vi "Lab Panel V2.6.vi"() -> ()   [LabVIEW 2013]
uses:
  <vilib>/Platform/TimedLoop/XDataNode/timing_clust.ctl
  <vilib>/Platform/TimedLoop/XDataNode/nitl_modes.ctl
  <vilib>/Platform/TimedLoop/XDataNode/wakeup.ctl
  <vilib>/platform/TimedLoop/XDataNode/XDataNode.xnode
  <vilib>/Platform/TimedLoop/XDataNode/XDNodeRunTimeDep.lvlib
panel:
  out "TEMP update":bool
  out "AI update":bool
  in  "stop":bool
  in  "Tab Control 2":T1(tab)
  out "LAB05-2 (SIG)":T2 {"PF" format="%.2f"; "AMPS" format="%.1f"}
  out "LAB05-1 (SIG)":T2 {"PF" format="%.2f"; "AMPS" format="%.1f"}
  out "LAB04-2 (SIG)":T2 {"PF" format="%.2f"; "AMPS" format="%.1f"}
  out "LAB04-1 (SIG)":T2 {"PF" format="%.2f"; "AMPS" format="%.1f"}
  out "LAB03-2 (SIG)":T2 {"PF" format="%.2f"; "AMPS" format="%.1f"}
  out "LAB03-1 (SIG)":T2 {"PF" format="%.2f"; "AMPS" format="%.1f"}
  out "LAB02-2 (SIG)":T2 {"PF" format="%.2f"; "AMPS" format="%.1f"}
  in  "LAB01-1RUN":bool
  in  "LAB05-1 (O/I)":bool
  in  "LAB05-2 (O/I)":bool
  in  "LAB04-1 (O/I)":bool
  in  "LAB04-2 (O/I)":bool
  in  "LAB02-1 (O/I)":bool
  in  "LAB02-2 (O/I)":bool
  in  "LAB01-2 (O/I)":bool
  in  "LAB01-1 (O/I)":bool
  in  "LAB03-1 (O/I)":bool
  in  "LAB05-2 RUN":bool
  in  "LAB05-1 RUN":bool
  in  "LAB04-2 RUN":bool
  in  "LAB04-1 RUN":bool
  in  "LAB03-2 RUN":bool
  in  "LAB03-1 RUN":bool
  in  "LAB02-2 RUN":bool
  in  "LAB02-1 RUN":bool
  in  "LAB01-2 RUN":bool
  in  "LAB05-2 SELECT":T3(radio)
  in  "LAB05-1 SELECT":T3(radio)
  in  "LAB04-2 SELECT":T3(radio)
  in  "LAB04-1 SELECT":T3(radio)
  in  "LAB03-2 SELECT":T3(radio)
  in  "LAB03-1 SELECT":T3(radio)
  in  "LAB02-2 SELECT":T3(radio)
  in  "LAB02-1 SELECT":T3(radio)
  in  "LAB01-2 SELECT":T3(radio)
  in  "LAB01-1 SELECT":T3(radio)
  in  "LAB03-2 (O/I)":bool
  out "LAB01-1 (SIG)":T2 {"PF" format="%.2f"; "AMPS" format="%.1f"}
  out "LAB01-2 (SIG)":T2 {"PF" format="%.2f"; "AMPS" format="%.1f"}
  out "LAB02-1 (SIG)":T2 {"PF" format="%.2f"; "AMPS" format="%.1f"}
  out "LAB05-2 (DISP)":T4 {"MINS" format="%.2g"}
  out "LAB05-1 (DISP)":T4 {"MINS" format="%.2g"}
  out "LAB04-2 (DISP)":T4 {"MINS" format="%.2g"}
  out "LAB04-1 (DISP)":T4 {"MINS" format="%.2g"}
  out "LAB03-2 (DISP)":T4 {"MINS" format="%.2g"}
  out "LAB03-1 (DISP)":T4 {"MINS" format="%.2g"}
  in  "LAB05-2 (SET)":T5
  in  "LAB05-1 (SET)":T5
  in  "LAB04-2 (SET)":T5
  in  "LAB04-1 (SET)":T5
  in  "LAB03-2 (SET)":T5
  in  "LAB03-1 (SET)":T5
  out "LAB02-2 (DISP)":T4 {"MINS" format="%.2g"}
  out "LAB02-1 (DISP)":T4 {"MINS" format="%.2g"}
  in  "LAB02-2 (SET)":T5
  in  "LAB02-1 (SET)":T5
  out "LAB05-2 (RESULT)":bool
  out "LAB05-1 (RESULT)":bool
  out "LAB04-2 (RESULT)":bool
  out "LAB04-1 (RESULT)":bool
  out "LAB03-2 (RESULT)":bool
  out "LAB03-1 (RESULT)":bool
  out "LAB02-2 (RESULT)":bool
  out "LAB02-1 (RESULT)":bool
  out "LAB01-2 (RESULT)":bool
  out "LAB01-1 (RESULT)":bool
  in  "LAB01-1 (SET)":T5
  in  "LAB01-2(SET)":T5
  out "LAB01-1 (DISP)":T4 {"MINS" format="%.2g"}
  out "LAB01-2 (DISP)":T4 {"MINS" format="%.2f"}
  out "LAB05-2 (TEMP START)":cluster{"TL":dbl, "TN":dbl}
  out "LAB04-2 (TEMP START)":cluster{"TL":dbl, "TN":dbl}
  out "LAB03-2 (TEMP START)":cluster{"TL":dbl, "TN":dbl}
  out "LAB02-2 (TEMP START)":cluster{"TL":dbl, "TN":dbl}
  out "LAB01-2 (TEMP START)":cluster{"TL":dbl, "TN":dbl}
  out "LAB05-1 (TEMP START)":cluster{"TL":dbl, "TN":dbl}
  out "LAB04-1 (TEMP START)":cluster{"TL":dbl, "TN":dbl}
  out "LAB03-1 (TEMP START)":cluster{"TL":dbl, "TN":dbl}
  out "LAB02-1 (TEMP START)":cluster{"TL":dbl, "TN":dbl}
  out "LAB01-1 (TEMP START)":cluster{"TL":dbl, "TN":dbl}
  in  "JIG ON TIME (S)":dbl=1.0 min=1.0 max=10.0 step=0.5 format="%.1g"
  in  "JIG OFF TIME (S)":dbl=2.0 min=2.0 max=10.0 step=0.5 format="%.1g"
  out "LAB01-1 (JIG)":bool
  out "LAB01-2 (JIG)":bool
  out "LAB02-1 (JIG)":bool
  out "LAB02-2 (JIG)":bool
  out "LAB03-1 (JIG)":bool
  out "LAB03-2 (JIG)":bool
  out "LAB04-1 (JIG)":bool
  out "LAB04-2 (JIG)":bool
  out "LAB05-1 (JIG)":bool
  out "LAB05-2 (JIG)":bool
  out "LAB01 (CAL)":T6 {"2 (TN) cal" min=0.0 step=0.01 format="%.2f"; "2 (TL) cal" min=0.0 step=0.01 format="%.2f"; "2 (PF) cal" min=0.0 step=0.01 format="%.2f"; "2 (V) cal" min=0.0 step=0.01 format="%.2f"; "2 (A) cal" min=0.0 step=0.01 format="%.2f"; "1 (TN) cal" min=0.0 step=0.01 format="%.2f"; "1 (TL) cal" min=0.0 step=0.01 format="%.2f"; "1 (PF) cal" min=0.0 step=0.01 format="%.2f"; "1 (V) cal" min=0.0 step=0.01 format="%.2f"; "1  (A) cal" min=0.0 step=0.01 format="%.2f"}
  out "LAB03 (CAL)":T6 {"2 (TN) cal" min=0.0 step=0.01 format="%.2f"; "2 (TL) cal" min=0.0 step=0.01 format="%.2f"; "2 (PF) cal" min=0.0 step=0.01 format="%.2f"; "2 (V) cal" min=0.0 step=0.01 format="%.2f"; "2 (A) cal" min=0.0 step=0.01 format="%.2f"; "1 (TN) cal" min=0.0 step=0.01 format="%.2f"; "1 (TL) cal" min=0.0 step=0.01 format="%.2f"; "1 (PF) cal" min=0.0 step=0.01 format="%.2f"; "1 (V) cal" min=0.0 step=0.01 format="%.2f"; "1  (A) cal" min=0.0 step=0.01 format="%.2f"}
  out "LAB02 (CAL)":T7 {"2 (TN) cal" min=0.0 step=0.01 format="%.2f"; "2 (TL) cal" min=0.0 step=0.01 format="%.2f"; "2 (PF) cal" min=0.0 step=0.01 format="%.2f"; "2 (V) cal" min=0.0 step=0.01 format="%.2f"; "2 (A) cal" min=0.0 step=0.01 format="%.2f"; "1 (TN) cal" min=0.0 step=0.01 format="%.2f"; "1 (TL) cal" min=0.0 step=0.01 format="%.2f"; "1 (PF) cal" min=0.0 step=0.01 format="%.2f"; "1 (V) cal" min=0.0 step=0.01 format="%.2f"; "1 (A) cal" min=0.0 step=0.01 format="%.2f"}
  out "LAB05 (CAL)":T6 {"2 (TN) cal" min=0.0 step=0.01 format="%.2f"; "2 (TL) cal" min=0.0 step=0.01 format="%.2f"; "2 (PF) cal" min=0.0 step=0.01 format="%.2f"; "2 (V) cal" min=0.0 step=0.01 format="%.2f"; "2 (A) cal" min=0.0 step=0.01 format="%.2f"; "1 (TN) cal" min=0.0 step=0.01 format="%.2f"; "1 (TL) cal" min=0.0 step=0.01 format="%.2f"; "1 (PF) cal" min=0.0 step=0.01 format="%.2f"; "1 (V) cal" min=0.0 step=0.01 format="%.2f"; "1  (A) cal" min=0.0 step=0.01 format="%.2f"}
  out "LAB04 (CAL)":T6 {"2 (TN) cal" min=0.0 step=0.01 format="%.2f"; "2 (TL) cal" min=0.0 step=0.01 format="%.2f"; "2 (PF) cal" min=0.0 step=0.01 format="%.2f"; "2 (V) cal" min=0.0 step=0.01 format="%.2f"; "2 (A) cal" min=0.0 step=0.01 format="%.2f"; "1 (TN) cal" min=0.0 step=0.01 format="%.2f"; "1 (TL) cal" min=0.0 step=0.01 format="%.2f"; "1 (PF) cal" min=0.0 step=0.01 format="%.2f"; "1 (V) cal" min=0.0 step=0.01 format="%.2f"; "1  (A) cal" min=0.0 step=0.01 format="%.2f"}
  out "calibration file error out":errorcluster
  in  "CALIBRATE":bool
  in  "Amps fail level":dbl=1.0 min=1.0 max=100.0 step=1.0
  in  "Tab Control":T8(tab)
  out "LAB01-2 (GRAPH)":dynamicdata(graph)
  out "LAB01-1 (GRAPH)":dynamicdata(graph)
  out "LAB02-2 (GRAPH)":dynamicdata(graph)
  out "LAB02-1 (GRAPH)":dynamicdata(graph)
  out "LAB03-2 (GRAPH)":dynamicdata(graph)
  out "LAB03-1 (GRAPH)":dynamicdata(graph)
  out "LAB04-2 (GRAPH)":dynamicdata(graph)
  out "LAB04-1 (GRAPH)":dynamicdata(graph)
  out "LAB05-2 (GRAPH)":dynamicdata(graph)
  out "LAB05-1 (GRAPH)":dynamicdata(graph)
  out "LAB05 TEMP":T9
  out "LAB04 TEMP":T9
  out "LAB02 TEMP":T9
  out "LAB01 TEMP":T9
  out "LAB03 TEMP":T9
  out "Analog Error Array":errorcluster[](array[cluster])
  out "AI loop time":dbl format="%.6g"
  out "loops":dbl
  in  "loop  delay(mS)":dbl
  out "on loops":dbl
  out "off loops":dbl
  out "jig cycle":dbl
  out "LAB01-1 (TDMS)":refnum<k34>
  out "data file error":errorcluster
  out "LAB02-1 (TDMS)":refnum<k34>
  out "LAB01-2 (TDMS)":refnum<k34>
  out "LAB02-2 (TDMS)":refnum<k34>
  out "LAB03-1 (TDMS)":refnum<k34>
  out "LAB03-2 (TDMS)":refnum<k34>
  out "LAB04-1 (TDMS)":refnum<k34>
  out "LAB04-2 (TDMS)":refnum<k34>
  out "LAB05-1 (TDMS)":refnum<k34>
  out "LAB05-2 (TDMS)":refnum<k34>
  # "LAB01"
  # "LAB02"
  # "LAB05"
  # "LAB03"
  # "LAB04"
  # "LAB01"
  # "LAB02"
  # "LAB03"
  # "LAB04"
  # "LAB05"
  # "JIG SET"
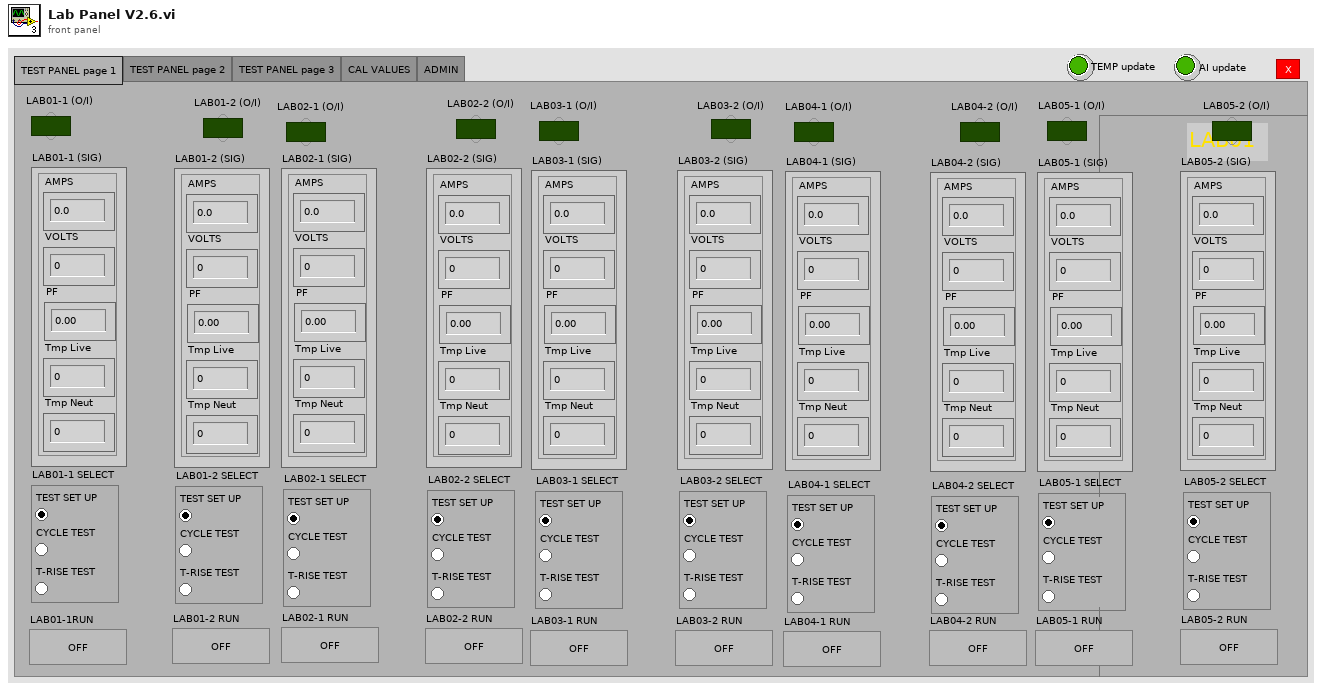
[diagram p1: front panel]
types:
  T1 = enum32{"TEST PANEL page 1", "TEST PANEL page 2", "TEST PANEL page 3", "CAL VALUES", "ADMIN"}
  T2 = cluster{"AMPS":dbl, "VOLTS":dbl, "PF":dbl, "Tmp Live":dbl, "Tmp Neut":dbl}
  T3 = enum32{"TEST SET UP", "CYCLE TEST", "T-RISE TEST"}
  T4 = cluster{"CYCLE":dbl, "MINS":dbl, "STATUS":string}
  T5 = cluster{"NAME":string, "DESCRIPTION":string, "CYCLES":dbl, "T-RISE mins":dbl, "T-RISE deg C":dbl}
  T6 = cluster{"1  (A) cal":dbl, "1 (V) cal":dbl, "1 (PF) cal":dbl, "1 (TL) cal":dbl, "1 (TN) cal":dbl, "2 (A) cal":dbl, "2 (V) cal":dbl, "2 (PF) cal":dbl, "2 (TL) cal":dbl, "2 (TN) cal":dbl}
  T7 = cluster{"1 (A) cal":dbl, "1 (V) cal":dbl, "1 (PF) cal":dbl, "1 (TL) cal":dbl, "1 (TN) cal":dbl, "2 (A) cal":dbl, "2 (V) cal":dbl, "2 (PF) cal":dbl, "2 (TL) cal":dbl, "2 (TN) cal":dbl}
  T8 = enum32{"LAB01", "LAB02", "LAB03", "LAB04", "LAB05", "TEMPERATURE", "ERROR"}
  T9 = cluster{"T1 Live":dbl, "T1 Neut":dbl, "T2 Live":dbl, "T2 Neut":dbl, "ID":dbl, "ER":dbl}
  T10 = typedef "XDNodeRunTimeDep.lvlib/timing_clust.ctl" = cluster{"Expected End [f-1]":u64, "Actual End [f-1]":u64, "Finished Late? [f-1]":bool, "Expected End [i-1]":u64, "Actual End [i-1]":u64, "Finished Late? [i-1]":bool, "Expected Start [i]":u64, "Actual Start [i]":u64, "Expected Start [f]":u64, "Actual Start [f]":u64, "Source Name":string, "Structure Name":string, "Period":i64, "Deadline":i64, "Offset":i64, "Start":i64, "Priority":i32, "Timeout":i32, "Mode":T11, "Wakeup Reason":T12, "Error":errorcluster, "Source Type":string, "Secondary Source Type":string, "Global End Time":u64, "Global Start Time":u64, "Frame Duration":u64, "Iteration Duration":u64, "Assigned CPU":i32, "I/O Scan Engine Mode":u32}
  T11 = typedef "XDNodeRunTimeDep.lvlib/nitl_modes.ctl" = enum32{"No Change", "Process missed periods, maintain original phase", "Discard missed periods, maintain original phase", "Process missed periods, ignore original phase", "Discard missed periods, ignore original phase"}
  T12 = typedef "XDNodeRunTimeDep.lvlib/wakeup.ctl" = enum32{"Normal", "Aborted", "Asynchronous wakeup", "Timing source error", "Timed loop error", "Timeout"}
  T13 = enum16{"open", "open or create", "create or replace", "create", "open (read-only)"}
  T14 = cluster{"T1":dbl, "T2":dbl, "T3":dbl, "T4":dbl, "ID":dbl, "ER":dbl}
  T15 = cluster{"LAB01-1 (A)":dbl, "LAB01-1 (V)":dbl, "LAB01-1 (PF)":dbl, "LAB01-2 (A)":dbl, "LAB01-2 (V)":dbl, "LAB01-2 (PF)":dbl}
  T16 = cluster{"LAB02-1 (A)":dbl, "LAB02-1 (V)":dbl, "LAB02-1 (PF)":dbl, "LAB02-2 (A)":dbl, "LAB02-2 (V)":dbl, "LAB02-2 (PF)":dbl}
  T17 = cluster{"LAB03-1 (A)":dbl, "LAB03-1 (V)":dbl, "LAB03-1 (PF)":dbl, "LAB03-2 (A)":dbl, "LAB03-2 (V)":dbl, "LAB03-2 (PF)":dbl}
  T18 = cluster{"LAB04-1 (A)":dbl, "LAB04-1 (V)":dbl, "LAB04-1 (PF)":dbl, "LAB04-2 (A)":dbl, "LAB04-2 (V)":dbl, "LAB04-2 (PF)":dbl}
  T19 = cluster{"LAB05-1 (A)":dbl, "LAB05-1 (V)":dbl, "LAB05-1 (PF)":dbl, "LAB05-2 (A)":dbl, "LAB05-2 (V)":dbl, "LAB05-2 (PF)":dbl}
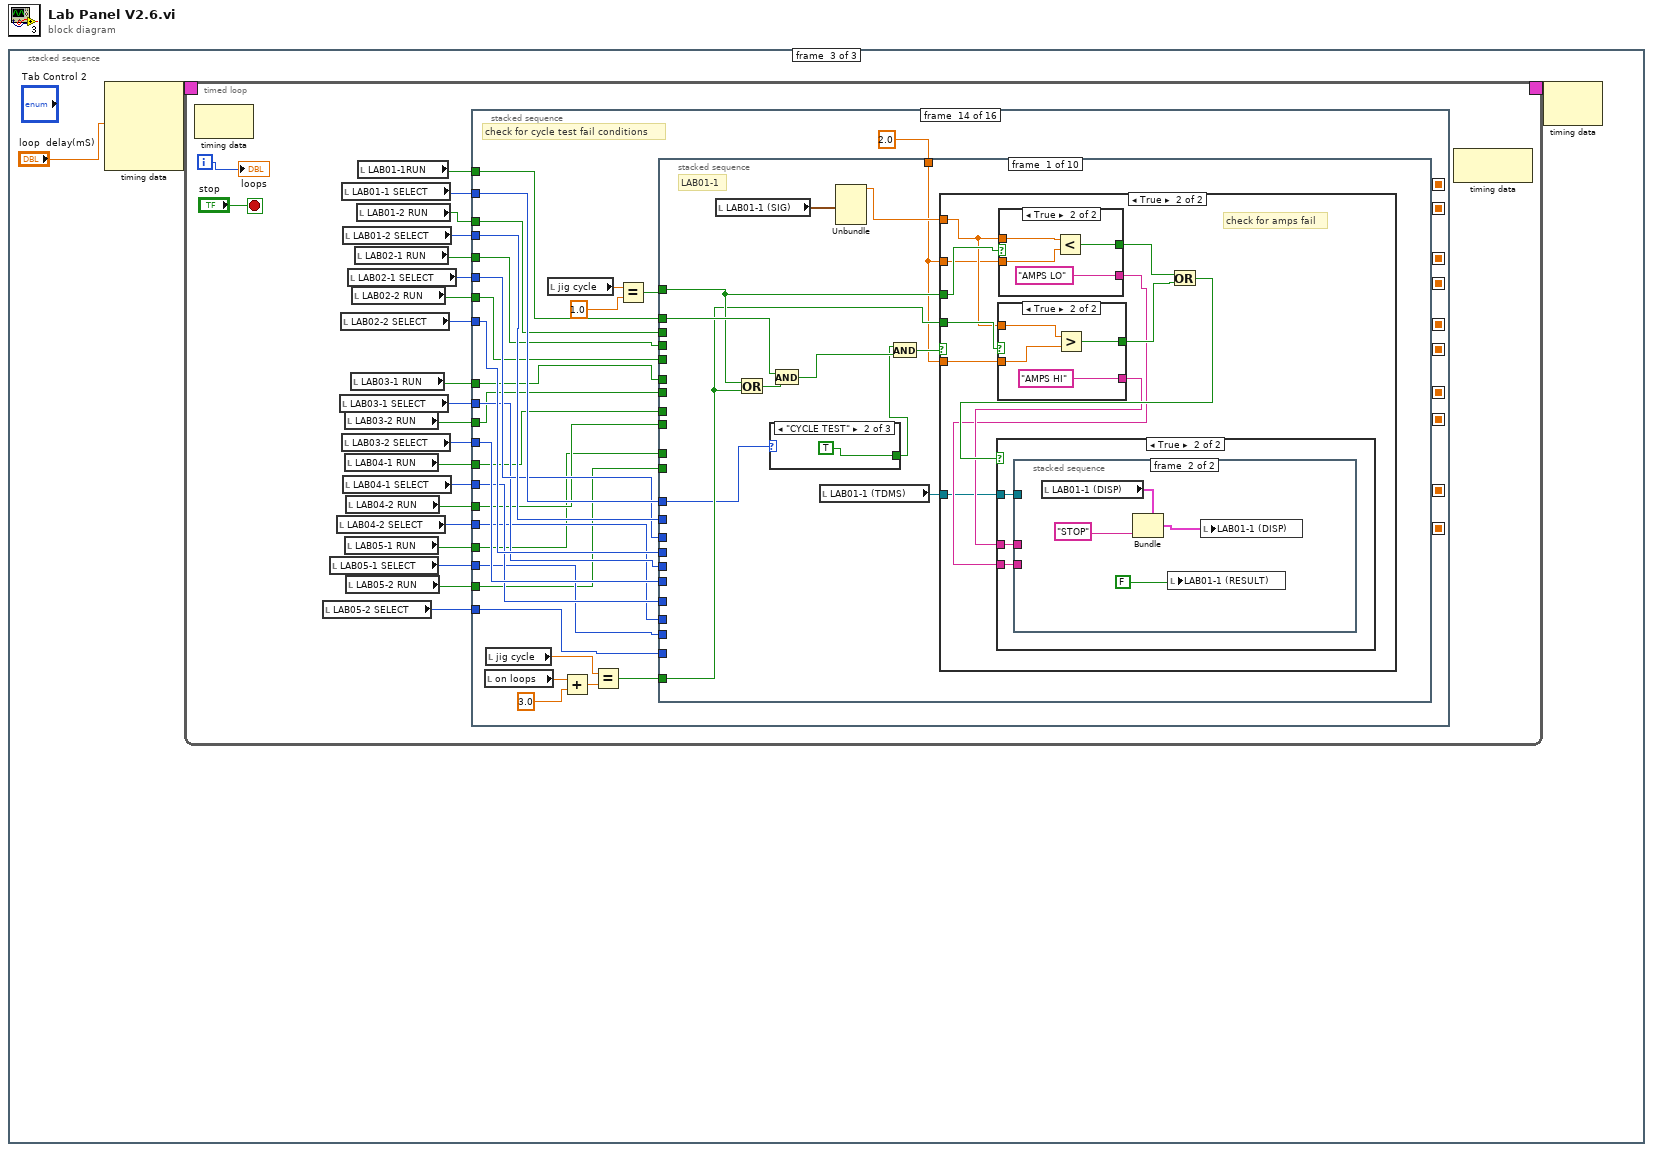
[diagram p0: block diagram]
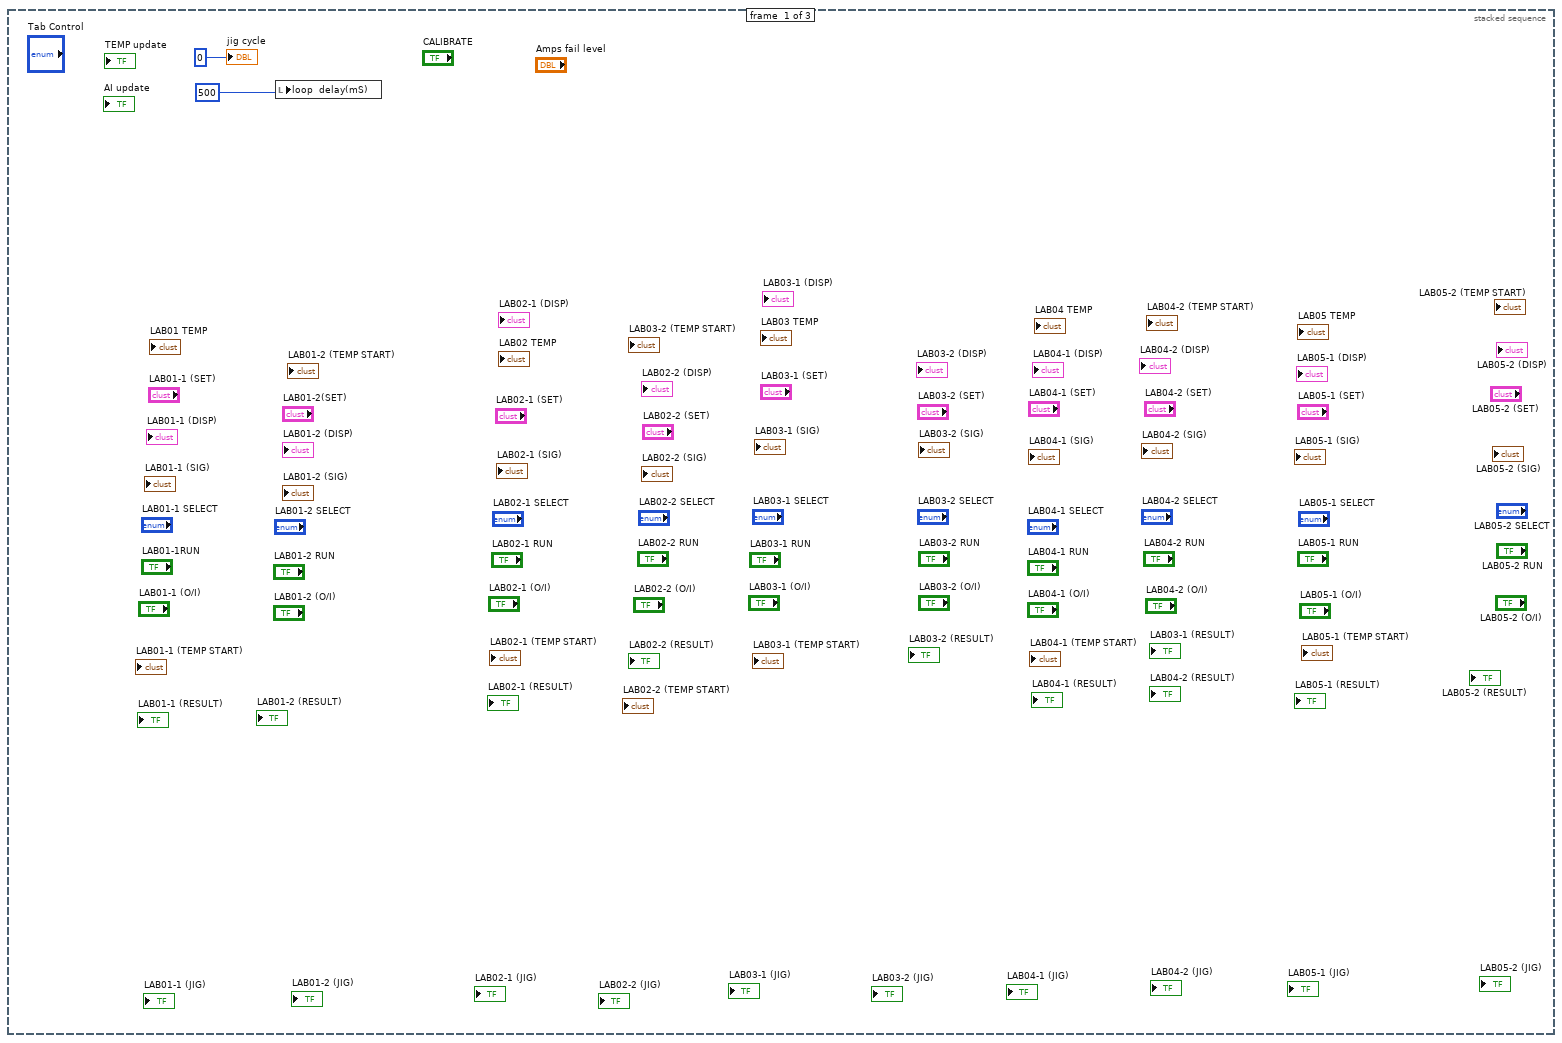
[diagram p2: hidden frame]
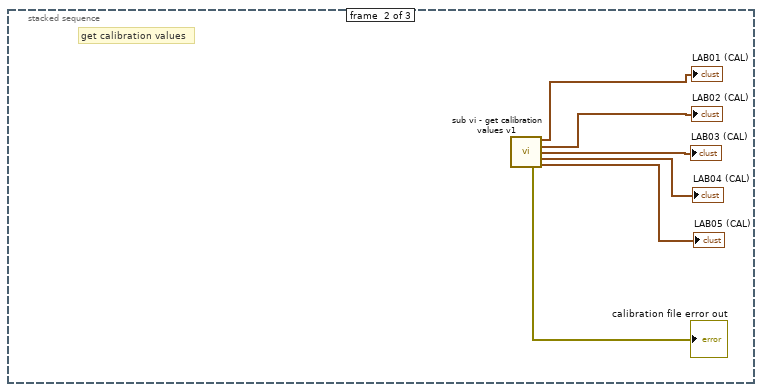
[diagram p3: hidden frame]
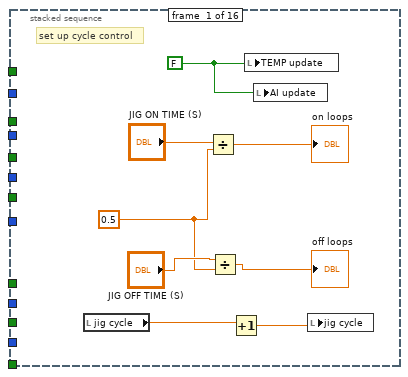
[diagram p4: hidden frame]
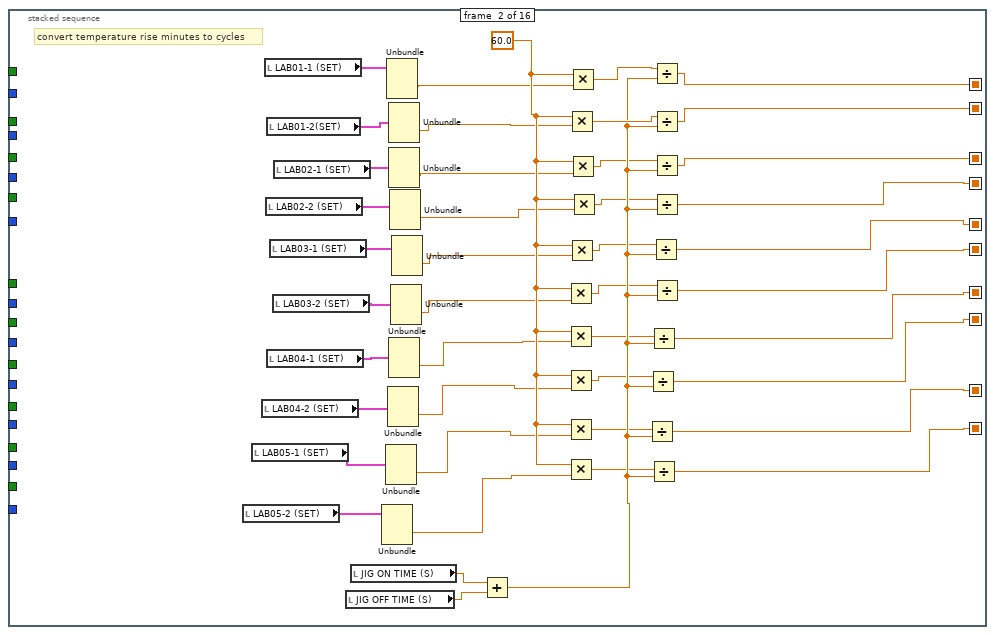
[diagram p5: hidden frame]
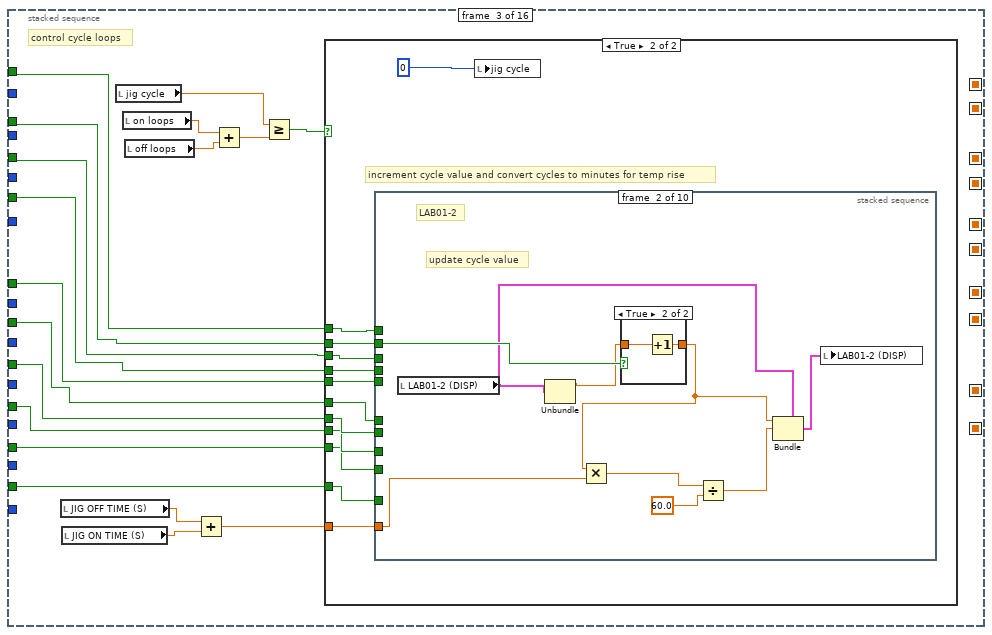
[diagram p6: hidden frame]
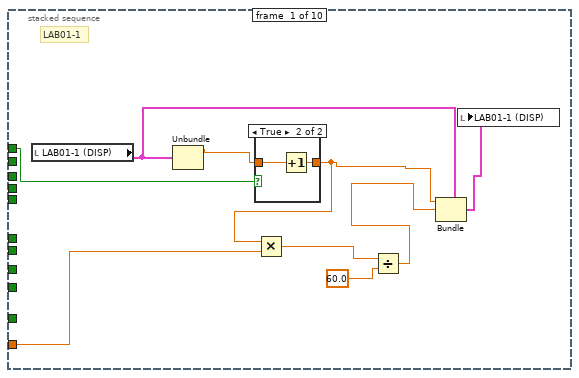
[diagram p8: hidden frame]
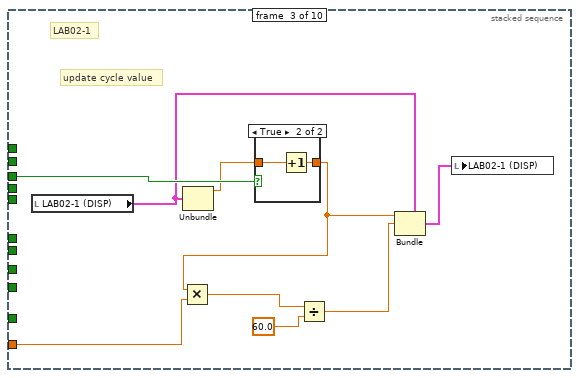
[diagram p11: hidden frame]
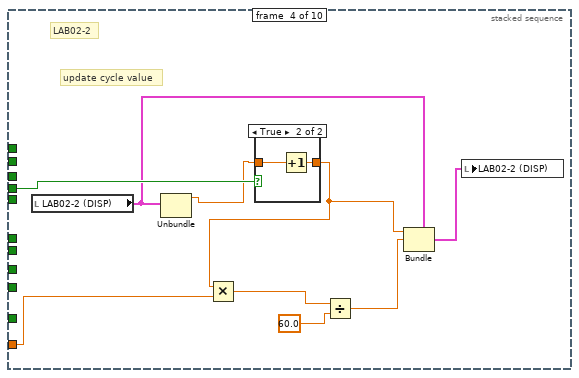
[diagram p13: hidden frame]
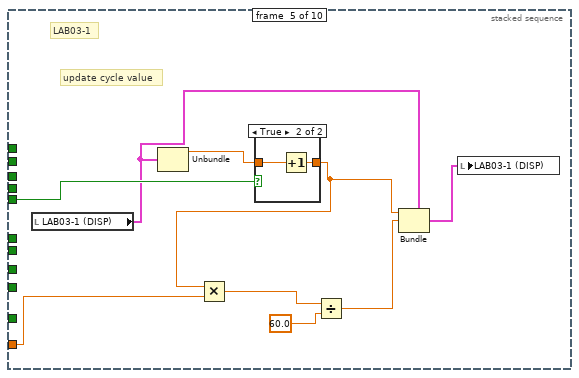
[diagram p15: hidden frame]
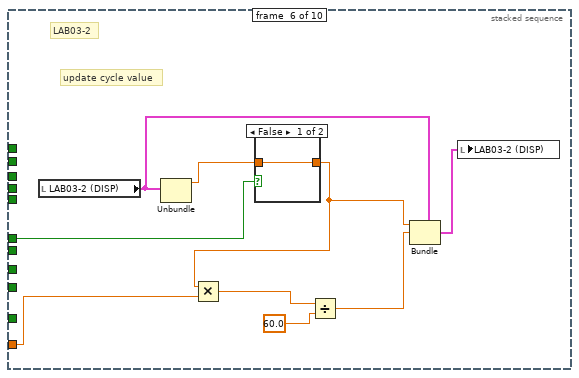
[diagram p17: hidden frame]
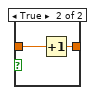
[diagram p18: hidden frame]
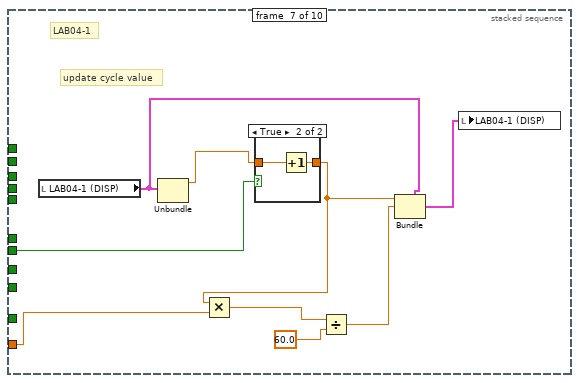
[diagram p19: hidden frame]
diagram:
  n1 = stacked-sequence {
    frame #0 {
      n2 = local write "loop  delay(mS)"(500) -> ()
      "jig cycle" <- 0
    }
    frame #1 {
      # "get calibration values"
      n3 = call "sub vi - get calibration values v1.vi"() -> ("LAB01 (CAL)"=→"LAB01 (CAL)":T6, "LAB02 (CAL)"=→"LAB02 (CAL)":T7, "LAB03 (CAL)"=→"LAB03 (CAL)":T6, "LAB04 (CAL)"=→"LAB04 (CAL)":T6, "calibration file error out"=→"calibration file error out":errorcluster, "LAB05 (CAL)"=→"LAB05 (CAL)":T6)  [unwired: 10 in]
    }
    frame #2 {
      n4 = node-c288("loop  delay(mS)") -> (w11:T10)  [unwired: 3 in]
      n5 = timed-loop {
        timing: w11 -> [_]
        timing-out: [_] -> w10
        i -> [w33]
        stop <- "stop" stop-if-true
        n6 = node-c288() -> ()  [unwired: 1 in, 1 out]
        n7 = local read "LAB05-2 SELECT"() -> (w12:T3)
        n8 = local read "LAB05-1 SELECT"() -> (w13:T3)
        n9 = local read "LAB04-2 SELECT"() -> (w14:T3)
        n10 = local read "LAB03-1 SELECT"() -> (w17:T3)
        n11 = local read "LAB02-2 SELECT"() -> (w18:T3)
        n12 = local read "LAB01-1 SELECT"() -> (w21:T3)
        n13 = local read "LAB03-2 SELECT"() -> (w16:T3)
        n14 = local read "LAB01-2 SELECT"() -> (w20:T3)
        n15 = local read "LAB04-1 SELECT"() -> (w15:T3)
        n16 = local read "LAB03-2 RUN"() -> (w26:bool)
        n17 = local read "LAB04-1 RUN"() -> (w25:bool)
        n18 = local read "LAB05-1 RUN"() -> (w23:bool)
        n19 = local read "LAB04-2 RUN"() -> (w24:bool)
        n20 = local read "LAB05-2 RUN"() -> (w22:bool)
        n21 = local read "LAB02-1 SELECT"() -> (w19:T3)
        n22 = local read "LAB03-1 RUN"() -> (w27:bool)
        n23 = local read "LAB02-2 RUN"() -> (w28:bool)
        n24 = local read "LAB02-1 RUN"() -> (w29:bool)
        n25 = local read "LAB01-2 RUN"() -> (w30:bool)
        n26 = local read "LAB01-1RUN"() -> (w31:bool)
        n27 = stacked-sequence {
          seq-local: [_ w85 _ _ _ _ _ _ _ _ _ _ _ _ _ _] -> [_ _ _ _ _ w1464 _ _ _ _ _ _ _ _ _ _]
          seq-local: [_ w84 _ _ _ _ _ _ _ _ _ _ _ _ _ _] -> [_ _ _ _ _ _ _ _ _ _ _ _ _ _ _ _]
          seq-local: [_ w71 _ _ _ _ _ _ _ _ _ _ _ _ _ _] -> [_ _ _ _ _ _ _ _ _ _ _ _ _ _ _ _]
          seq-local: [_ w70 _ _ _ _ _ _ _ _ _ _ _ _ _ _] -> [_ _ _ _ _ _ _ _ _ _ _ _ _ _ _ _]
          seq-local: [_ w69 _ _ _ _ _ _ _ _ _ _ _ _ _ _] -> [_ _ _ _ _ _ _ _ _ _ _ _ _ _ _ _]
          seq-local: [_ w68 _ _ _ _ _ _ _ _ _ _ _ _ _ _] -> [_ _ _ _ _ _ _ _ _ _ _ _ _ _ _ _]
          seq-local: [_ w67 _ _ _ _ _ _ _ _ _ _ _ _ _ _] -> [_ _ _ _ _ _ _ _ _ _ _ _ _ _ _ _]
          seq-local: [_ w66 _ _ _ _ _ _ _ _ _ _ _ _ _ _] -> [_ _ _ _ _ _ _ _ _ _ _ _ _ _ _ _]
          seq-local: [_ w65 _ _ _ _ _ _ _ _ _ _ _ _ _ _] -> [_ _ _ _ _ _ _ _ _ _ _ _ _ _ _ _]
          seq-local: [_ w64 _ _ _ _ _ _ _ _ _ _ _ _ _ _] -> [_ _ _ _ _ _ _ _ _ _ _ _ _ _ _ _]
          tunnel: w31 -> [_ _ w101 w257 w1064 w1475 w1785 _ _ _ _ _ w2350 w2839 w3378 _]
          tunnel: w30 -> [_ _ w100 w255 w1063 w1474 w1784 _ _ _ _ _ w2349 w2837 w3368 _]
          tunnel: w29 -> [_ _ w99 w253 w1062 w1473 w1783 _ _ _ _ _ w2348 w2835 w3367 _]
          tunnel: w28 -> [_ _ w98 w251 w1061 w1472 w1782 _ _ _ _ _ w2347 w2833 w3366 _]
          tunnel: w27 -> [_ _ w97 w249 w1060 w1471 w1781 _ _ _ _ _ w2346 w2831 w3365 _]
          tunnel: w26 -> [_ _ w96 w247 w1059 w1470 w1780 _ _ _ _ _ w2345 w2829 w3364 _]
          tunnel: w25 -> [_ _ w95 w245 w1058 w1469 w1779 _ _ _ _ _ w2344 w2827 w3360 _]
          tunnel: w24 -> [_ _ w94 w243 w1057 w1468 w1778 _ _ _ _ _ w2343 w2825 w3363 _]
          tunnel: w23 -> [_ _ w93 w241 w1056 w1467 w1777 _ _ _ _ _ w2342 w2823 w3362 _]
          tunnel: w22 -> [_ _ w92 w239 w1055 w1466 w1776 _ _ _ _ _ w2341 w2821 w3361 _]
          tunnel: w21 -> [_ _ _ w256 w1054 w1465 _ _ _ _ _ _ _ w2841 w3379 _]
          tunnel: w20 -> [_ _ _ w254 w1053 w1463 _ _ _ _ _ _ _ w2836 w3377 _]
          tunnel: w19 -> [_ _ _ w252 w1052 w1462 _ _ _ _ _ _ _ w2834 w3376 _]
          tunnel: w18 -> [_ _ _ w250 w1051 w1461 _ _ _ _ _ _ _ w2832 w3375 _]
          tunnel: w17 -> [_ _ _ w248 w1050 w1460 _ _ _ _ _ _ _ w2830 w3374 _]
          tunnel: w16 -> [_ _ _ w246 w1049 w1459 _ _ _ _ _ _ _ w2828 w3373 _]
          tunnel: w15 -> [_ _ _ w244 w1048 w1458 _ _ _ _ _ _ _ w2826 w3372 _]
          tunnel: w14 -> [_ _ _ w242 w1047 w1457 _ _ _ _ _ _ _ w2824 w3371 _]
          tunnel: w13 -> [_ _ _ w240 w1046 w1456 _ _ _ _ _ _ _ w2822 w3370 _]
          tunnel: w12 -> [_ _ _ w238 w1045 w1455 _ _ _ _ _ _ _ w2820 w3369 _]
          frame #0 {
            w36 = FALSE
            w41 = 0.5
            # "set up cycle control"
            n28 = local read "jig cycle"() -> (w40:dbl)
            n29 = Divide(x="JIG ON TIME (S)", y=w41) -> (x/y=→"on loops":dbl)
            n30 = Divide(x="JIG OFF TIME (S)", y=w41) -> (x/y=→"off loops":dbl)
            n31 = Increment(x=w40) -> (x+1=w39:dbl)
            n32 = local write "TEMP update"(w36) -> ()
            n33 = local write "AI update"(w36) -> ()
            n34 = local write "jig cycle"(w39) -> ()
          }
          frame #1 {
            w81 = 60.0
            # "convert temperature rise minutes to cycles"
            n35 = local read "LAB05-2 (SET)"() -> (w45:T5)
            n36 = local read "LAB05-1 (SET)"() -> (w47:T5)
            n37 = local read "LAB04-2 (SET)"() -> (w49:T5)
            n38 = local read "LAB01-1 (SET)"() -> (w63:T5)
            n39 = local read "LAB02-2 (SET)"() -> (w57:T5)
            n40 = local read "LAB01-2(SET)"() -> (w61:T5)
            n41 = local read "LAB04-1 (SET)"() -> (w51:T5)
            n42 = local read "LAB03-1 (SET)"() -> (w55:T5)
            n43 = local read "LAB03-2 (SET)"() -> (w53:T5)
            n44 = local read "LAB02-1 (SET)"() -> (w59:T5)
            n45 = local read "JIG OFF TIME (S)"() -> (w86:dbl)
            n46 = local read "JIG ON TIME (S)"() -> (w87:dbl)
            n47 = Unbundle(w45) -> ("T-RISE mins"=w44:dbl)  [unwired: 4 out]
            n48 = Unbundle(w47) -> ("T-RISE mins"=w46:dbl)  [unwired: 4 out]
            n49 = Unbundle(w63) -> ("T-RISE mins"=w62:dbl)  [unwired: 4 out]
            n50 = Unbundle(w49) -> ("T-RISE mins"=w48:dbl)  [unwired: 4 out]
            n51 = Unbundle(w61) -> ("T-RISE mins"=w60:dbl)  [unwired: 4 out]
            n52 = Unbundle(w59) -> ("T-RISE mins"=w58:dbl)  [unwired: 4 out]
            n53 = Unbundle(w51) -> ("T-RISE mins"=w50:dbl)  [unwired: 4 out]
            n54 = Unbundle(w57) -> ("T-RISE mins"=w56:dbl)  [unwired: 4 out]
            n55 = Unbundle(w53) -> ("T-RISE mins"=w52:dbl)  [unwired: 4 out]
            n56 = Unbundle(w55) -> ("T-RISE mins"=w54:dbl)  [unwired: 4 out]
            n57 = Add(x=w87, y=w86) -> (x+y=w80:dbl)
            n58 = Multiply(x=w81, y=w52) -> (x*y=w76:dbl)
            n59 = Multiply(x=w81, y=w50) -> (x*y=w75:dbl)
            n60 = Multiply(x=w81, y=w48) -> (x*y=w74:dbl)
            n61 = Multiply(x=w81, y=w46) -> (x*y=w73:dbl)
            n62 = Multiply(x=w81, y=w44) -> (x*y=w72:dbl)
            n63 = Multiply(x=w81, y=w60) -> (x*y=w82:dbl)
            n64 = Multiply(x=w81, y=w54) -> (x*y=w77:dbl)
            n65 = Multiply(x=w81, y=w62) -> (x*y=w83:dbl)
            n66 = Multiply(x=w81, y=w58) -> (x*y=w79:dbl)
            n67 = Multiply(x=w81, y=w56) -> (x*y=w78:dbl)
            n68 = Divide(x=w73, y=w80) -> (x/y=w65:dbl)
            n69 = Divide(x=w74, y=w80) -> (x/y=w66:dbl)
            n70 = Divide(x=w75, y=w80) -> (x/y=w67:dbl)
            n71 = Divide(x=w72, y=w80) -> (x/y=w64:dbl)
            n72 = Divide(x=w77, y=w80) -> (x/y=w69:dbl)
            n73 = Divide(x=w83, y=w80) -> (x/y=w85:dbl)
            n74 = Divide(x=w82, y=w80) -> (x/y=w84:dbl)
            n75 = Divide(x=w79, y=w80) -> (x/y=w71:dbl)
            n76 = Divide(x=w78, y=w80) -> (x/y=w70:dbl)
            n77 = Divide(x=w76, y=w80) -> (x/y=w68:dbl)
          }
          frame #2 {
            # "control cycle loops"
            n78 = local read "JIG OFF TIME (S)"() -> (w90:dbl)
            n79 = local read "JIG ON TIME (S)"() -> (w89:dbl)
            n80 = local read "jig cycle"() -> (w103:dbl)
            n81 = local read "on loops"() -> (w105:dbl)
            n82 = local read "off loops"() -> (w104:dbl)
            n83 = Add(x=w90, y=w89) -> (x+y=w88:dbl)
            n84 = Add(x=w105, y=w104) -> (x+y=w91:dbl)
            n85 = Greater Or Equal?(x=w103, y=w91) -> (x >= y?=w102:bool)
            n86 = case shown="True" w102 {
              tunnel: w101 -> [_ w116]
              tunnel: w100 -> [_ w115]
              tunnel: w99 -> [_ w114]
              tunnel: w98 -> [_ w113]
              tunnel: w97 -> [_ w112]
              tunnel: w96 -> [_ w111]
              tunnel: w95 -> [_ w110]
              tunnel: w94 -> [_ w109]
              tunnel: w93 -> [_ w108]
              tunnel: w92 -> [_ w107]
              tunnel: w88 -> [_ w106]
              frame False {
              }
              frame True {
                # "increment cycle value and convert cycles to minutes for temp rise"
                n87 = stacked-sequence {
                  tunnel: w116 -> [w126 _ _ _ _ _ _ _ _ _]
                  tunnel: w115 -> [_ w138 _ _ _ _ _ _ _ _]
                  tunnel: w114 -> [_ _ w150 _ _ _ _ _ _ _]
                  tunnel: w113 -> [_ _ _ w162 _ _ _ _ _ _]
                  tunnel: w112 -> [_ _ _ _ w174 _ _ _ _ _]
                  tunnel: w111 -> [_ _ _ _ _ w186 _ _ _ _]
                  tunnel: w110 -> [_ _ _ _ _ _ w198 _ _ _]
                  tunnel: w109 -> [_ _ _ _ _ _ _ w210 _ _]
                  tunnel: w108 -> [_ _ _ _ _ _ _ _ w222 _]
                  tunnel: w107 -> [_ _ _ _ _ _ _ _ _ w234]
                  tunnel: w106 -> [w123 w135 w147 w159 w171 w183 w195 w207 w219 w231]
                  frame #0 {
                    # "LAB01-1"
                    n88 = local read "LAB01-1 (DISP)"() -> (w121:T4)
                    n89 = Unbundle(w121) -> ("CYCLE"=w122:dbl)  [unwired: 2 out]
                    n90 = case shown="True" w126 {
                      tunnel: w122 -> [w127 w129]
                      tunnel: [w127 w128] -> w120
                      frame False {
                      }
                      frame True {
                        n91 = Increment(x=w129) -> (x+1=w128:dbl)
                      }
                    }
                    n92 = Multiply(x=w120, y=w123) -> (x*y=w124:dbl)
                    n93 = Divide(x=w124, y=60.0) -> (x/y=w119:dbl)
                    n94 = Bundle(cluster=w121, "CYCLE"=w120, "MINS"=w119) -> (w118:T4)  [unwired: 1 in]
                    n95 = local write "LAB01-1 (DISP)"(w118) -> ()
                  }
                  frame #1 {
                    # "update cycle value"
                    # "LAB01-2"
                    n96 = local read "LAB01-2 (DISP)"() -> (w133:T4)
                    n97 = Unbundle(w133) -> ("CYCLE"=w134:dbl)  [unwired: 2 out]
                    n98 = case shown="True" w138 {
                      tunnel: w134 -> [w139 w141]
                      tunnel: [w139 w140] -> w131
                      frame False {
                      }
                      frame True {
                        n99 = Increment(x=w141) -> (x+1=w140:dbl)
                      }
                    }
                    n100 = Multiply(x=w131, y=w135) -> (x*y=w136:dbl)
                    n101 = Divide(x=w136, y=60.0) -> (x/y=w130:dbl)
                    n102 = Bundle(cluster=w133, "CYCLE"=w131, "MINS"=w130) -> (w132:T4)  [unwired: 1 in]
                    n103 = local write "LAB01-2 (DISP)"(w132) -> ()
                  }
                  frame #2 {
                    # "update cycle value"
                    # "LAB02-1"
                    n104 = local read "LAB02-1 (DISP)"() -> (w145:T4)
                    n105 = Unbundle(w145) -> ("CYCLE"=w146:dbl)  [unwired: 2 out]
                    n106 = case shown="True" w150 {
                      tunnel: [w151 w153] -> w143
                      tunnel: w146 -> [w151 w152]
                      frame False {
                      }
                      frame True {
                        n107 = Increment(x=w152) -> (x+1=w153:dbl)
                      }
                    }
                    n108 = Multiply(x=w143, y=w147) -> (x*y=w148:dbl)
                    n109 = Divide(x=w148, y=60.0) -> (x/y=w142:dbl)
                    n110 = Bundle(cluster=w145, "CYCLE"=w143, "MINS"=w142) -> (w144:T4)  [unwired: 1 in]
                    n111 = local write "LAB02-1 (DISP)"(w144) -> ()
                  }
                  frame #3 {
                    # "update cycle value"
                    # "LAB02-2"
                    n112 = local read "LAB02-2 (DISP)"() -> (w157:T4)
                    n113 = Unbundle(w157) -> ("CYCLE"=w158:dbl)  [unwired: 2 out]
                    n114 = case shown="True" w162 {
                      tunnel: [w163 w165] -> w156
                      tunnel: w158 -> [w163 w164]
                      frame False {
                      }
                      frame True {
                        n115 = Increment(x=w164) -> (x+1=w165:dbl)
                      }
                    }
                    n116 = Multiply(x=w156, y=w159) -> (x*y=w160:dbl)
                    n117 = Divide(x=w160, y=60.0) -> (x/y=w155:dbl)
                    n118 = Bundle(cluster=w157, "CYCLE"=w156, "MINS"=w155) -> (w154:T4)  [unwired: 1 in]
                    n119 = local write "LAB02-2 (DISP)"(w154) -> ()
                  }
                  frame #4 {
                    # "update cycle value"
                    # "LAB03-1"
                    n120 = local read "LAB03-1 (DISP)"() -> (w169:T4)
                    n121 = Unbundle(w169) -> ("CYCLE"=w170:dbl)  [unwired: 2 out]
                    n122 = case shown="True" w174 {
                      tunnel: [w175 w177] -> w166
                      tunnel: w170 -> [w175 w176]
                      frame False {
                      }
                      frame True {
                        n123 = Increment(x=w176) -> (x+1=w177:dbl)
                      }
                    }
                    n124 = Multiply(x=w166, y=w171) -> (x*y=w172:dbl)
                    n125 = Divide(x=w172, y=60.0) -> (x/y=w167:dbl)
                    n126 = Bundle(cluster=w169, "CYCLE"=w166, "MINS"=w167) -> (w168:T4)  [unwired: 1 in]
                    n127 = local write "LAB03-1 (DISP)"(w168) -> ()
                  }
                  frame #5 {
                    # "update cycle value"
                    # "LAB03-2"
                    n128 = local read "LAB03-2 (DISP)"() -> (w181:T4)
                    n129 = Unbundle(w181) -> ("CYCLE"=w182:dbl)  [unwired: 2 out]
                    n130 = case shown="False" w186 {
                      tunnel: [w187 w189] -> w180
                      tunnel: w182 -> [w187 w188]
                      frame False {
                      }
                      frame True {
                        n131 = Increment(x=w188) -> (x+1=w189:dbl)
                      }
                    }
                    n132 = Multiply(x=w180, y=w183) -> (x*y=w184:dbl)
                    n133 = Divide(x=w184, y=60.0) -> (x/y=w179:dbl)
                    n134 = Bundle(cluster=w181, "CYCLE"=w180, "MINS"=w179) -> (w178:T4)  [unwired: 1 in]
                    n135 = local write "LAB03-2 (DISP)"(w178) -> ()
                  }
                  frame #6 {
                    # "update cycle value"
                    # "LAB04-1"
                    n136 = local read "LAB04-1 (DISP)"() -> (w193:T4)
                    n137 = Unbundle(w193) -> ("CYCLE"=w194:dbl)  [unwired: 2 out]
                    n138 = case shown="True" w198 {
                      tunnel: [w199 w201] -> w191
                      tunnel: w194 -> [w199 w200]
                      frame False {
                      }
                      frame True {
                        n139 = Increment(x=w200) -> (x+1=w201:dbl)
                      }
                    }
                    n140 = Multiply(x=w191, y=w195) -> (x*y=w196:dbl)
                    n141 = Divide(x=w196, y=60.0) -> (x/y=w190:dbl)
                    n142 = Bundle(cluster=w193, "CYCLE"=w191, "MINS"=w190) -> (w192:T4)  [unwired: 1 in]
                    n143 = local write "LAB04-1 (DISP)"(w192) -> ()
                  }
                  frame #7 {
                    # "update cycle value"
                    # "LAB04-2"
                    n144 = local read "LAB04-2 (DISP)"() -> (w205:T4)
                    n145 = Unbundle(w205) -> ("CYCLE"=w206:dbl)  [unwired: 2 out]
                    n146 = case shown="True" w210 {
                      tunnel: [w211 w213] -> w203
                      tunnel: w206 -> [w211 w212]
                      frame False {
                      }
                      frame True {
                        n147 = Increment(x=w212) -> (x+1=w213:dbl)
                      }
                    }
                    n148 = Multiply(x=w203, y=w207) -> (x*y=w209:dbl)
                    n149 = Divide(x=w209, y=60.0) -> (x/y=w202:dbl)
                    n150 = Bundle(cluster=w205, "CYCLE"=w203, "MINS"=w202) -> (w204:T4)  [unwired: 1 in]
                    n151 = local write "LAB04-2 (DISP)"(w204) -> ()
                  }
                  frame #8 {
                    # "update cycle value"
                    # "LAB05-1"
                    n152 = local read "LAB05-1 (DISP)"() -> (w217:T4)
                    n153 = Unbundle(w217) -> ("CYCLE"=w218:dbl)  [unwired: 2 out]
                    n154 = case shown="True" w222 {
                      tunnel: [w223 w225] -> w215
                      tunnel: w218 -> [w223 w224]
                      frame False {
                      }
                      frame True {
                        n155 = Increment(x=w224) -> (x+1=w225:dbl)
                      }
                    }
                    n156 = Multiply(x=w215, y=w219) -> (x*y=w220:dbl)
                    n157 = Divide(x=w220, y=60.0) -> (x/y=w214:dbl)
                    n158 = Bundle(cluster=w217, "CYCLE"=w215, "MINS"=w214) -> (w216:T4)  [unwired: 1 in]
                    n159 = local write "LAB05-1 (DISP)"(w216) -> ()
                  }
                  frame #9 {
                    # "update cycle value"
                    # "LAB05-2"
                    n160 = local read "LAB05-2 (DISP)"() -> (w230:T4)
                    n161 = Unbundle(w230) -> ("CYCLE"=w229:dbl)  [unwired: 2 out]
                    n162 = case shown="True" w234 {
                      tunnel: [w235 w237] -> w228
                      tunnel: w229 -> [w235 w236]
                      frame False {
                      }
                      frame True {
                        n163 = Increment(x=w236) -> (x+1=w237:dbl)
                      }
                    }
                    n164 = Multiply(x=w228, y=w231) -> (x*y=w232:dbl)
                    n165 = Divide(x=w232, y=60.0) -> (x/y=w227:dbl)
                    n166 = Bundle(cluster=w230, "CYCLE"=w228, "MINS"=w227) -> (w226:T4)  [unwired: 1 in]
                    n167 = local write "LAB05-2 (DISP)"(w226) -> ()
                  }
                }
                n168 = local write "jig cycle"(0) -> ()
              }
            }
          }
          frame #3 {
            # "check for RUN switch change, start test if true and stop test if false"
            n169 = Get Date/Time In Seconds() -> (seconds since 1Jan1904=w260:timestamp)
            n170 = Format Date/Time String(time format string (%c)="%Y%m%d", seconds (now)=w260) -> (date/time string=w261:string)  [unwired: 1 in]
            n171 = Format Date/Time String(time format string (%c)="%H%M", seconds (now)=w260) -> (date/time string=w258:string)  [unwired: 1 in]
            n172 = event shown="[3] \"LAB02-1 RUN\": Value Change" {
              selector: _ -> [_ _ _ _ _ _ _ _ _ _ _]
              dyn-events: _ -> [_ _ _ _ _ _ _ _ _ _ _]
              timeout: 10 -> [_ _ _ _ _ _ _ _ _ _ _]
              tunnel: "c:\\crabtree\\Test Data\\" -> [_ w269 w347 w425 w503 w581 w659 w737 w815 w893 w971]
              tunnel: w261 -> [_ w268 w346 w424 w502 w580 w658 w736 w814 w892 w970]
              tunnel: w258 -> [_ w266 w345 w423 w501 w579 w657 w735 w813 w891 w969]
              tunnel: w256 -> [_ w267 _ _ _ _ _ _ _ _ _]
              tunnel: w257 -> [_ w265 _ _ _ _ _ _ _ _ _]
              tunnel: w255 -> [_ _ w344 _ _ _ _ _ _ _ _]
              tunnel: w254 -> [_ _ w343 _ _ _ _ _ _ _ _]
              tunnel: w253 -> [_ _ _ w422 _ _ _ _ _ _ _]
              tunnel: w252 -> [_ _ _ w421 _ _ _ _ _ _ _]
              tunnel: w251 -> [_ _ _ _ w500 _ _ _ _ _ _]
              tunnel: w250 -> [_ _ _ _ w499 _ _ _ _ _ _]
              tunnel: w249 -> [_ _ _ _ _ w578 _ _ _ _ _]
              tunnel: w248 -> [_ _ _ _ _ w577 _ _ _ _ _]
              tunnel: w247 -> [_ _ _ _ _ _ w656 _ _ _ _]
              tunnel: w246 -> [_ _ _ _ _ _ w655 _ _ _ _]
              tunnel: w245 -> [_ _ _ _ _ _ _ w734 _ _ _]
              tunnel: w244 -> [_ _ _ _ _ _ _ w733 _ _ _]
              tunnel: w243 -> [_ _ _ _ _ _ _ _ w812 _ _]
              tunnel: w242 -> [_ _ _ _ _ _ _ _ w811 _ _]
              tunnel: w241 -> [_ _ _ _ _ _ _ _ _ w890 _]
              tunnel: w240 -> [_ _ _ _ _ _ _ _ _ w889 _]
              tunnel: w239 -> [_ _ _ _ _ _ _ _ _ _ w968]
              tunnel: w238 -> [_ _ _ _ _ _ _ _ _ _ w967]
              event Timeout {
                n173 = event-data() -> ()  [unwired: 1 in, 3 out]
              }
              event "LAB01-1RUN": Value Change {
                n174 = event-data() -> ()  [unwired: 1 in, 6 out]
                n175 = case shown="True" w265 {
                  tunnel: w269 -> [_ w291]
                  tunnel: w268 -> [_ w290]
                  tunnel: w267 -> [w270 w289]
                  tunnel: w266 -> [_ w288]
                  frame False {
                    # "stop test"
                    n176 = stacked-sequence {
                      tunnel: w270 -> [w276 _]
                      frame #0 {
                        n177 = local read "LAB01-1 (DISP)"() -> (w275:T4)
                        n178 = Unbundle(w275) -> ("CYCLE"=w273:dbl, "MINS"=w274:dbl)  [unwired: 1 out]
                        n179 = case shown="\"CYCLE TEST\"" w276 {
                          tunnel: w274 -> [_ _ w283]
                          tunnel: w273 -> [w281 w282 _]
                          tunnel: [w281 w282 w283] -> w272
                          frame "TEST SET UP", Default {
                          }
                          frame "CYCLE TEST" {
                          }
                          frame "T-RISE TEST" {
                          }
                        }
                        n180 = local read "LAB01-1 (TDMS)"() -> (w280:refnum<k34>)
                        n181 = Build Array("STOPPED") -> (w277:string[])
                        n182 = Build Array(w272) -> (w271:dbl[])
                        n183 = TDMS Write(0:w280, 5:"TEST RESULT", 7:w277, 9:w271) -> ()  [unwired: 2 in, 4 out]
                      }
                      frame #1 {
                        n184 = local read "LAB01-1 (DISP)"() -> (w287:T4)
                        n185 = Bundle(cluster=w287, "STATUS"="STOP") -> (w285:T4)  [unwired: 2 in]
                        n186 = local write "LAB01-1 (RESULT)"(FALSE) -> ()
                        n187 = local write "LAB01-1 (DISP)"(w285) -> ()
                      }
                    }
                  }
                  frame True {
                    # "start new test and create test file"
                    n188 = stacked-sequence {
                      seq-local: [w297 _ _ _ _] -> [_ w316 _ _ _]
                      tunnel: w291 -> [w306 _ _ _ _]
                      tunnel: w290 -> [w304 _ _ _ _]
                      tunnel: w289 -> [w303 _ _ _ _]
                      tunnel: w288 -> [w294 _ _ _ _]
                      frame #0 {
                        n189 = local read "LAB01-1 (SET)"() -> (w296:T5)
                        n190 = case shown="\"TEST SET UP\", Default" w303 {
                          tunnel: ["TEST SET UP-" "CYCLE TEST-" "T-RISE TEST-"] -> w299
                          frame "TEST SET UP", Default {
                          }
                          frame "CYCLE TEST" {
                          }
                          frame "T-RISE TEST" {
                          }
                        }
                        n191 = Unbundle(w296) -> ("DESCRIPTION"=w295:string)  [unwired: 4 out]
                        n192 = Concatenate Strings(w306, "LAB01-1\\", w304, "\\") -> (w300:string)
                        n193 = String To Path(string=w300) -> (path=w302:path)
                        n194 = Concatenate Strings(w300, w299, w295, "-", w294, ".tdms") -> (w297:string)
                        n195 = Create Folder(path (use dialog)=w302) -> (error out=w301:errorcluster)  [unwired: 2 in, 2 out]
                        n196 = call <vilib>:"Clear Errors.vi"("error in (no error)"=w301) -> ()  [unwired: 6 in, 1 out]
                      }
                      frame #1 {
                        n197 = String To Path(string=w316) -> (path=w310:path)
                        n198 = TDMS Open(5:FALSE, 6:FALSE, 10:T13."create or replace" ("operation (0:open)"), 11:w310) -> (0:w312:errorcluster, 3:→"LAB01-1 (TDMS)":refnum<k34>)  [unwired: 3 in]
                        n199 = local write "data file error"(w312) -> ()
                      }
                      frame #2 {
                        n200 = local read "LAB01-1 (SET)"() -> (w322:T5)
                        n201 = local read "LAB01-1 (TDMS)"() -> (w333:refnum<k34>)
                        n202 = Build Array("Testers Name", "Description", "Set Test Cycles", "T-Rise minutes", "T-Rise Deg C") -> (w323:string[])
                        n203 = Unbundle(w322) -> ("NAME"=w321:string, "DESCRIPTION"=w320:string, "CYCLES"=w319:dbl, "T-RISE mins"=w318:dbl, "T-RISE deg C"=w317:dbl)
                        n204 = Number To Decimal String(number=w319) -> (decimal integer string=w332:string)  [unwired: 1 in]
                        n205 = Number To Decimal String(number=w318) -> (decimal integer string=w331:string)  [unwired: 1 in]
                        n206 = Number To Decimal String(number=w317) -> (decimal integer string=w330:string)  [unwired: 1 in]
                        n207 = Build Array(w321, w320, w332, w331, w330) -> (w329:string[])
                        n208 = TDMS Set Properties(5:w329, 7:w323, 11:w333) -> ()  [unwired: 3 in, 4 out]
                      }
                      frame #3 {
                        w335 = 0.0
                        n209 = local read "LAB01-1 (DISP)"() -> (w337:T4)
                        n210 = Bundle(cluster=w337, "CYCLE"=w335, "MINS"=w335, "STATUS"="RUN") -> (w336:T4)
                        n211 = local write "LAB01-1 (DISP)"(w336) -> ()
                      }
                      frame #4 {
                        n212 = local read "LAB01-1 (SIG)"() -> (w340:T2)
                        n213 = local read "LAB01-1 (TEMP START)"() -> (w342:cluster{"TL":dbl, "TN":dbl})
                        n214 = Unbundle(w340) -> ("Tmp Live"=w339:dbl, "Tmp Neut"=w338:dbl)  [unwired: 3 out]
                        n215 = Bundle(cluster=w342, "TL"=w339, "TN"=w338) -> (w341:cluster{"TL":dbl, "TN":dbl})
                        n216 = local write "LAB01-1 (TEMP START)"(w341) -> ()
                      }
                    }
                  }
                }
              }
              event "LAB01-2 RUN": Value Change {
                n217 = event-data() -> ()  [unwired: 1 in, 6 out]
                n218 = case shown="True" w344 {
                  tunnel: w347 -> [_ w369]
                  tunnel: w346 -> [_ w368]
                  tunnel: w343 -> [w348 w367]
                  tunnel: w345 -> [_ w366]
                  frame False {
                    # "stop test"
                    n219 = stacked-sequence {
                      tunnel: w348 -> [w354 _]
                      frame #0 {
                        n220 = local read "LAB01-2 (DISP)"() -> (w353:T4)
                        n221 = Unbundle(w353) -> ("CYCLE"=w351:dbl, "MINS"=w352:dbl)  [unwired: 1 out]
                        n222 = case shown="\"CYCLE TEST\"" w354 {
                          tunnel: w352 -> [_ _ w361]
                          tunnel: w351 -> [w359 w360 _]
                          tunnel: [w359 w360 w361] -> w350
                          frame "TEST SET UP", Default {
                          }
                          frame "CYCLE TEST" {
                          }
                          frame "T-RISE TEST" {
                          }
                        }
                        n223 = local read "LAB01-2 (TDMS)"() -> (w358:refnum<k34>)
                        n224 = Build Array("STOPPED") -> (w355:string[])
                        n225 = Build Array(w350) -> (w349:dbl[])
                        n226 = TDMS Write(0:w358, 5:"TEST RESULT", 7:w355, 9:w349) -> ()  [unwired: 2 in, 4 out]
                      }
                      frame #1 {
                        n227 = local read "LAB01-2 (DISP)"() -> (w365:T4)
                        n228 = Bundle(cluster=w365, "STATUS"="STOP") -> (w363:T4)  [unwired: 2 in]
                        n229 = local write "LAB01-2 (RESULT)"(FALSE) -> ()
                        n230 = local write "LAB01-2 (DISP)"(w363) -> ()
                      }
                    }
                  }
                  frame True {
                    # "start new test and create test file"
                    n231 = stacked-sequence {
                      seq-local: [w375 _ _ _ _] -> [_ w394 _ _ _]
                      tunnel: w369 -> [w384 _ _ _ _]
                      tunnel: w368 -> [w382 _ _ _ _]
                      tunnel: w367 -> [w381 _ _ _ _]
                      tunnel: w366 -> [w372 _ _ _ _]
                      frame #0 {
                        n232 = local read "LAB01-2(SET)"() -> (w374:T5)
                        n233 = case shown="\"TEST SET UP\", Default" w381 {
                          tunnel: ["TEST SET UP-" "CYCLE TEST-" "T-RISE TEST-"] -> w377
                          frame "TEST SET UP", Default {
                          }
                          frame "CYCLE TEST" {
                          }
                          frame "T-RISE TEST" {
                          }
                        }
                        n234 = Unbundle(w374) -> ("DESCRIPTION"=w373:string)  [unwired: 4 out]
                        n235 = Concatenate Strings(w384, "LAB01-2\\", w382, "\\") -> (w378:string)
                        n236 = String To Path(string=w378) -> (path=w380:path)
                        n237 = Concatenate Strings(w378, w377, w373, "-", w372, ".tdms") -> (w375:string)
                        n238 = Create Folder(path (use dialog)=w380) -> (error out=w379:errorcluster)  [unwired: 2 in, 2 out]
                        n239 = call <vilib>:"Clear Errors.vi"("error in (no error)"=w379) -> ()  [unwired: 6 in, 1 out]
                      }
                      frame #1 {
                        n240 = String To Path(string=w394) -> (path=w388:path)
                        n241 = TDMS Open(5:FALSE, 6:FALSE, 10:T13."create or replace" ("operation (0:open)"), 11:w388) -> (0:w390:errorcluster, 3:→"LAB01-2 (TDMS)":refnum<k34>)  [unwired: 3 in]
                        n242 = local write "data file error"(w390) -> ()
                      }
                      frame #2 {
                        n243 = local read "LAB01-2(SET)"() -> (w400:T5)
                        n244 = local read "LAB01-2 (TDMS)"() -> (w411:refnum<k34>)
                        n245 = Build Array("Testers Name", "Description", "Set Test Cycles", "T-Rise minutes", "T-Rise Deg C") -> (w401:string[])
                        n246 = Unbundle(w400) -> ("NAME"=w399:string, "DESCRIPTION"=w398:string, "CYCLES"=w397:dbl, "T-RISE mins"=w396:dbl, "T-RISE deg C"=w395:dbl)
                        n247 = Number To Decimal String(number=w397) -> (decimal integer string=w410:string)  [unwired: 1 in]
                        n248 = Number To Decimal String(number=w396) -> (decimal integer string=w409:string)  [unwired: 1 in]
                        n249 = Number To Decimal String(number=w395) -> (decimal integer string=w408:string)  [unwired: 1 in]
                        n250 = Build Array(w399, w398, w410, w409, w408) -> (w407:string[])
                        n251 = TDMS Set Properties(5:w407, 7:w401, 11:w411) -> ()  [unwired: 3 in, 4 out]
                      }
                      frame #3 {
                        w413 = 0.0
                        n252 = local read "LAB01-2 (DISP)"() -> (w415:T4)
                        n253 = Bundle(cluster=w415, "CYCLE"=w413, "MINS"=w413, "STATUS"="RUN") -> (w414:T4)
                        n254 = local write "LAB01-2 (DISP)"(w414) -> ()
                      }
                      frame #4 {
                        n255 = local read "LAB01-2 (SIG)"() -> (w418:T2)
                        n256 = local read "LAB01-2 (TEMP START)"() -> (w420:cluster{"TL":dbl, "TN":dbl})
                        n257 = Unbundle(w418) -> ("Tmp Live"=w417:dbl, "Tmp Neut"=w416:dbl)  [unwired: 3 out]
                        n258 = Bundle(cluster=w420, "TL"=w417, "TN"=w416) -> (w419:cluster{"TL":dbl, "TN":dbl})
                        n259 = local write "LAB01-2 (TEMP START)"(w419) -> ()
                      }
                    }
                  }
                }
              }
              event "LAB02-1 RUN": Value Change {
                n260 = event-data() -> ()  [unwired: 1 in, 6 out]
                n261 = case shown="False" w422 {
                  tunnel: w425 -> [_ w447]
                  tunnel: w424 -> [_ w446]
                  tunnel: w421 -> [w426 w445]
                  tunnel: w423 -> [_ w444]
                  frame False {
                    # "stop test"
                    n262 = stacked-sequence {
                      tunnel: w426 -> [w432 _]
                      frame #0 {
                        n263 = local read "LAB02-1 (DISP)"() -> (w431:T4)
                        n264 = Unbundle(w431) -> ("CYCLE"=w429:dbl, "MINS"=w430:dbl)  [unwired: 1 out]
                        n265 = case shown="\"CYCLE TEST\"" w432 {
                          tunnel: w430 -> [_ _ w439]
                          tunnel: w429 -> [w437 w438 _]
                          tunnel: [w437 w438 w439] -> w428
                          frame "TEST SET UP", Default {
                          }
                          frame "CYCLE TEST" {
                          }
                          frame "T-RISE TEST" {
                          }
                        }
                        n266 = local read "LAB02-1 (TDMS)"() -> (w436:refnum<k34>)
                        n267 = Build Array("STOPPED") -> (w433:string[])
                        n268 = Build Array(w428) -> (w427:dbl[])
                        n269 = TDMS Write(0:w436, 5:"TEST RESULT", 7:w433, 9:w427) -> ()  [unwired: 2 in, 4 out]
                      }
                      frame #1 {
                        n270 = local read "LAB02-1 (DISP)"() -> (w443:T4)
                        n271 = Bundle(cluster=w443, "STATUS"="STOP") -> (w441:T4)  [unwired: 2 in]
                        n272 = local write "LAB02-1 (RESULT)"(FALSE) -> ()
                        n273 = local write "LAB02-1 (DISP)"(w441) -> ()
                      }
                    }
                  }
                  frame True {
                    # "start new test and create test file"
                    n274 = stacked-sequence {
                      seq-local: [w453 _ _ _ _] -> [_ w472 _ _ _]
                      tunnel: w447 -> [w462 _ _ _ _]
                      tunnel: w446 -> [w460 _ _ _ _]
                      tunnel: w445 -> [w459 _ _ _ _]
                      tunnel: w444 -> [w450 _ _ _ _]
                      frame #0 {
                        n275 = local read "LAB02-1 (SET)"() -> (w452:T5)
                        n276 = case shown="\"TEST SET UP\", Default" w459 {
                          tunnel: ["TEST SET UP-" "CYCLE TEST-" "T-RISE TEST-"] -> w455
                          frame "TEST SET UP", Default {
                          }
                          frame "CYCLE TEST" {
                          }
                          frame "T-RISE TEST" {
                          }
                        }
                        n277 = Unbundle(w452) -> ("DESCRIPTION"=w451:string)  [unwired: 4 out]
                        n278 = Concatenate Strings(w462, "LAB02-1\\", w460, "\\") -> (w456:string)
                        n279 = String To Path(string=w456) -> (path=w458:path)
                        n280 = Concatenate Strings(w456, w455, w451, "-", w450, ".tdms") -> (w453:string)
                        n281 = Create Folder(path (use dialog)=w458) -> (error out=w457:errorcluster)  [unwired: 2 in, 2 out]
                        n282 = call <vilib>:"Clear Errors.vi"("error in (no error)"=w457) -> ()  [unwired: 6 in, 1 out]
                      }
                      frame #1 {
                        n283 = String To Path(string=w472) -> (path=w466:path)
                        n284 = TDMS Open(5:FALSE, 6:FALSE, 10:T13."create or replace" ("operation (0:open)"), 11:w466) -> (0:w468:errorcluster, 3:→"LAB02-1 (TDMS)":refnum<k34>)  [unwired: 3 in]
                        n285 = local write "data file error"(w468) -> ()
                      }
                      frame #2 {
                        n286 = local read "LAB02-1 (SET)"() -> (w478:T5)
                        n287 = local read "LAB02-1 (TDMS)"() -> (w489:refnum<k34>)
                        n288 = Build Array("Testers Name", "Description", "Set Test Cycles", "T-Rise minutes", "T-Rise Deg C") -> (w479:string[])
                        n289 = Unbundle(w478) -> ("NAME"=w477:string, "DESCRIPTION"=w476:string, "CYCLES"=w475:dbl, "T-RISE mins"=w474:dbl, "T-RISE deg C"=w473:dbl)
                        n290 = Number To Decimal String(number=w475) -> (decimal integer string=w488:string)  [unwired: 1 in]
                        n291 = Number To Decimal String(number=w474) -> (decimal integer string=w487:string)  [unwired: 1 in]
                        n292 = Number To Decimal String(number=w473) -> (decimal integer string=w486:string)  [unwired: 1 in]
                        n293 = Build Array(w477, w476, w488, w487, w486) -> (w485:string[])
                        n294 = TDMS Set Properties(5:w485, 7:w479, 11:w489) -> ()  [unwired: 3 in, 4 out]
                      }
                      frame #3 {
                        w491 = 0.0
                        n295 = local read "LAB02-1 (DISP)"() -> (w493:T4)
                        n296 = Bundle(cluster=w493, "CYCLE"=w491, "MINS"=w491, "STATUS"="RUN") -> (w492:T4)
                        n297 = local write "LAB02-1 (DISP)"(w492) -> ()
                      }
                      frame #4 {
                        n298 = local read "LAB02-1 (SIG)"() -> (w496:T2)
                        n299 = local read "LAB02-1 (TEMP START)"() -> (w498:cluster{"TL":dbl, "TN":dbl})
                        n300 = Unbundle(w496) -> ("Tmp Live"=w495:dbl, "Tmp Neut"=w494:dbl)  [unwired: 3 out]
                        n301 = Bundle(cluster=w498, "TL"=w495, "TN"=w494) -> (w497:cluster{"TL":dbl, "TN":dbl})
                        n302 = local write "LAB02-1 (TEMP START)"(w497) -> ()
                      }
                    }
                  }
                }
              }
              event "LAB02-2 RUN": Value Change {
                n303 = event-data() -> ()  [unwired: 1 in, 6 out]
                n304 = case shown="True" w500 {
                  tunnel: w503 -> [_ w525]
                  tunnel: w502 -> [_ w524]
                  tunnel: w499 -> [w504 w523]
                  tunnel: w501 -> [_ w522]
                  frame False {
                    # "stop test"
                    n305 = stacked-sequence {
                      tunnel: w504 -> [w510 _]
                      frame #0 {
                        n306 = local read "LAB02-2 (DISP)"() -> (w509:T4)
                        n307 = Unbundle(w509) -> ("CYCLE"=w507:dbl, "MINS"=w508:dbl)  [unwired: 1 out]
                        n308 = case shown="\"CYCLE TEST\"" w510 {
                          tunnel: w508 -> [_ _ w517]
                          tunnel: w507 -> [w515 w516 _]
                          tunnel: [w515 w516 w517] -> w506
                          frame "TEST SET UP", Default {
                          }
                          frame "CYCLE TEST" {
                          }
                          frame "T-RISE TEST" {
                          }
                        }
                        n309 = local read "LAB02-2 (TDMS)"() -> (w514:refnum<k34>)
                        n310 = Build Array("STOPPED") -> (w511:string[])
                        n311 = Build Array(w506) -> (w505:dbl[])
                        n312 = TDMS Write(0:w514, 5:"TEST RESULT", 7:w511, 9:w505) -> ()  [unwired: 2 in, 4 out]
                      }
                      frame #1 {
                        n313 = local read "LAB02-2 (DISP)"() -> (w521:T4)
                        n314 = Bundle(cluster=w521, "STATUS"="STOP") -> (w519:T4)  [unwired: 2 in]
                        n315 = local write "LAB02-2 (RESULT)"(FALSE) -> ()
                        n316 = local write "LAB02-2 (DISP)"(w519) -> ()
                      }
                    }
                  }
                  frame True {
                    # "start new test and create test file"
                    n317 = stacked-sequence {
                      seq-local: [w531 _ _ _ _] -> [_ w550 _ _ _]
                      tunnel: w525 -> [w540 _ _ _ _]
                      tunnel: w524 -> [w538 _ _ _ _]
                      tunnel: w523 -> [w537 _ _ _ _]
                      tunnel: w522 -> [w528 _ _ _ _]
                      frame #0 {
                        n318 = local read "LAB02-2 (SET)"() -> (w530:T5)
                        n319 = case shown="\"TEST SET UP\", Default" w537 {
                          tunnel: ["TEST SET UP-" "CYCLE TEST-" "T-RISE TEST-"] -> w533
                          frame "TEST SET UP", Default {
                          }
                          frame "CYCLE TEST" {
                          }
                          frame "T-RISE TEST" {
                          }
                        }
                        n320 = Unbundle(w530) -> ("DESCRIPTION"=w529:string)  [unwired: 4 out]
                        n321 = Concatenate Strings(w540, "LAB02-2\\", w538, "\\") -> (w534:string)
                        n322 = String To Path(string=w534) -> (path=w536:path)
                        n323 = Concatenate Strings(w534, w533, w529, "-", w528, ".tdms") -> (w531:string)
                        n324 = Create Folder(path (use dialog)=w536) -> (error out=w535:errorcluster)  [unwired: 2 in, 2 out]
                        n325 = call <vilib>:"Clear Errors.vi"("error in (no error)"=w535) -> ()  [unwired: 6 in, 1 out]
                      }
                      frame #1 {
                        n326 = String To Path(string=w550) -> (path=w544:path)
                        n327 = TDMS Open(5:FALSE, 6:FALSE, 10:T13."create or replace" ("operation (0:open)"), 11:w544) -> (0:w546:errorcluster, 3:→"LAB02-2 (TDMS)":refnum<k34>)  [unwired: 3 in]
                        n328 = local write "data file error"(w546) -> ()
                      }
                      frame #2 {
                        n329 = local read "LAB02-2 (SET)"() -> (w556:T5)
                        n330 = local read "LAB02-2 (TDMS)"() -> (w567:refnum<k34>)
                        n331 = Build Array("Testers Name", "Description", "Set Test Cycles", "T-Rise minutes", "T-Rise Deg C") -> (w557:string[])
                        n332 = Unbundle(w556) -> ("NAME"=w555:string, "DESCRIPTION"=w554:string, "CYCLES"=w553:dbl, "T-RISE mins"=w552:dbl, "T-RISE deg C"=w551:dbl)
                        n333 = Number To Decimal String(number=w553) -> (decimal integer string=w566:string)  [unwired: 1 in]
                        n334 = Number To Decimal String(number=w552) -> (decimal integer string=w565:string)  [unwired: 1 in]
                        n335 = Number To Decimal String(number=w551) -> (decimal integer string=w564:string)  [unwired: 1 in]
                        n336 = Build Array(w555, w554, w566, w565, w564) -> (w563:string[])
                        n337 = TDMS Set Properties(5:w563, 7:w557, 11:w567) -> ()  [unwired: 3 in, 4 out]
                      }
                      frame #3 {
                        w569 = 0.0
                        n338 = local read "LAB02-2 (DISP)"() -> (w571:T4)
                        n339 = Bundle(cluster=w571, "CYCLE"=w569, "MINS"=w569, "STATUS"="RUN") -> (w570:T4)
                        n340 = local write "LAB02-2 (DISP)"(w570) -> ()
                      }
                      frame #4 {
                        n341 = local read "LAB02-2 (SIG)"() -> (w574:T2)
                        n342 = local read "LAB02-2 (TEMP START)"() -> (w576:cluster{"TL":dbl, "TN":dbl})
                        n343 = Unbundle(w574) -> ("Tmp Live"=w573:dbl, "Tmp Neut"=w572:dbl)  [unwired: 3 out]
                        n344 = Bundle(cluster=w576, "TL"=w573, "TN"=w572) -> (w575:cluster{"TL":dbl, "TN":dbl})
                        n345 = local write "LAB02-2 (TEMP START)"(w575) -> ()
                      }
                    }
                  }
                }
              }
              event "LAB03-1 RUN": Value Change {
                n346 = event-data() -> ()  [unwired: 1 in, 6 out]
                n347 = case shown="True" w578 {
                  tunnel: w581 -> [_ w603]
                  tunnel: w580 -> [_ w602]
                  tunnel: w577 -> [w582 w601]
                  tunnel: w579 -> [_ w600]
                  frame False {
                    # "stop test"
                    n348 = stacked-sequence {
                      tunnel: w582 -> [w588 _]
                      frame #0 {
                        n349 = local read "LAB03-1 (DISP)"() -> (w587:T4)
                        n350 = Unbundle(w587) -> ("CYCLE"=w585:dbl, "MINS"=w586:dbl)  [unwired: 1 out]
                        n351 = case shown="\"CYCLE TEST\"" w588 {
                          tunnel: w586 -> [_ _ w595]
                          tunnel: w585 -> [w593 w594 _]
                          tunnel: [w593 w594 w595] -> w584
                          frame "TEST SET UP", Default {
                          }
                          frame "CYCLE TEST" {
                          }
                          frame "T-RISE TEST" {
                          }
                        }
                        n352 = local read "LAB03-1 (TDMS)"() -> (w592:refnum<k34>)
                        n353 = Build Array("STOPPED") -> (w589:string[])
                        n354 = Build Array(w584) -> (w583:dbl[])
                        n355 = TDMS Write(0:w592, 5:"TEST RESULT", 7:w589, 9:w583) -> ()  [unwired: 2 in, 4 out]
                      }
                      frame #1 {
                        n356 = local read "LAB03-1 (DISP)"() -> (w599:T4)
                        n357 = Bundle(cluster=w599, "STATUS"="STOP") -> (w597:T4)  [unwired: 2 in]
                        n358 = local write "LAB03-1 (RESULT)"(FALSE) -> ()
                        n359 = local write "LAB03-1 (DISP)"(w597) -> ()
                      }
                    }
                  }
                  frame True {
                    # "start new test and create test file"
                    n360 = stacked-sequence {
                      seq-local: [w609 _ _ _ _] -> [_ w628 _ _ _]
                      tunnel: w603 -> [w618 _ _ _ _]
                      tunnel: w602 -> [w616 _ _ _ _]
                      tunnel: w601 -> [w615 _ _ _ _]
                      tunnel: w600 -> [w606 _ _ _ _]
                      frame #0 {
                        n361 = local read "LAB03-1 (SET)"() -> (w608:T5)
                        n362 = case shown="\"TEST SET UP\", Default" w615 {
                          tunnel: ["TEST SET UP-" "CYCLE TEST-" "T-RISE TEST-"] -> w611
                          frame "TEST SET UP", Default {
                          }
                          frame "CYCLE TEST" {
                          }
                          frame "T-RISE TEST" {
                          }
                        }
                        n363 = Unbundle(w608) -> ("DESCRIPTION"=w607:string)  [unwired: 4 out]
                        n364 = Concatenate Strings(w618, "LAB03-1\\", w616, "\\") -> (w612:string)
                        n365 = String To Path(string=w612) -> (path=w614:path)
                        n366 = Concatenate Strings(w612, w611, w607, "-", w606, ".tdms") -> (w609:string)
                        n367 = Create Folder(path (use dialog)=w614) -> (error out=w613:errorcluster)  [unwired: 2 in, 2 out]
                        n368 = call <vilib>:"Clear Errors.vi"("error in (no error)"=w613) -> ()  [unwired: 6 in, 1 out]
                      }
                      frame #1 {
                        n369 = String To Path(string=w628) -> (path=w622:path)
                        n370 = TDMS Open(5:FALSE, 6:FALSE, 10:T13."create or replace" ("operation (0:open)"), 11:w622) -> (0:w624:errorcluster, 3:→"LAB03-1 (TDMS)":refnum<k34>)  [unwired: 3 in]
                        n371 = local write "data file error"(w624) -> ()
                      }
                      frame #2 {
                        n372 = local read "LAB03-1 (SET)"() -> (w634:T5)
                        n373 = local read "LAB03-1 (TDMS)"() -> (w645:refnum<k34>)
                        n374 = Build Array("Testers Name", "Description", "Set Test Cycles", "T-Rise minutes", "T-Rise Deg C") -> (w635:string[])
                        n375 = Unbundle(w634) -> ("NAME"=w633:string, "DESCRIPTION"=w632:string, "CYCLES"=w631:dbl, "T-RISE mins"=w630:dbl, "T-RISE deg C"=w629:dbl)
                        n376 = Number To Decimal String(number=w631) -> (decimal integer string=w644:string)  [unwired: 1 in]
                        n377 = Number To Decimal String(number=w630) -> (decimal integer string=w643:string)  [unwired: 1 in]
                        n378 = Number To Decimal String(number=w629) -> (decimal integer string=w642:string)  [unwired: 1 in]
                        n379 = Build Array(w633, w632, w644, w643, w642) -> (w641:string[])
                        n380 = TDMS Set Properties(5:w641, 7:w635, 11:w645) -> ()  [unwired: 3 in, 4 out]
                      }
                      frame #3 {
                        w647 = 0.0
                        n381 = local read "LAB03-1 (DISP)"() -> (w649:T4)
                        n382 = Bundle(cluster=w649, "CYCLE"=w647, "MINS"=w647, "STATUS"="RUN") -> (w648:T4)
                        n383 = local write "LAB03-1 (DISP)"(w648) -> ()
                      }
                      frame #4 {
                        n384 = local read "LAB03-1 (SIG)"() -> (w652:T2)
                        n385 = local read "LAB03-1 (TEMP START)"() -> (w654:cluster{"TL":dbl, "TN":dbl})
                        n386 = Unbundle(w652) -> ("Tmp Live"=w651:dbl, "Tmp Neut"=w650:dbl)  [unwired: 3 out]
                        n387 = Bundle(cluster=w654, "TL"=w651, "TN"=w650) -> (w653:cluster{"TL":dbl, "TN":dbl})
                        n388 = local write "LAB03-1 (TEMP START)"(w653) -> ()
                      }
                    }
                  }
                }
              }
              event "LAB03-2 RUN": Value Change {
                n389 = event-data() -> ()  [unwired: 1 in, 6 out]
                n390 = case shown="True" w656 {
                  tunnel: w659 -> [_ w681]
                  tunnel: w658 -> [_ w680]
                  tunnel: w655 -> [w660 w679]
                  tunnel: w657 -> [_ w678]
                  frame False {
                    # "stop test"
                    n391 = stacked-sequence {
                      tunnel: w660 -> [w666 _]
                      frame #0 {
                        n392 = local read "LAB03-2 (DISP)"() -> (w665:T4)
                        n393 = Unbundle(w665) -> ("CYCLE"=w663:dbl, "MINS"=w664:dbl)  [unwired: 1 out]
                        n394 = case shown="\"CYCLE TEST\"" w666 {
                          tunnel: w664 -> [_ _ w673]
                          tunnel: w663 -> [w671 w672 _]
                          tunnel: [w671 w672 w673] -> w662
                          frame "TEST SET UP", Default {
                          }
                          frame "CYCLE TEST" {
                          }
                          frame "T-RISE TEST" {
                          }
                        }
                        n395 = local read "LAB03-2 (TDMS)"() -> (w670:refnum<k34>)
                        n396 = Build Array("STOPPED") -> (w667:string[])
                        n397 = Build Array(w662) -> (w661:dbl[])
                        n398 = TDMS Write(0:w670, 5:"TEST RESULT", 7:w667, 9:w661) -> ()  [unwired: 2 in, 4 out]
                      }
                      frame #1 {
                        n399 = local read "LAB03-2 (DISP)"() -> (w677:T4)
                        n400 = Bundle(cluster=w677, "STATUS"="STOP") -> (w675:T4)  [unwired: 2 in]
                        n401 = local write "LAB03-2 (RESULT)"(FALSE) -> ()
                        n402 = local write "LAB03-2 (DISP)"(w675) -> ()
                      }
                    }
                  }
                  frame True {
                    # "start new test and create test file"
                    n403 = stacked-sequence {
                      seq-local: [w687 _ _ _ _] -> [_ w706 _ _ _]
                      tunnel: w681 -> [w696 _ _ _ _]
                      tunnel: w680 -> [w694 _ _ _ _]
                      tunnel: w679 -> [w693 _ _ _ _]
                      tunnel: w678 -> [w684 _ _ _ _]
                      frame #0 {
                        n404 = local read "LAB03-2 (SET)"() -> (w686:T5)
                        n405 = case shown="\"TEST SET UP\", Default" w693 {
                          tunnel: ["TEST SET UP-" "CYCLE TEST-" "T-RISE TEST-"] -> w689
                          frame "TEST SET UP", Default {
                          }
                          frame "CYCLE TEST" {
                          }
                          frame "T-RISE TEST" {
                          }
                        }
                        n406 = Unbundle(w686) -> ("DESCRIPTION"=w685:string)  [unwired: 4 out]
                        n407 = Concatenate Strings(w696, "LAB03-2\\", w694, "\\") -> (w690:string)
                        n408 = String To Path(string=w690) -> (path=w692:path)
                        n409 = Concatenate Strings(w690, w689, w685, "-", w684, ".tdms") -> (w687:string)
                        n410 = Create Folder(path (use dialog)=w692) -> (error out=w691:errorcluster)  [unwired: 2 in, 2 out]
                        n411 = call <vilib>:"Clear Errors.vi"("error in (no error)"=w691) -> ()  [unwired: 6 in, 1 out]
                      }
                      frame #1 {
                        n412 = String To Path(string=w706) -> (path=w700:path)
                        n413 = TDMS Open(5:FALSE, 6:FALSE, 10:T13."create or replace" ("operation (0:open)"), 11:w700) -> (0:w702:errorcluster, 3:→"LAB03-2 (TDMS)":refnum<k34>)  [unwired: 3 in]
                        n414 = local write "data file error"(w702) -> ()
                      }
                      frame #2 {
                        n415 = local read "LAB03-2 (SET)"() -> (w712:T5)
                        n416 = local read "LAB03-2 (TDMS)"() -> (w723:refnum<k34>)
                        n417 = Build Array("Testers Name", "Description", "Set Test Cycles", "T-Rise minutes", "T-Rise Deg C") -> (w713:string[])
                        n418 = Unbundle(w712) -> ("NAME"=w711:string, "DESCRIPTION"=w710:string, "CYCLES"=w709:dbl, "T-RISE mins"=w708:dbl, "T-RISE deg C"=w707:dbl)
                        n419 = Number To Decimal String(number=w709) -> (decimal integer string=w722:string)  [unwired: 1 in]
                        n420 = Number To Decimal String(number=w708) -> (decimal integer string=w721:string)  [unwired: 1 in]
                        n421 = Number To Decimal String(number=w707) -> (decimal integer string=w720:string)  [unwired: 1 in]
                        n422 = Build Array(w711, w710, w722, w721, w720) -> (w719:string[])
                        n423 = TDMS Set Properties(5:w719, 7:w713, 11:w723) -> ()  [unwired: 3 in, 4 out]
                      }
                      frame #3 {
                        w725 = 0.0
                        n424 = local read "LAB03-2 (DISP)"() -> (w727:T4)
                        n425 = Bundle(cluster=w727, "CYCLE"=w725, "MINS"=w725, "STATUS"="RUN") -> (w726:T4)
                        n426 = local write "LAB03-2 (DISP)"(w726) -> ()
                      }
                      frame #4 {
                        n427 = local read "LAB03-2 (SIG)"() -> (w730:T2)
                        n428 = local read "LAB03-2 (TEMP START)"() -> (w732:cluster{"TL":dbl, "TN":dbl})
                        n429 = Unbundle(w730) -> ("Tmp Live"=w729:dbl, "Tmp Neut"=w728:dbl)  [unwired: 3 out]
                        n430 = Bundle(cluster=w732, "TL"=w729, "TN"=w728) -> (w731:cluster{"TL":dbl, "TN":dbl})
                        n431 = local write "LAB03-2 (TEMP START)"(w731) -> ()
                      }
                    }
                  }
                }
              }
              event "LAB04-1 RUN": Value Change {
                n432 = event-data() -> ()  [unwired: 1 in, 6 out]
                n433 = case shown="True" w734 {
                  tunnel: w737 -> [_ w759]
                  tunnel: w736 -> [_ w758]
                  tunnel: w733 -> [w738 w757]
                  tunnel: w735 -> [_ w756]
                  frame False {
                    # "stop test"
                    n434 = stacked-sequence {
                      tunnel: w738 -> [w744 _]
                      frame #0 {
                        n435 = local read "LAB04-1 (DISP)"() -> (w743:T4)
                        n436 = Unbundle(w743) -> ("CYCLE"=w741:dbl, "MINS"=w742:dbl)  [unwired: 1 out]
                        n437 = case shown="\"CYCLE TEST\"" w744 {
                          tunnel: w742 -> [_ _ w751]
                          tunnel: w741 -> [w749 w750 _]
                          tunnel: [w749 w750 w751] -> w740
                          frame "TEST SET UP", Default {
                          }
                          frame "CYCLE TEST" {
                          }
                          frame "T-RISE TEST" {
                          }
                        }
                        n438 = local read "LAB04-1 (TDMS)"() -> (w748:refnum<k34>)
                        n439 = Build Array("STOPPED") -> (w745:string[])
                        n440 = Build Array(w740) -> (w739:dbl[])
                        n441 = TDMS Write(0:w748, 5:"TEST RESULT", 7:w745, 9:w739) -> ()  [unwired: 2 in, 4 out]
                      }
                      frame #1 {
                        n442 = local read "LAB04-1 (DISP)"() -> (w755:T4)
                        n443 = Bundle(cluster=w755, "STATUS"="STOP") -> (w753:T4)  [unwired: 2 in]
                        n444 = local write "LAB04-1 (RESULT)"(FALSE) -> ()
                        n445 = local write "LAB04-1 (DISP)"(w753) -> ()
                      }
                    }
                  }
                  frame True {
                    # "start new test and create test file"
                    n446 = stacked-sequence {
                      seq-local: [w765 _ _ _ _] -> [_ w784 _ _ _]
                      tunnel: w759 -> [w774 _ _ _ _]
                      tunnel: w758 -> [w772 _ _ _ _]
                      tunnel: w757 -> [w771 _ _ _ _]
                      tunnel: w756 -> [w762 _ _ _ _]
                      frame #0 {
                        n447 = local read "LAB04-1 (SET)"() -> (w764:T5)
                        n448 = case shown="\"TEST SET UP\", Default" w771 {
                          tunnel: ["TEST SET UP-" "CYCLE TEST-" "T-RISE TEST-"] -> w767
                          frame "TEST SET UP", Default {
                          }
                          frame "CYCLE TEST" {
                          }
                          frame "T-RISE TEST" {
                          }
                        }
                        n449 = Unbundle(w764) -> ("DESCRIPTION"=w763:string)  [unwired: 4 out]
                        n450 = Concatenate Strings(w774, "LAB04-1\\", w772, "\\") -> (w768:string)
                        n451 = String To Path(string=w768) -> (path=w770:path)
                        n452 = Concatenate Strings(w768, w767, w763, "-", w762, ".tdms") -> (w765:string)
                        n453 = Create Folder(path (use dialog)=w770) -> (error out=w769:errorcluster)  [unwired: 2 in, 2 out]
                        n454 = call <vilib>:"Clear Errors.vi"("error in (no error)"=w769) -> ()  [unwired: 6 in, 1 out]
                      }
                      frame #1 {
                        n455 = String To Path(string=w784) -> (path=w778:path)
                        n456 = TDMS Open(5:FALSE, 6:FALSE, 10:T13."create or replace" ("operation (0:open)"), 11:w778) -> (0:w780:errorcluster, 3:→"LAB04-1 (TDMS)":refnum<k34>)  [unwired: 3 in]
                        n457 = local write "data file error"(w780) -> ()
                      }
                      frame #2 {
                        n458 = local read "LAB04-1 (SET)"() -> (w790:T5)
                        n459 = local read "LAB04-1 (TDMS)"() -> (w801:refnum<k34>)
                        n460 = Build Array("Testers Name", "Description", "Set Test Cycles", "T-Rise minutes", "T-Rise Deg C") -> (w791:string[])
                        n461 = Unbundle(w790) -> ("NAME"=w789:string, "DESCRIPTION"=w788:string, "CYCLES"=w787:dbl, "T-RISE mins"=w786:dbl, "T-RISE deg C"=w785:dbl)
                        n462 = Number To Decimal String(number=w787) -> (decimal integer string=w800:string)  [unwired: 1 in]
                        n463 = Number To Decimal String(number=w786) -> (decimal integer string=w799:string)  [unwired: 1 in]
                        n464 = Number To Decimal String(number=w785) -> (decimal integer string=w798:string)  [unwired: 1 in]
                        n465 = Build Array(w789, w788, w800, w799, w798) -> (w797:string[])
                        n466 = TDMS Set Properties(5:w797, 7:w791, 11:w801) -> ()  [unwired: 3 in, 4 out]
                      }
                      frame #3 {
                        w803 = 0.0
                        n467 = local read "LAB04-1 (DISP)"() -> (w805:T4)
                        n468 = Bundle(cluster=w805, "CYCLE"=w803, "MINS"=w803, "STATUS"="RUN") -> (w804:T4)
                        n469 = local write "LAB04-1 (DISP)"(w804) -> ()
                      }
                      frame #4 {
                        n470 = local read "LAB04-1 (SIG)"() -> (w808:T2)
                        n471 = local read "LAB04-1 (TEMP START)"() -> (w810:cluster{"TL":dbl, "TN":dbl})
                        n472 = Unbundle(w808) -> ("Tmp Live"=w807:dbl, "Tmp Neut"=w806:dbl)  [unwired: 3 out]
                        n473 = Bundle(cluster=w810, "TL"=w807, "TN"=w806) -> (w809:cluster{"TL":dbl, "TN":dbl})
                        n474 = local write "LAB04-1 (TEMP START)"(w809) -> ()
                      }
                    }
                  }
                }
              }
              event "LAB04-2 RUN": Value Change {
                n475 = event-data() -> ()  [unwired: 1 in, 6 out]
                n476 = case shown="True" w812 {
                  tunnel: w815 -> [_ w837]
                  tunnel: w814 -> [_ w836]
                  tunnel: w811 -> [w816 w835]
                  tunnel: w813 -> [_ w834]
                  frame False {
                    # "stop test"
                    n477 = stacked-sequence {
                      tunnel: w816 -> [w822 _]
                      frame #0 {
                        n478 = local read "LAB04-2 (DISP)"() -> (w821:T4)
                        n479 = Unbundle(w821) -> ("CYCLE"=w819:dbl, "MINS"=w820:dbl)  [unwired: 1 out]
                        n480 = case shown="\"CYCLE TEST\"" w822 {
                          tunnel: w820 -> [_ _ w829]
                          tunnel: w819 -> [w827 w828 _]
                          tunnel: [w827 w828 w829] -> w818
                          frame "TEST SET UP", Default {
                          }
                          frame "CYCLE TEST" {
                          }
                          frame "T-RISE TEST" {
                          }
                        }
                        n481 = local read "LAB04-2 (TDMS)"() -> (w826:refnum<k34>)
                        n482 = Build Array("STOPPED") -> (w823:string[])
                        n483 = Build Array(w818) -> (w817:dbl[])
                        n484 = TDMS Write(0:w826, 5:"TEST RESULT", 7:w823, 9:w817) -> ()  [unwired: 2 in, 4 out]
                      }
                      frame #1 {
                        n485 = local read "LAB04-2 (DISP)"() -> (w833:T4)
                        n486 = Bundle(cluster=w833, "STATUS"="STOP") -> (w831:T4)  [unwired: 2 in]
                        n487 = local write "LAB04-2 (RESULT)"(FALSE) -> ()
                        n488 = local write "LAB04-2 (DISP)"(w831) -> ()
                      }
                    }
                  }
                  frame True {
                    # "start new test and create test file"
                    n489 = stacked-sequence {
                      seq-local: [w843 _ _ _ _] -> [_ w862 _ _ _]
                      tunnel: w837 -> [w852 _ _ _ _]
                      tunnel: w836 -> [w850 _ _ _ _]
                      tunnel: w835 -> [w849 _ _ _ _]
                      tunnel: w834 -> [w840 _ _ _ _]
                      frame #0 {
                        n490 = local read "LAB04-2 (SET)"() -> (w842:T5)
                        n491 = case shown="\"TEST SET UP\", Default" w849 {
                          tunnel: ["TEST SET UP-" "CYCLE TEST-" "T-RISE TEST-"] -> w845
                          frame "TEST SET UP", Default {
                          }
                          frame "CYCLE TEST" {
                          }
                          frame "T-RISE TEST" {
                          }
                        }
                        n492 = Unbundle(w842) -> ("DESCRIPTION"=w841:string)  [unwired: 4 out]
                        n493 = Concatenate Strings(w852, "LAB04-2\\", w850, "\\") -> (w846:string)
                        n494 = String To Path(string=w846) -> (path=w848:path)
                        n495 = Concatenate Strings(w846, w845, w841, "-", w840, ".tdms") -> (w843:string)
                        n496 = Create Folder(path (use dialog)=w848) -> (error out=w847:errorcluster)  [unwired: 2 in, 2 out]
                        n497 = call <vilib>:"Clear Errors.vi"("error in (no error)"=w847) -> ()  [unwired: 6 in, 1 out]
                      }
                      frame #1 {
                        n498 = String To Path(string=w862) -> (path=w856:path)
                        n499 = TDMS Open(5:FALSE, 6:FALSE, 10:T13."create or replace" ("operation (0:open)"), 11:w856) -> (0:w858:errorcluster, 3:→"LAB04-2 (TDMS)":refnum<k34>)  [unwired: 3 in]
                        n500 = local write "data file error"(w858) -> ()
                      }
                      frame #2 {
                        n501 = local read "LAB04-2 (SET)"() -> (w868:T5)
                        n502 = local read "LAB04-2 (TDMS)"() -> (w879:refnum<k34>)
                        n503 = Build Array("Testers Name", "Description", "Set Test Cycles", "T-Rise minutes", "T-Rise Deg C") -> (w869:string[])
                        n504 = Unbundle(w868) -> ("NAME"=w867:string, "DESCRIPTION"=w866:string, "CYCLES"=w865:dbl, "T-RISE mins"=w864:dbl, "T-RISE deg C"=w863:dbl)
                        n505 = Number To Decimal String(number=w865) -> (decimal integer string=w878:string)  [unwired: 1 in]
                        n506 = Number To Decimal String(number=w864) -> (decimal integer string=w877:string)  [unwired: 1 in]
                        n507 = Number To Decimal String(number=w863) -> (decimal integer string=w876:string)  [unwired: 1 in]
                        n508 = Build Array(w867, w866, w878, w877, w876) -> (w875:string[])
                        n509 = TDMS Set Properties(5:w875, 7:w869, 11:w879) -> ()  [unwired: 3 in, 4 out]
                      }
                      frame #3 {
                        w881 = 0.0
                        n510 = local read "LAB04-2 (DISP)"() -> (w883:T4)
                        n511 = Bundle(cluster=w883, "CYCLE"=w881, "MINS"=w881, "STATUS"="RUN") -> (w882:T4)
                        n512 = local write "LAB04-2 (DISP)"(w882) -> ()
                      }
                      frame #4 {
                        n513 = local read "LAB04-2 (SIG)"() -> (w886:T2)
                        n514 = local read "LAB04-2 (TEMP START)"() -> (w888:cluster{"TL":dbl, "TN":dbl})
                        n515 = Unbundle(w886) -> ("Tmp Live"=w885:dbl, "Tmp Neut"=w884:dbl)  [unwired: 3 out]
                        n516 = Bundle(cluster=w888, "TL"=w885, "TN"=w884) -> (w887:cluster{"TL":dbl, "TN":dbl})
                        n517 = local write "LAB04-2 (TEMP START)"(w887) -> ()
                      }
                    }
                  }
                }
              }
              event "LAB05-1 RUN": Value Change {
                n518 = event-data() -> ()  [unwired: 1 in, 6 out]
                n519 = case shown="True" w890 {
                  tunnel: w893 -> [_ w915]
                  tunnel: w892 -> [_ w914]
                  tunnel: w889 -> [w894 w913]
                  tunnel: w891 -> [_ w912]
                  frame False {
                    # "stop test"
                    n520 = stacked-sequence {
                      tunnel: w894 -> [w900 _]
                      frame #0 {
                        n521 = local read "LAB05-1 (DISP)"() -> (w899:T4)
                        n522 = Unbundle(w899) -> ("CYCLE"=w897:dbl, "MINS"=w898:dbl)  [unwired: 1 out]
                        n523 = case shown="\"CYCLE TEST\"" w900 {
                          tunnel: w898 -> [_ _ w907]
                          tunnel: w897 -> [w905 w906 _]
                          tunnel: [w905 w906 w907] -> w896
                          frame "TEST SET UP", Default {
                          }
                          frame "CYCLE TEST" {
                          }
                          frame "T-RISE TEST" {
                          }
                        }
                        n524 = local read "LAB05-1 (TDMS)"() -> (w904:refnum<k34>)
                        n525 = Build Array("STOPPED") -> (w901:string[])
                        n526 = Build Array(w896) -> (w895:dbl[])
                        n527 = TDMS Write(0:w904, 5:"TEST RESULT", 7:w901, 9:w895) -> ()  [unwired: 2 in, 4 out]
                      }
                      frame #1 {
                        n528 = local read "LAB05-1 (DISP)"() -> (w911:T4)
                        n529 = Bundle(cluster=w911, "STATUS"="STOP") -> (w909:T4)  [unwired: 2 in]
                        n530 = local write "LAB05-1 (RESULT)"(FALSE) -> ()
                        n531 = local write "LAB05-1 (DISP)"(w909) -> ()
                      }
                    }
                  }
                  frame True {
                    # "start new test and create test file"
                    n532 = stacked-sequence {
                      seq-local: [w921 _ _ _ _] -> [_ w940 _ _ _]
                      tunnel: w915 -> [w930 _ _ _ _]
                      tunnel: w914 -> [w928 _ _ _ _]
                      tunnel: w913 -> [w927 _ _ _ _]
                      tunnel: w912 -> [w918 _ _ _ _]
                      frame #0 {
                        n533 = local read "LAB05-1 (SET)"() -> (w920:T5)
                        n534 = case shown="\"TEST SET UP\", Default" w927 {
                          tunnel: ["TEST SET UP-" "CYCLE TEST-" "T-RISE TEST-"] -> w923
                          frame "TEST SET UP", Default {
                          }
                          frame "CYCLE TEST" {
                          }
                          frame "T-RISE TEST" {
                          }
                        }
                        n535 = Unbundle(w920) -> ("DESCRIPTION"=w919:string)  [unwired: 4 out]
                        n536 = Concatenate Strings(w930, "LAB05-1\\", w928, "\\") -> (w924:string)
                        n537 = String To Path(string=w924) -> (path=w926:path)
                        n538 = Concatenate Strings(w924, w923, w919, "-", w918, ".tdms") -> (w921:string)
                        n539 = Create Folder(path (use dialog)=w926) -> (error out=w925:errorcluster)  [unwired: 2 in, 2 out]
                        n540 = call <vilib>:"Clear Errors.vi"("error in (no error)"=w925) -> ()  [unwired: 6 in, 1 out]
                      }
                      frame #1 {
                        n541 = String To Path(string=w940) -> (path=w934:path)
                        n542 = TDMS Open(5:FALSE, 6:FALSE, 10:T13."create or replace" ("operation (0:open)"), 11:w934) -> (0:w936:errorcluster, 3:→"LAB05-1 (TDMS)":refnum<k34>)  [unwired: 3 in]
                        n543 = local write "data file error"(w936) -> ()
                      }
                      frame #2 {
                        n544 = local read "LAB05-1 (SET)"() -> (w946:T5)
                        n545 = local read "LAB05-1 (TDMS)"() -> (w957:refnum<k34>)
                        n546 = Build Array("Testers Name", "Description", "Set Test Cycles", "T-Rise minutes", "T-Rise Deg C") -> (w947:string[])
                        n547 = Unbundle(w946) -> ("NAME"=w945:string, "DESCRIPTION"=w944:string, "CYCLES"=w943:dbl, "T-RISE mins"=w942:dbl, "T-RISE deg C"=w941:dbl)
                        n548 = Number To Decimal String(number=w943) -> (decimal integer string=w956:string)  [unwired: 1 in]
                        n549 = Number To Decimal String(number=w942) -> (decimal integer string=w955:string)  [unwired: 1 in]
                        n550 = Number To Decimal String(number=w941) -> (decimal integer string=w954:string)  [unwired: 1 in]
                        n551 = Build Array(w945, w944, w956, w955, w954) -> (w953:string[])
                        n552 = TDMS Set Properties(5:w953, 7:w947, 11:w957) -> ()  [unwired: 3 in, 4 out]
                      }
                      frame #3 {
                        w959 = 0.0
                        n553 = local read "LAB05-1 (DISP)"() -> (w961:T4)
                        n554 = Bundle(cluster=w961, "CYCLE"=w959, "MINS"=w959, "STATUS"="RUN") -> (w960:T4)
                        n555 = local write "LAB05-1 (DISP)"(w960) -> ()
                      }
                      frame #4 {
                        n556 = local read "LAB05-1 (SIG)"() -> (w964:T2)
                        n557 = local read "LAB05-1 (TEMP START)"() -> (w966:cluster{"TL":dbl, "TN":dbl})
                        n558 = Unbundle(w964) -> ("Tmp Live"=w963:dbl, "Tmp Neut"=w962:dbl)  [unwired: 3 out]
                        n559 = Bundle(cluster=w966, "TL"=w963, "TN"=w962) -> (w965:cluster{"TL":dbl, "TN":dbl})
                        n560 = local write "LAB05-1 (TEMP START)"(w965) -> ()
                      }
                    }
                  }
                }
              }
              event "LAB05-2 RUN": Value Change {
                n561 = event-data() -> ()  [unwired: 1 in, 6 out]
                n562 = case shown="True" w968 {
                  tunnel: w971 -> [_ w993]
                  tunnel: w970 -> [_ w992]
                  tunnel: w967 -> [w972 w991]
                  tunnel: w969 -> [_ w990]
                  frame False {
                    # "stop test"
                    n563 = stacked-sequence {
                      tunnel: w972 -> [w978 _]
                      frame #0 {
                        n564 = local read "LAB05-2 (DISP)"() -> (w977:T4)
                        n565 = Unbundle(w977) -> ("CYCLE"=w975:dbl, "MINS"=w976:dbl)  [unwired: 1 out]
                        n566 = case shown="\"CYCLE TEST\"" w978 {
                          tunnel: w976 -> [_ _ w985]
                          tunnel: w975 -> [w983 w984 _]
                          tunnel: [w983 w984 w985] -> w974
                          frame "TEST SET UP", Default {
                          }
                          frame "CYCLE TEST" {
                          }
                          frame "T-RISE TEST" {
                          }
                        }
                        n567 = local read "LAB05-2 (TDMS)"() -> (w982:refnum<k34>)
                        n568 = Build Array("STOPPED") -> (w979:string[])
                        n569 = Build Array(w974) -> (w973:dbl[])
                        n570 = TDMS Write(0:w982, 5:"TEST RESULT", 7:w979, 9:w973) -> ()  [unwired: 2 in, 4 out]
                      }
                      frame #1 {
                        n571 = local read "LAB05-2 (DISP)"() -> (w989:T4)
                        n572 = Bundle(cluster=w989, "STATUS"="STOP") -> (w987:T4)  [unwired: 2 in]
                        n573 = local write "LAB05-2 (RESULT)"(FALSE) -> ()
                        n574 = local write "LAB05-2 (DISP)"(w987) -> ()
                      }
                    }
                  }
                  frame True {
                    # "start new test and create test file"
                    n575 = stacked-sequence {
                      seq-local: [w999 _ _ _ _] -> [_ w1018 _ _ _]
                      tunnel: w993 -> [w1008 _ _ _ _]
                      tunnel: w992 -> [w1006 _ _ _ _]
                      tunnel: w991 -> [w1005 _ _ _ _]
                      tunnel: w990 -> [w996 _ _ _ _]
                      frame #0 {
                        n576 = local read "LAB05-2 (SET)"() -> (w998:T5)
                        n577 = case shown="\"TEST SET UP\", Default" w1005 {
                          tunnel: ["TEST SET UP-" "CYCLE TEST-" "T-RISE TEST-"] -> w1001
                          frame "TEST SET UP", Default {
                          }
                          frame "CYCLE TEST" {
                          }
                          frame "T-RISE TEST" {
                          }
                        }
                        n578 = Unbundle(w998) -> ("DESCRIPTION"=w997:string)  [unwired: 4 out]
                        n579 = Concatenate Strings(w1008, "LAB05-2\\", w1006, "\\") -> (w1002:string)
                        n580 = String To Path(string=w1002) -> (path=w1004:path)
                        n581 = Concatenate Strings(w1002, w1001, w997, "-", w996, ".tdms") -> (w999:string)
                        n582 = Create Folder(path (use dialog)=w1004) -> (error out=w1003:errorcluster)  [unwired: 2 in, 2 out]
                        n583 = call <vilib>:"Clear Errors.vi"("error in (no error)"=w1003) -> ()  [unwired: 6 in, 1 out]
                      }
                      frame #1 {
                        n584 = String To Path(string=w1018) -> (path=w1012:path)
                        n585 = TDMS Open(5:FALSE, 6:FALSE, 10:T13."create or replace" ("operation (0:open)"), 11:w1012) -> (0:w1014:errorcluster, 3:→"LAB05-2 (TDMS)":refnum<k34>)  [unwired: 3 in]
                        n586 = local write "data file error"(w1014) -> ()
                      }
                      frame #2 {
                        n587 = local read "LAB05-2 (SET)"() -> (w1024:T5)
                        n588 = local read "LAB05-2 (TDMS)"() -> (w1035:refnum<k34>)
                        n589 = Build Array("Testers Name", "Description", "Set Test Cycles", "T-Rise minutes", "T-Rise Deg C") -> (w1025:string[])
                        n590 = Unbundle(w1024) -> ("NAME"=w1023:string, "DESCRIPTION"=w1022:string, "CYCLES"=w1021:dbl, "T-RISE mins"=w1020:dbl, "T-RISE deg C"=w1019:dbl)
                        n591 = Number To Decimal String(number=w1021) -> (decimal integer string=w1034:string)  [unwired: 1 in]
                        n592 = Number To Decimal String(number=w1020) -> (decimal integer string=w1033:string)  [unwired: 1 in]
                        n593 = Number To Decimal String(number=w1019) -> (decimal integer string=w1032:string)  [unwired: 1 in]
                        n594 = Build Array(w1023, w1022, w1034, w1033, w1032) -> (w1031:string[])
                        n595 = TDMS Set Properties(5:w1031, 7:w1025, 11:w1035) -> ()  [unwired: 3 in, 4 out]
                      }
                      frame #3 {
                        w1037 = 0.0
                        n596 = local read "LAB05-2 (DISP)"() -> (w1039:T4)
                        n597 = Bundle(cluster=w1039, "CYCLE"=w1037, "MINS"=w1037, "STATUS"="RUN") -> (w1038:T4)
                        n598 = local write "LAB05-2 (DISP)"(w1038) -> ()
                      }
                      frame #4 {
                        n599 = local read "LAB05-2 (SIG)"() -> (w1042:T2)
                        n600 = local read "LAB05-2 (TEMP START)"() -> (w1044:cluster{"TL":dbl, "TN":dbl})
                        n601 = Unbundle(w1042) -> ("Tmp Live"=w1041:dbl, "Tmp Neut"=w1040:dbl)  [unwired: 3 out]
                        n602 = Bundle(cluster=w1044, "TL"=w1041, "TN"=w1040) -> (w1043:cluster{"TL":dbl, "TN":dbl})
                        n603 = local write "LAB05-2 (TEMP START)"(w1043) -> ()
                      }
                    }
                  }
                }
              }
            }
          }
          frame #4 {
            # "check if test cycles reached for cycle tests, if so then test pass"
            n604 = stacked-sequence {
              tunnel: w1064 -> [_ _ _ _ _ _ _ _ _ _]
              tunnel: w1063 -> [_ _ _ _ _ _ _ _ _ _]
              tunnel: w1062 -> [_ _ _ _ _ _ _ _ _ _]
              tunnel: w1061 -> [_ _ _ _ _ _ _ _ _ _]
              tunnel: w1060 -> [_ _ _ _ _ _ _ _ _ _]
              tunnel: w1059 -> [_ _ _ _ _ _ _ _ _ _]
              tunnel: w1058 -> [_ _ _ _ _ _ _ _ _ _]
              tunnel: w1057 -> [_ _ _ _ _ _ _ _ _ _]
              tunnel: w1056 -> [_ _ _ _ _ _ _ _ _ _]
              tunnel: w1055 -> [_ _ _ _ _ _ _ _ _ _]
              tunnel: w1054 -> [w1069 _ _ _ _ _ _ _ _ _]
              tunnel: w1053 -> [_ w1104 _ _ _ _ _ _ _ _]
              tunnel: w1052 -> [_ _ w1143 _ _ _ _ _ _ _]
              tunnel: w1051 -> [_ _ _ w1182 _ _ _ _ _ _]
              tunnel: w1050 -> [_ _ _ _ w1221 _ _ _ _ _]
              tunnel: w1049 -> [_ _ _ _ _ w1260 _ _ _ _]
              tunnel: w1048 -> [_ _ _ _ _ _ w1299 _ _ _]
              tunnel: w1047 -> [_ _ _ _ _ _ _ w1338 _ _]
              tunnel: w1046 -> [_ _ _ _ _ _ _ _ w1377 _]
              tunnel: w1045 -> [_ _ _ _ _ _ _ _ _ w1416]
              frame #0 {
                # "LAB01-1"
                n605 = Less?(x=w1069, y=2) -> (x < y?=w1067:bool)
                n606 = local read "LAB01-1 (DISP)"() -> (w1070:T4)
                n607 = Unbundle(w1070) -> ("STATUS"=w1071:string)  [unwired: 2 out]
                n608 = Equal?(x=w1071, y="RUN") -> (x = y?=w1066:bool)
                n609 = And(x=w1066, y=w1067) -> (x .and. y?=w1065:bool)
                n610 = case shown="True" w1065 {
                  tunnel: w1070 -> [_ w1074]
                  tunnel: w1069 -> [_ w1079]
                  frame False {
                  }
                  frame True {
                    n611 = local read "LAB01-1 (SET)"() -> (w1081:T5)
                    n612 = local read "LAB01-1 (TDMS)"() -> (w1073:refnum<k34>)
                    n613 = Unbundle(w1074) -> ("CYCLE"=w1080:dbl)  [unwired: 2 out]
                    n614 = Unbundle(w1081) -> ("CYCLES"=w1076:dbl, "T-RISE mins"=w1078:dbl)  [unwired: 3 out]
                    n615 = case shown="\"TEST SET UP\", Default" w1079 {
                      tunnel: w1078 -> [_ _ w1088]
                      tunnel: [w1083 w1085 w1088] -> w1077
                      tunnel: w1076 -> [w1083 w1085 _]
                      tunnel: ["TEST SET UP CYCLES" "CYCLES" "T-RISE TEST"] -> w1075
                      frame "TEST SET UP", Default {
                      }
                      frame "CYCLE TEST" {
                      }
                      frame "T-RISE TEST" {
                      }
                    }
                    n616 = Greater Or Equal?(x=w1080, y=w1076) -> (x >= y?=w1082:bool)
                    n617 = case shown="True" w1082 {
                      tunnel: w1077 -> [w1092 _]
                      tunnel: w1075 -> [w1091 _]
                      tunnel: w1074 -> [w1090 _]
                      tunnel: w1073 -> [w1089 _]
                      frame True {
                        n618 = stacked-sequence {
                          tunnel: w1092 -> [w1096 _]
                          tunnel: w1091 -> [w1094 _]
                          tunnel: w1090 -> [_ w1102]
                          tunnel: w1089 -> [w1093 _]
                          frame #0 {
                            n619 = Build Array(w1094) -> (w1097:string[])
                            n620 = Build Array(w1096) -> (w1095:dbl[])
                            n621 = TDMS Write(0:w1093, 5:"TEST PASS", 7:w1097, 9:w1095) -> (15:w1099:errorcluster)  [unwired: 2 in, 3 out]
                            n622 = local write "data file error"(w1099) -> ()
                          }
                          frame #1 {
                            n623 = Bundle(cluster=w1102, "STATUS"="STOP") -> (w1100:T4)  [unwired: 2 in]
                            n624 = local write "LAB01-1 (RESULT)"(TRUE) -> ()
                            n625 = local write "LAB01-1 (DISP)"(w1100) -> ()
                          }
                        }
                      }
                      frame False {
                      }
                    }
                  }
                }
              }
              frame #1 {
                # "LAB01-2"
                n626 = Less?(x=w1104, y=2) -> (x < y?=w1107:bool)
                n627 = local read "LAB01-2 (DISP)"() -> (w1109:T4)
                n628 = Unbundle(w1109) -> ("STATUS"=w1110:string)  [unwired: 2 out]
                n629 = Equal?(x=w1110, y="RUN") -> (x = y?=w1106:bool)
                n630 = And(x=w1106, y=w1107) -> (x .and. y?=w1105:bool)
                n631 = case shown="True" w1105 {
                  tunnel: w1109 -> [_ w1113]
                  tunnel: w1104 -> [_ w1118]
                  frame False {
                  }
                  frame True {
                    n632 = local read "LAB01-2 (TDMS)"() -> (w1112:refnum<k34>)
                    n633 = local read "LAB01-2(SET)"() -> (w1120:T5)
                    n634 = Unbundle(w1113) -> ("CYCLE"=w1119:dbl)  [unwired: 2 out]
                    n635 = Unbundle(w1120) -> ("CYCLES"=w1115:dbl, "T-RISE mins"=w1117:dbl)  [unwired: 3 out]
                    n636 = case shown="\"TEST SET UP\", Default" w1118 {
                      tunnel: w1117 -> [_ _ w1127]
                      tunnel: [w1122 w1124 w1127] -> w1116
                      tunnel: w1115 -> [w1122 w1124 _]
                      tunnel: ["TEST SET UP CYCLES" "CYCLES" "T-RISE TEST"] -> w1114
                      frame "TEST SET UP", Default {
                      }
                      frame "CYCLE TEST" {
                      }
                      frame "T-RISE TEST" {
                      }
                    }
                    n637 = Greater Or Equal?(x=w1119, y=w1115) -> (x >= y?=w1121:bool)
                    n638 = case shown="True" w1121 {
                      tunnel: w1116 -> [w1131 _]
                      tunnel: w1114 -> [w1130 _]
                      tunnel: w1113 -> [w1129 _]
                      tunnel: w1112 -> [w1128 _]
                      frame True {
                        n639 = stacked-sequence {
                          tunnel: w1131 -> [w1135 _]
                          tunnel: w1130 -> [w1133 _]
                          tunnel: w1129 -> [_ w1141]
                          tunnel: w1128 -> [w1132 _]
                          frame #0 {
                            n640 = Build Array(w1133) -> (w1136:string[])
                            n641 = Build Array(w1135) -> (w1134:dbl[])
                            n642 = TDMS Write(0:w1132, 5:"TEST PASS", 7:w1136, 9:w1134) -> (15:w1138:errorcluster)  [unwired: 2 in, 3 out]
                            n643 = local write "data file error"(w1138) -> ()
                          }
                          frame #1 {
                            n644 = Bundle(cluster=w1141, "STATUS"="STOP") -> (w1139:T4)  [unwired: 2 in]
                            n645 = local write "LAB01-2 (RESULT)"(TRUE) -> ()
                            n646 = local write "LAB01-2 (DISP)"(w1139) -> ()
                          }
                        }
                      }
                      frame False {
                      }
                    }
                  }
                }
              }
              frame #2 {
                # "LAB02-1"
                n647 = Less?(x=w1143, y=2) -> (x < y?=w1146:bool)
                n648 = local read "LAB02-1 (DISP)"() -> (w1148:T4)
                n649 = Unbundle(w1148) -> ("STATUS"=w1149:string)  [unwired: 2 out]
                n650 = Equal?(x=w1149, y="RUN") -> (x = y?=w1145:bool)
                n651 = And(x=w1145, y=w1146) -> (x .and. y?=w1144:bool)
                n652 = case shown="True" w1144 {
                  tunnel: w1148 -> [_ w1152]
                  tunnel: w1143 -> [_ w1157]
                  frame False {
                  }
                  frame True {
                    n653 = local read "LAB02-1 (SET)"() -> (w1159:T5)
                    n654 = local read "LAB02-1 (TDMS)"() -> (w1151:refnum<k34>)
                    n655 = Unbundle(w1152) -> ("CYCLE"=w1158:dbl)  [unwired: 2 out]
                    n656 = Unbundle(w1159) -> ("CYCLES"=w1154:dbl, "T-RISE mins"=w1156:dbl)  [unwired: 3 out]
                    n657 = case shown="\"TEST SET UP\", Default" w1157 {
                      tunnel: w1156 -> [_ _ w1166]
                      tunnel: [w1161 w1163 w1166] -> w1155
                      tunnel: w1154 -> [w1161 w1163 _]
                      tunnel: ["TEST SET UP CYCLES" "CYCLES" "T-RISE TEST"] -> w1153
                      frame "TEST SET UP", Default {
                      }
                      frame "CYCLE TEST" {
                      }
                      frame "T-RISE TEST" {
                      }
                    }
                    n658 = Greater Or Equal?(x=w1158, y=w1154) -> (x >= y?=w1160:bool)
                    n659 = case shown="True" w1160 {
                      tunnel: w1155 -> [w1170 _]
                      tunnel: w1153 -> [w1169 _]
                      tunnel: w1152 -> [w1168 _]
                      tunnel: w1151 -> [w1167 _]
                      frame True {
                        n660 = stacked-sequence {
                          tunnel: w1170 -> [w1174 _]
                          tunnel: w1169 -> [w1172 _]
                          tunnel: w1168 -> [_ w1180]
                          tunnel: w1167 -> [w1171 _]
                          frame #0 {
                            n661 = Build Array(w1172) -> (w1175:string[])
                            n662 = Build Array(w1174) -> (w1173:dbl[])
                            n663 = TDMS Write(0:w1171, 5:"TEST PASS", 7:w1175, 9:w1173) -> (15:w1177:errorcluster)  [unwired: 2 in, 3 out]
                            n664 = local write "data file error"(w1177) -> ()
                          }
                          frame #1 {
                            n665 = Bundle(cluster=w1180, "STATUS"="STOP") -> (w1178:T4)  [unwired: 2 in]
                            n666 = local write "LAB02-1 (RESULT)"(TRUE) -> ()
                            n667 = local write "LAB02-1 (DISP)"(w1178) -> ()
                          }
                        }
                      }
                      frame False {
                      }
                    }
                  }
                }
              }
              frame #3 {
                # "LAB02-2"
                n668 = Less?(x=w1182, y=2) -> (x < y?=w1185:bool)
                n669 = local read "LAB02-2 (DISP)"() -> (w1187:T4)
                n670 = Unbundle(w1187) -> ("STATUS"=w1188:string)  [unwired: 2 out]
                n671 = Equal?(x=w1188, y="RUN") -> (x = y?=w1184:bool)
                n672 = And(x=w1184, y=w1185) -> (x .and. y?=w1183:bool)
                n673 = case shown="True" w1183 {
                  tunnel: w1187 -> [_ w1191]
                  tunnel: w1182 -> [_ w1196]
                  frame False {
                  }
                  frame True {
                    n674 = local read "LAB02-2 (SET)"() -> (w1198:T5)
                    n675 = local read "LAB02-2 (TDMS)"() -> (w1190:refnum<k34>)
                    n676 = Unbundle(w1191) -> ("CYCLE"=w1197:dbl)  [unwired: 2 out]
                    n677 = Unbundle(w1198) -> ("CYCLES"=w1193:dbl, "T-RISE mins"=w1195:dbl)  [unwired: 3 out]
                    n678 = case shown="\"TEST SET UP\", Default" w1196 {
                      tunnel: w1195 -> [_ _ w1205]
                      tunnel: [w1200 w1202 w1205] -> w1194
                      tunnel: w1193 -> [w1200 w1202 _]
                      tunnel: ["TEST SET UP CYCLES" "CYCLES" "T-RISE TEST"] -> w1192
                      frame "TEST SET UP", Default {
                      }
                      frame "CYCLE TEST" {
                      }
                      frame "T-RISE TEST" {
                      }
                    }
                    n679 = Greater Or Equal?(x=w1197, y=w1193) -> (x >= y?=w1199:bool)
                    n680 = case shown="True" w1199 {
                      tunnel: w1194 -> [w1209 _]
                      tunnel: w1192 -> [w1208 _]
                      tunnel: w1191 -> [w1207 _]
                      tunnel: w1190 -> [w1206 _]
                      frame True {
                        n681 = stacked-sequence {
                          tunnel: w1209 -> [w1213 _]
                          tunnel: w1208 -> [w1211 _]
                          tunnel: w1207 -> [_ w1219]
                          tunnel: w1206 -> [w1210 _]
                          frame #0 {
                            n682 = Build Array(w1211) -> (w1214:string[])
                            n683 = Build Array(w1213) -> (w1212:dbl[])
                            n684 = TDMS Write(0:w1210, 5:"TEST PASS", 7:w1214, 9:w1212) -> (15:w1216:errorcluster)  [unwired: 2 in, 3 out]
                            n685 = local write "data file error"(w1216) -> ()
                          }
                          frame #1 {
                            n686 = Bundle(cluster=w1219, "STATUS"="STOP") -> (w1217:T4)  [unwired: 2 in]
                            n687 = local write "LAB02-2 (RESULT)"(TRUE) -> ()
                            n688 = local write "LAB02-2 (DISP)"(w1217) -> ()
                          }
                        }
                      }
                      frame False {
                      }
                    }
                  }
                }
              }
              frame #4 {
                # "LAB03-1"
                n689 = Less?(x=w1221, y=2) -> (x < y?=w1224:bool)
                n690 = local read "LAB03-1 (DISP)"() -> (w1226:T4)
                n691 = Unbundle(w1226) -> ("STATUS"=w1227:string)  [unwired: 2 out]
                n692 = Equal?(x=w1227, y="RUN") -> (x = y?=w1223:bool)
                n693 = And(x=w1223, y=w1224) -> (x .and. y?=w1222:bool)
                n694 = case shown="True" w1222 {
                  tunnel: w1226 -> [_ w1230]
                  tunnel: w1221 -> [_ w1235]
                  frame False {
                  }
                  frame True {
                    n695 = local read "LAB03-1 (SET)"() -> (w1237:T5)
                    n696 = local read "LAB03-1 (TDMS)"() -> (w1229:refnum<k34>)
                    n697 = Unbundle(w1230) -> ("CYCLE"=w1236:dbl)  [unwired: 2 out]
                    n698 = Unbundle(w1237) -> ("CYCLES"=w1232:dbl, "T-RISE mins"=w1234:dbl)  [unwired: 3 out]
                    n699 = case shown="\"TEST SET UP\", Default" w1235 {
                      tunnel: w1234 -> [_ _ w1244]
                      tunnel: [w1239 w1241 w1244] -> w1233
                      tunnel: w1232 -> [w1239 w1241 _]
                      tunnel: ["TEST SET UP CYCLES" "CYCLES" "T-RISE TEST"] -> w1231
                      frame "TEST SET UP", Default {
                      }
                      frame "CYCLE TEST" {
                      }
                      frame "T-RISE TEST" {
                      }
                    }
                    n700 = Greater Or Equal?(x=w1236, y=w1232) -> (x >= y?=w1238:bool)
                    n701 = case shown="True" w1238 {
                      tunnel: w1233 -> [w1248 _]
                      tunnel: w1231 -> [w1247 _]
                      tunnel: w1230 -> [w1246 _]
                      tunnel: w1229 -> [w1245 _]
                      frame True {
                        n702 = stacked-sequence {
                          tunnel: w1248 -> [w1252 _]
                          tunnel: w1247 -> [w1250 _]
                          tunnel: w1246 -> [_ w1258]
                          tunnel: w1245 -> [w1249 _]
                          frame #0 {
                            n703 = Build Array(w1250) -> (w1253:string[])
                            n704 = Build Array(w1252) -> (w1251:dbl[])
                            n705 = TDMS Write(0:w1249, 5:"TEST PASS", 7:w1253, 9:w1251) -> (15:w1255:errorcluster)  [unwired: 2 in, 3 out]
                            n706 = local write "data file error"(w1255) -> ()
                          }
                          frame #1 {
                            n707 = Bundle(cluster=w1258, "STATUS"="STOP") -> (w1256:T4)  [unwired: 2 in]
                            n708 = local write "LAB03-1 (RESULT)"(TRUE) -> ()
                            n709 = local write "LAB03-1 (DISP)"(w1256) -> ()
                          }
                        }
                      }
                      frame False {
                      }
                    }
                  }
                }
              }
              frame #5 {
                # "LAB03-2"
                n710 = Less?(x=w1260, y=2) -> (x < y?=w1263:bool)
                n711 = local read "LAB03-2 (DISP)"() -> (w1265:T4)
                n712 = Unbundle(w1265) -> ("STATUS"=w1266:string)  [unwired: 2 out]
                n713 = Equal?(x=w1266, y="RUN") -> (x = y?=w1262:bool)
                n714 = And(x=w1262, y=w1263) -> (x .and. y?=w1261:bool)
                n715 = case shown="True" w1261 {
                  tunnel: w1265 -> [_ w1269]
                  tunnel: w1260 -> [_ w1274]
                  frame False {
                  }
                  frame True {
                    n716 = local read "LAB03-2 (SET)"() -> (w1276:T5)
                    n717 = local read "LAB03-2 (TDMS)"() -> (w1268:refnum<k34>)
                    n718 = Unbundle(w1269) -> ("CYCLE"=w1275:dbl)  [unwired: 2 out]
                    n719 = Unbundle(w1276) -> ("CYCLES"=w1271:dbl, "T-RISE mins"=w1273:dbl)  [unwired: 3 out]
                    n720 = case shown="\"TEST SET UP\", Default" w1274 {
                      tunnel: w1273 -> [_ _ w1283]
                      tunnel: [w1278 w1280 w1283] -> w1272
                      tunnel: w1271 -> [w1278 w1280 _]
                      tunnel: ["TEST SET UP CYCLES" "CYCLES" "T-RISE TEST"] -> w1270
                      frame "TEST SET UP", Default {
                      }
                      frame "CYCLE TEST" {
                      }
                      frame "T-RISE TEST" {
                      }
                    }
                    n721 = Greater Or Equal?(x=w1275, y=w1271) -> (x >= y?=w1277:bool)
                    n722 = case shown="True" w1277 {
                      tunnel: w1272 -> [w1287 _]
                      tunnel: w1270 -> [w1286 _]
                      tunnel: w1269 -> [w1285 _]
                      tunnel: w1268 -> [w1284 _]
                      frame True {
                        n723 = stacked-sequence {
                          tunnel: w1287 -> [w1291 _]
                          tunnel: w1286 -> [w1289 _]
                          tunnel: w1285 -> [_ w1297]
                          tunnel: w1284 -> [w1288 _]
                          frame #0 {
                            n724 = Build Array(w1289) -> (w1292:string[])
                            n725 = Build Array(w1291) -> (w1290:dbl[])
                            n726 = TDMS Write(0:w1288, 5:"TEST PASS", 7:w1292, 9:w1290) -> (15:w1294:errorcluster)  [unwired: 2 in, 3 out]
                            n727 = local write "data file error"(w1294) -> ()
                          }
                          frame #1 {
                            n728 = Bundle(cluster=w1297, "STATUS"="STOP") -> (w1295:T4)  [unwired: 2 in]
                            n729 = local write "LAB03-2 (RESULT)"(TRUE) -> ()
                            n730 = local write "LAB03-2 (DISP)"(w1295) -> ()
                          }
                        }
                      }
                      frame False {
                      }
                    }
                  }
                }
              }
              frame #6 {
                # "LAB04-1"
                n731 = Less?(x=w1299, y=2) -> (x < y?=w1302:bool)
                n732 = local read "LAB04-1 (DISP)"() -> (w1304:T4)
                n733 = Unbundle(w1304) -> ("STATUS"=w1305:string)  [unwired: 2 out]
                n734 = Equal?(x=w1305, y="RUN") -> (x = y?=w1301:bool)
                n735 = And(x=w1301, y=w1302) -> (x .and. y?=w1300:bool)
                n736 = case shown="True" w1300 {
                  tunnel: w1304 -> [_ w1308]
                  tunnel: w1299 -> [_ w1313]
                  frame False {
                  }
                  frame True {
                    n737 = local read "LAB04-1 (SET)"() -> (w1315:T5)
                    n738 = local read "LAB04-1 (TDMS)"() -> (w1307:refnum<k34>)
                    n739 = Unbundle(w1308) -> ("CYCLE"=w1314:dbl)  [unwired: 2 out]
                    n740 = Unbundle(w1315) -> ("CYCLES"=w1310:dbl, "T-RISE mins"=w1312:dbl)  [unwired: 3 out]
                    n741 = case shown="\"TEST SET UP\", Default" w1313 {
                      tunnel: w1312 -> [_ _ w1322]
                      tunnel: [w1317 w1319 w1322] -> w1311
                      tunnel: w1310 -> [w1317 w1319 _]
                      tunnel: ["TEST SET UP CYCLES" "CYCLES" "T-RISE TEST"] -> w1309
                      frame "TEST SET UP", Default {
                      }
                      frame "CYCLE TEST" {
                      }
                      frame "T-RISE TEST" {
                      }
                    }
                    n742 = Greater Or Equal?(x=w1314, y=w1310) -> (x >= y?=w1316:bool)
                    n743 = case shown="True" w1316 {
                      tunnel: w1311 -> [w1326 _]
                      tunnel: w1309 -> [w1325 _]
                      tunnel: w1308 -> [w1324 _]
                      tunnel: w1307 -> [w1323 _]
                      frame True {
                        n744 = stacked-sequence {
                          tunnel: w1326 -> [w1330 _]
                          tunnel: w1325 -> [w1328 _]
                          tunnel: w1324 -> [_ w1336]
                          tunnel: w1323 -> [w1327 _]
                          frame #0 {
                            n745 = Build Array(w1328) -> (w1331:string[])
                            n746 = Build Array(w1330) -> (w1329:dbl[])
                            n747 = TDMS Write(0:w1327, 5:"TEST PASS", 7:w1331, 9:w1329) -> (15:w1333:errorcluster)  [unwired: 2 in, 3 out]
                            n748 = local write "data file error"(w1333) -> ()
                          }
                          frame #1 {
                            n749 = Bundle(cluster=w1336, "STATUS"="STOP") -> (w1334:T4)  [unwired: 2 in]
                            n750 = local write "LAB04-1 (RESULT)"(TRUE) -> ()
                            n751 = local write "LAB04-1 (DISP)"(w1334) -> ()
                          }
                        }
                      }
                      frame False {
                      }
                    }
                  }
                }
              }
              frame #7 {
                # "LAB04-2"
                n752 = Less?(x=w1338, y=2) -> (x < y?=w1341:bool)
                n753 = local read "LAB04-2 (DISP)"() -> (w1343:T4)
                n754 = Unbundle(w1343) -> ("STATUS"=w1344:string)  [unwired: 2 out]
                n755 = Equal?(x=w1344, y="RUN") -> (x = y?=w1340:bool)
                n756 = And(x=w1340, y=w1341) -> (x .and. y?=w1339:bool)
                n757 = case shown="True" w1339 {
                  tunnel: w1343 -> [_ w1347]
                  tunnel: w1338 -> [_ w1352]
                  frame False {
                  }
                  frame True {
                    n758 = local read "LAB04-2 (SET)"() -> (w1354:T5)
                    n759 = local read "LAB04-2 (TDMS)"() -> (w1346:refnum<k34>)
                    n760 = Unbundle(w1347) -> ("CYCLE"=w1353:dbl)  [unwired: 2 out]
                    n761 = Unbundle(w1354) -> ("CYCLES"=w1349:dbl, "T-RISE mins"=w1351:dbl)  [unwired: 3 out]
                    n762 = case shown="\"TEST SET UP\", Default" w1352 {
                      tunnel: w1351 -> [_ _ w1361]
                      tunnel: [w1356 w1358 w1361] -> w1350
                      tunnel: w1349 -> [w1356 w1358 _]
                      tunnel: ["TEST SET UP CYCLES" "CYCLES" "T-RISE TEST"] -> w1348
                      frame "TEST SET UP", Default {
                      }
                      frame "CYCLE TEST" {
                      }
                      frame "T-RISE TEST" {
                      }
                    }
                    n763 = Greater Or Equal?(x=w1353, y=w1349) -> (x >= y?=w1355:bool)
                    n764 = case shown="True" w1355 {
                      tunnel: w1350 -> [w1365 _]
                      tunnel: w1348 -> [w1364 _]
                      tunnel: w1347 -> [w1363 _]
                      tunnel: w1346 -> [w1362 _]
                      frame True {
                        n765 = stacked-sequence {
                          tunnel: w1365 -> [w1369 _]
                          tunnel: w1364 -> [w1367 _]
                          tunnel: w1363 -> [_ w1375]
                          tunnel: w1362 -> [w1366 _]
                          frame #0 {
                            n766 = Build Array(w1367) -> (w1370:string[])
                            n767 = Build Array(w1369) -> (w1368:dbl[])
                            n768 = TDMS Write(0:w1366, 5:"TEST PASS", 7:w1370, 9:w1368) -> (15:w1372:errorcluster)  [unwired: 2 in, 3 out]
                            n769 = local write "data file error"(w1372) -> ()
                          }
                          frame #1 {
                            n770 = Bundle(cluster=w1375, "STATUS"="STOP") -> (w1373:T4)  [unwired: 2 in]
                            n771 = local write "LAB04-2 (RESULT)"(TRUE) -> ()
                            n772 = local write "LAB04-2 (DISP)"(w1373) -> ()
                          }
                        }
                      }
                      frame False {
                      }
                    }
                  }
                }
              }
              frame #8 {
                # "LAB05-1"
                n773 = Less?(x=w1377, y=2) -> (x < y?=w1380:bool)
                n774 = local read "LAB05-1 (DISP)"() -> (w1382:T4)
                n775 = Unbundle(w1382) -> ("STATUS"=w1383:string)  [unwired: 2 out]
                n776 = Equal?(x=w1383, y="RUN") -> (x = y?=w1379:bool)
                n777 = And(x=w1379, y=w1380) -> (x .and. y?=w1378:bool)
                n778 = case shown="True" w1378 {
                  tunnel: w1382 -> [_ w1386]
                  tunnel: w1377 -> [_ w1391]
                  frame False {
                  }
                  frame True {
                    n779 = local read "LAB05-1 (SET)"() -> (w1393:T5)
                    n780 = local read "LAB05-1 (TDMS)"() -> (w1385:refnum<k34>)
                    n781 = Unbundle(w1386) -> ("CYCLE"=w1392:dbl)  [unwired: 2 out]
                    n782 = Unbundle(w1393) -> ("CYCLES"=w1388:dbl, "T-RISE mins"=w1390:dbl)  [unwired: 3 out]
                    n783 = case shown="\"TEST SET UP\", Default" w1391 {
                      tunnel: w1390 -> [_ _ w1400]
                      tunnel: [w1395 w1397 w1400] -> w1389
                      tunnel: w1388 -> [w1395 w1397 _]
                      tunnel: ["TEST SET UP CYCLES" "CYCLES" "T-RISE TEST"] -> w1387
                      frame "TEST SET UP", Default {
                      }
                      frame "CYCLE TEST" {
                      }
                      frame "T-RISE TEST" {
                      }
                    }
                    n784 = Greater Or Equal?(x=w1392, y=w1388) -> (x >= y?=w1394:bool)
                    n785 = case shown="True" w1394 {
                      tunnel: w1389 -> [w1404 _]
                      tunnel: w1387 -> [w1403 _]
                      tunnel: w1386 -> [w1402 _]
                      tunnel: w1385 -> [w1401 _]
                      frame True {
                        n786 = stacked-sequence {
                          tunnel: w1404 -> [w1408 _]
                          tunnel: w1403 -> [w1406 _]
                          tunnel: w1402 -> [_ w1414]
                          tunnel: w1401 -> [w1405 _]
                          frame #0 {
                            n787 = Build Array(w1406) -> (w1409:string[])
                            n788 = Build Array(w1408) -> (w1407:dbl[])
                            n789 = TDMS Write(0:w1405, 5:"TEST PASS", 7:w1409, 9:w1407) -> (15:w1411:errorcluster)  [unwired: 2 in, 3 out]
                            n790 = local write "data file error"(w1411) -> ()
                          }
                          frame #1 {
                            n791 = Bundle(cluster=w1414, "STATUS"="STOP") -> (w1412:T4)  [unwired: 2 in]
                            n792 = local write "LAB05-1 (RESULT)"(TRUE) -> ()
                            n793 = local write "LAB05-1 (DISP)"(w1412) -> ()
                          }
                        }
                      }
                      frame False {
                      }
                    }
                  }
                }
              }
              frame #9 {
                # "LAB05-2"
                n794 = Less?(x=w1416, y=2) -> (x < y?=w1419:bool)
                n795 = local read "LAB05-2 (DISP)"() -> (w1421:T4)
                n796 = Unbundle(w1421) -> ("STATUS"=w1422:string)  [unwired: 2 out]
                n797 = Equal?(x=w1422, y="RUN") -> (x = y?=w1418:bool)
                n798 = And(x=w1418, y=w1419) -> (x .and. y?=w1417:bool)
                n799 = case shown="True" w1417 {
                  tunnel: w1421 -> [_ w1425]
                  tunnel: w1416 -> [_ w1430]
                  frame False {
                  }
                  frame True {
                    n800 = local read "LAB05-2 (SET)"() -> (w1432:T5)
                    n801 = local read "LAB05-1 (TDMS)"() -> (w1424:refnum<k34>)
                    n802 = Unbundle(w1425) -> ("CYCLE"=w1431:dbl)  [unwired: 2 out]
                    n803 = Unbundle(w1432) -> ("CYCLES"=w1427:dbl, "T-RISE mins"=w1429:dbl)  [unwired: 3 out]
                    n804 = case shown="\"TEST SET UP\", Default" w1430 {
                      tunnel: w1429 -> [_ _ w1439]
                      tunnel: [w1434 w1436 w1439] -> w1428
                      tunnel: w1427 -> [w1434 w1436 _]
                      tunnel: ["TEST SET UP CYCLES" "CYCLES" "T-RISE TEST"] -> w1426
                      frame "TEST SET UP", Default {
                      }
                      frame "CYCLE TEST" {
                      }
                      frame "T-RISE TEST" {
                      }
                    }
                    n805 = Greater Or Equal?(x=w1431, y=w1427) -> (x >= y?=w1433:bool)
                    n806 = case shown="True" w1433 {
                      tunnel: w1428 -> [w1443 _]
                      tunnel: w1426 -> [w1442 _]
                      tunnel: w1425 -> [w1441 _]
                      tunnel: w1424 -> [w1440 _]
                      frame True {
                        n807 = stacked-sequence {
                          tunnel: w1443 -> [w1447 _]
                          tunnel: w1442 -> [w1445 _]
                          tunnel: w1441 -> [_ w1453]
                          tunnel: w1440 -> [w1444 _]
                          frame #0 {
                            n808 = Build Array(w1445) -> (w1448:string[])
                            n809 = Build Array(w1447) -> (w1446:dbl[])
                            n810 = TDMS Write(0:w1444, 5:"TEST PASS", 7:w1448, 9:w1446) -> (15:w1450:errorcluster)  [unwired: 2 in, 3 out]
                            n811 = local write "data file error"(w1450) -> ()
                          }
                          frame #1 {
                            n812 = Bundle(cluster=w1453, "STATUS"="STOP") -> (w1451:T4)  [unwired: 2 in]
                            n813 = local write "LAB05-2 (RESULT)"(TRUE) -> ()
                            n814 = local write "LAB05-2 (DISP)"(w1451) -> ()
                          }
                        }
                      }
                      frame False {
                      }
                    }
                  }
                }
              }
            }
          }
          frame #5 {
            # "check if test cycles reached for temperature rise test"
            n815 = stacked-sequence {
              tunnel: w1475 -> [_ _ _ _ _ _ _ _ _ _]
              tunnel: w1474 -> [_ _ _ _ _ _ _ _ _ _]
              tunnel: w1473 -> [_ _ _ _ _ _ _ _ _ _]
              tunnel: w1472 -> [_ _ _ _ _ _ _ _ _ _]
              tunnel: w1471 -> [_ _ _ _ _ _ _ _ _ _]
              tunnel: w1470 -> [_ _ _ _ _ _ _ _ _ _]
              tunnel: w1469 -> [_ _ _ _ _ _ _ _ _ _]
              tunnel: w1468 -> [_ _ _ _ _ _ _ _ _ _]
              tunnel: w1467 -> [_ _ _ _ _ _ _ _ _ _]
              tunnel: w1466 -> [_ _ _ _ _ _ _ _ _ _]
              tunnel: w1465 -> [w1481 _ _ _ _ _ _ _ _ _]
              tunnel: w1464 -> [w1476 w1507 w1537 w1567 w1597 w1627 w1657 w1687 w1717 w1747]
              tunnel: w1463 -> [_ w1506 _ _ _ _ _ _ _ _]
              tunnel: w1462 -> [_ _ w1536 _ _ _ _ _ _ _]
              tunnel: w1461 -> [_ _ _ w1566 _ _ _ _ _ _]
              tunnel: w1460 -> [_ _ _ _ w1596 _ _ _ _ _]
              tunnel: w1459 -> [_ _ _ _ _ w1626 _ _ _ _]
              tunnel: w1458 -> [_ _ _ _ _ _ w1656 _ _ _]
              tunnel: w1457 -> [_ _ _ _ _ _ _ w1686 _ _]
              tunnel: w1456 -> [_ _ _ _ _ _ _ _ w1716 _]
              tunnel: w1455 -> [_ _ _ _ _ _ _ _ _ w1746]
              frame #0 {
                # "LAB01-1"
                n816 = Equal?(x=w1481, y=2) -> (x = y?=w1479:bool)
                n817 = local read "LAB01-1 (DISP)"() -> (w1482:T4)
                n818 = Unbundle(w1482) -> ("STATUS"=w1483:string)  [unwired: 2 out]
                n819 = Equal?(x=w1483, y="RUN") -> (x = y?=w1478:bool)
                n820 = And(x=w1478, y=w1479) -> (x .and. y?=w1477:bool)
                n821 = case shown="True" w1477 {
                  tunnel: w1482 -> [_ w1486]
                  tunnel: w1476 -> [_ w1489]
                  frame False {
                  }
                  frame True {
                    n822 = local read "LAB01-1 (SET)"() -> (w1488:T5)
                    n823 = local read "LAB01-1 (TDMS)"() -> (w1485:refnum<k34>)
                    n824 = Unbundle(w1486) -> ("CYCLE"=w1490:dbl)  [unwired: 2 out]
                    n825 = Unbundle(w1488) -> ("T-RISE mins"=w1487:dbl)  [unwired: 4 out]
                    n826 = Greater Or Equal?(x=w1490, y=w1489) -> (x >= y?=w1491:bool)
                    n827 = case shown="True" w1491 {
                      tunnel: w1487 -> [w1494 _]
                      tunnel: w1486 -> [w1493 _]
                      tunnel: w1485 -> [w1492 _]
                      frame True {
                        n828 = stacked-sequence {
                          tunnel: w1494 -> [w1497 _]
                          tunnel: w1493 -> [_ w1502]
                          tunnel: w1492 -> [w1495 _]
                          frame #0 {
                            n829 = Build Array("T-RISE") -> (w1499:string[])
                            n830 = Build Array(w1497) -> (w1498:dbl[])
                            n831 = TDMS Write(0:w1495, 5:"TEST PASS", 7:w1499, 9:w1498) -> (15:w1501:errorcluster)  [unwired: 2 in, 3 out]
                            n832 = local write "data file error"(w1501) -> ()
                          }
                          frame #1 {
                            n833 = Bundle(cluster=w1502, "STATUS"="STOP") -> (w1504:T4)  [unwired: 2 in]
                            n834 = local write "LAB01-1 (RESULT)"(TRUE) -> ()
                            n835 = local write "LAB01-1 (DISP)"(w1504) -> ()
                          }
                        }
                      }
                      frame False {
                      }
                    }
                  }
                }
              }
              frame #1 {
                # "LAB01-2"
                n836 = Equal?(x=w1506, y=2) -> (x = y?=w1510:bool)
                n837 = local read "LAB01-2 (DISP)"() -> (w1512:T4)
                n838 = Unbundle(w1512) -> ("STATUS"=w1513:string)  [unwired: 2 out]
                n839 = Equal?(x=w1513, y="RUN") -> (x = y?=w1509:bool)
                n840 = And(x=w1509, y=w1510) -> (x .and. y?=w1508:bool)
                n841 = case shown="True" w1508 {
                  tunnel: w1512 -> [_ w1516]
                  tunnel: w1507 -> [_ w1519]
                  frame False {
                  }
                  frame True {
                    n842 = local read "LAB01-2(SET)"() -> (w1518:T5)
                    n843 = local read "LAB01-2 (TDMS)"() -> (w1515:refnum<k34>)
                    n844 = Unbundle(w1516) -> ("CYCLE"=w1520:dbl)  [unwired: 2 out]
                    n845 = Unbundle(w1518) -> ("T-RISE mins"=w1517:dbl)  [unwired: 4 out]
                    n846 = Greater Or Equal?(x=w1520, y=w1519) -> (x >= y?=w1521:bool)
                    n847 = case shown="True" w1521 {
                      tunnel: w1517 -> [w1524 _]
                      tunnel: w1516 -> [w1523 _]
                      tunnel: w1515 -> [w1522 _]
                      frame True {
                        n848 = stacked-sequence {
                          tunnel: w1524 -> [w1527 _]
                          tunnel: w1523 -> [_ w1532]
                          tunnel: w1522 -> [w1525 _]
                          frame #0 {
                            n849 = Build Array("T-RISE") -> (w1529:string[])
                            n850 = Build Array(w1527) -> (w1528:dbl[])
                            n851 = TDMS Write(0:w1525, 5:"TEST PASS", 7:w1529, 9:w1528) -> (15:w1531:errorcluster)  [unwired: 2 in, 3 out]
                            n852 = local write "data file error"(w1531) -> ()
                          }
                          frame #1 {
                            n853 = Bundle(cluster=w1532, "STATUS"="STOP") -> (w1534:T4)  [unwired: 2 in]
                            n854 = local write "LAB01-2 (RESULT)"(TRUE) -> ()
                            n855 = local write "LAB01-2 (DISP)"(w1534) -> ()
                          }
                        }
                      }
                      frame False {
                      }
                    }
                  }
                }
              }
              frame #2 {
                # "LAB02-1"
                n856 = Equal?(x=w1536, y=2) -> (x = y?=w1540:bool)
                n857 = local read "LAB02-1 (DISP)"() -> (w1542:T4)
                n858 = Unbundle(w1542) -> ("STATUS"=w1543:string)  [unwired: 2 out]
                n859 = Equal?(x=w1543, y="RUN") -> (x = y?=w1539:bool)
                n860 = And(x=w1539, y=w1540) -> (x .and. y?=w1538:bool)
                n861 = case shown="True" w1538 {
                  tunnel: w1542 -> [_ w1546]
                  tunnel: w1537 -> [_ w1549]
                  frame False {
                  }
                  frame True {
                    n862 = local read "LAB02-1 (SET)"() -> (w1548:T5)
                    n863 = local read "LAB02-1 (TDMS)"() -> (w1545:refnum<k34>)
                    n864 = Unbundle(w1546) -> ("CYCLE"=w1550:dbl)  [unwired: 2 out]
                    n865 = Unbundle(w1548) -> ("T-RISE mins"=w1547:dbl)  [unwired: 4 out]
                    n866 = Greater Or Equal?(x=w1550, y=w1549) -> (x >= y?=w1551:bool)
                    n867 = case shown="True" w1551 {
                      tunnel: w1547 -> [w1554 _]
                      tunnel: w1546 -> [w1553 _]
                      tunnel: w1545 -> [w1552 _]
                      frame True {
                        n868 = stacked-sequence {
                          tunnel: w1554 -> [w1557 _]
                          tunnel: w1553 -> [_ w1562]
                          tunnel: w1552 -> [w1555 _]
                          frame #0 {
                            n869 = Build Array("T-RISE") -> (w1559:string[])
                            n870 = Build Array(w1557) -> (w1558:dbl[])
                            n871 = TDMS Write(0:w1555, 5:"TEST PASS", 7:w1559, 9:w1558) -> (15:w1561:errorcluster)  [unwired: 2 in, 3 out]
                            n872 = local write "data file error"(w1561) -> ()
                          }
                          frame #1 {
                            n873 = Bundle(cluster=w1562, "STATUS"="STOP") -> (w1564:T4)  [unwired: 2 in]
                            n874 = local write "LAB02-1 (RESULT)"(TRUE) -> ()
                            n875 = local write "LAB02-1 (DISP)"(w1564) -> ()
                          }
                        }
                      }
                      frame False {
                      }
                    }
                  }
                }
              }
              frame #3 {
                # "LAB02-2"
                n876 = Equal?(x=w1566, y=2) -> (x = y?=w1570:bool)
                n877 = local read "LAB02-2 (DISP)"() -> (w1572:T4)
                n878 = Unbundle(w1572) -> ("STATUS"=w1573:string)  [unwired: 2 out]
                n879 = Equal?(x=w1573, y="RUN") -> (x = y?=w1569:bool)
                n880 = And(x=w1569, y=w1570) -> (x .and. y?=w1568:bool)
                n881 = case shown="True" w1568 {
                  tunnel: w1572 -> [_ w1576]
                  tunnel: w1567 -> [_ w1579]
                  frame False {
                  }
                  frame True {
                    n882 = local read "LAB02-2 (SET)"() -> (w1578:T5)
                    n883 = local read "LAB02-2 (TDMS)"() -> (w1575:refnum<k34>)
                    n884 = Unbundle(w1576) -> ("CYCLE"=w1580:dbl)  [unwired: 2 out]
                    n885 = Unbundle(w1578) -> ("T-RISE mins"=w1577:dbl)  [unwired: 4 out]
                    n886 = Greater Or Equal?(x=w1580, y=w1579) -> (x >= y?=w1581:bool)
                    n887 = case shown="True" w1581 {
                      tunnel: w1577 -> [w1584 _]
                      tunnel: w1576 -> [w1583 _]
                      tunnel: w1575 -> [w1582 _]
                      frame True {
                        n888 = stacked-sequence {
                          tunnel: w1584 -> [w1587 _]
                          tunnel: w1583 -> [_ w1592]
                          tunnel: w1582 -> [w1585 _]
                          frame #0 {
                            n889 = Build Array("T-RISE") -> (w1589:string[])
                            n890 = Build Array(w1587) -> (w1588:dbl[])
                            n891 = TDMS Write(0:w1585, 5:"TEST PASS", 7:w1589, 9:w1588) -> (15:w1591:errorcluster)  [unwired: 2 in, 3 out]
                            n892 = local write "data file error"(w1591) -> ()
                          }
                          frame #1 {
                            n893 = Bundle(cluster=w1592, "STATUS"="STOP") -> (w1594:T4)  [unwired: 2 in]
                            n894 = local write "LAB02-2 (RESULT)"(TRUE) -> ()
                            n895 = local write "LAB02-2 (DISP)"(w1594) -> ()
                          }
                        }
                      }
                      frame False {
                      }
                    }
                  }
                }
              }
              frame #4 {
                # "LAB03-1"
                n896 = Equal?(x=w1596, y=2) -> (x = y?=w1600:bool)
                n897 = local read "LAB03-1 (DISP)"() -> (w1602:T4)
                n898 = Unbundle(w1602) -> ("STATUS"=w1603:string)  [unwired: 2 out]
                n899 = Equal?(x=w1603, y="RUN") -> (x = y?=w1599:bool)
                n900 = And(x=w1599, y=w1600) -> (x .and. y?=w1598:bool)
                n901 = case shown="True" w1598 {
                  tunnel: w1602 -> [_ w1606]
                  tunnel: w1597 -> [_ w1609]
                  frame False {
                  }
                  frame True {
                    n902 = local read "LAB03-1 (SET)"() -> (w1608:T5)
                    n903 = local read "LAB03-1 (TDMS)"() -> (w1605:refnum<k34>)
                    n904 = Unbundle(w1606) -> ("CYCLE"=w1610:dbl)  [unwired: 2 out]
                    n905 = Unbundle(w1608) -> ("T-RISE mins"=w1607:dbl)  [unwired: 4 out]
                    n906 = Greater Or Equal?(x=w1610, y=w1609) -> (x >= y?=w1611:bool)
                    n907 = case shown="True" w1611 {
                      tunnel: w1607 -> [w1614 _]
                      tunnel: w1606 -> [w1613 _]
                      tunnel: w1605 -> [w1612 _]
                      frame True {
                        n908 = stacked-sequence {
                          tunnel: w1614 -> [w1617 _]
                          tunnel: w1613 -> [_ w1622]
                          tunnel: w1612 -> [w1615 _]
                          frame #0 {
                            n909 = Build Array("T-RISE") -> (w1619:string[])
                            n910 = Build Array(w1617) -> (w1618:dbl[])
                            n911 = TDMS Write(0:w1615, 5:"TEST PASS", 7:w1619, 9:w1618) -> (15:w1621:errorcluster)  [unwired: 2 in, 3 out]
                            n912 = local write "data file error"(w1621) -> ()
                          }
                          frame #1 {
                            n913 = Bundle(cluster=w1622, "STATUS"="STOP") -> (w1624:T4)  [unwired: 2 in]
                            n914 = local write "LAB03-1 (RESULT)"(TRUE) -> ()
                            n915 = local write "LAB03-1 (DISP)"(w1624) -> ()
                          }
                        }
                      }
                      frame False {
                      }
                    }
                  }
                }
              }
              frame #5 {
                # "LAB03-2"
                n916 = Equal?(x=w1626, y=2) -> (x = y?=w1630:bool)
                n917 = local read "LAB03-2 (DISP)"() -> (w1632:T4)
                n918 = Unbundle(w1632) -> ("STATUS"=w1633:string)  [unwired: 2 out]
                n919 = Equal?(x=w1633, y="RUN") -> (x = y?=w1629:bool)
                n920 = And(x=w1629, y=w1630) -> (x .and. y?=w1628:bool)
                n921 = case shown="True" w1628 {
                  tunnel: w1632 -> [_ w1636]
                  tunnel: w1627 -> [_ w1639]
                  frame False {
                  }
                  frame True {
                    n922 = local read "LAB03-2 (SET)"() -> (w1638:T5)
                    n923 = local read "LAB03-2 (TDMS)"() -> (w1635:refnum<k34>)
                    n924 = Unbundle(w1636) -> ("CYCLE"=w1640:dbl)  [unwired: 2 out]
                    n925 = Unbundle(w1638) -> ("T-RISE mins"=w1637:dbl)  [unwired: 4 out]
                    n926 = Greater Or Equal?(x=w1640, y=w1639) -> (x >= y?=w1641:bool)
                    n927 = case shown="True" w1641 {
                      tunnel: w1637 -> [w1644 _]
                      tunnel: w1636 -> [w1643 _]
                      tunnel: w1635 -> [w1642 _]
                      frame True {
                        n928 = stacked-sequence {
                          tunnel: w1644 -> [w1647 _]
                          tunnel: w1643 -> [_ w1652]
                          tunnel: w1642 -> [w1645 _]
                          frame #0 {
                            n929 = Build Array("T-RISE") -> (w1649:string[])
                            n930 = Build Array(w1647) -> (w1648:dbl[])
                            n931 = TDMS Write(0:w1645, 5:"TEST PASS", 7:w1649, 9:w1648) -> (15:w1651:errorcluster)  [unwired: 2 in, 3 out]
                            n932 = local write "data file error"(w1651) -> ()
                          }
                          frame #1 {
                            n933 = Bundle(cluster=w1652, "STATUS"="STOP") -> (w1654:T4)  [unwired: 2 in]
                            n934 = local write "LAB03-2 (RESULT)"(TRUE) -> ()
                            n935 = local write "LAB03-2 (DISP)"(w1654) -> ()
                          }
                        }
                      }
                      frame False {
                      }
                    }
                  }
                }
              }
              frame #6 {
                # "LAB04-1"
                n936 = Equal?(x=w1656, y=2) -> (x = y?=w1660:bool)
                n937 = local read "LAB04-1 (DISP)"() -> (w1662:T4)
                n938 = Unbundle(w1662) -> ("STATUS"=w1663:string)  [unwired: 2 out]
                n939 = Equal?(x=w1663, y="RUN") -> (x = y?=w1659:bool)
                n940 = And(x=w1659, y=w1660) -> (x .and. y?=w1658:bool)
                n941 = case shown="True" w1658 {
                  tunnel: w1662 -> [_ w1666]
                  tunnel: w1657 -> [_ w1669]
                  frame False {
                  }
                  frame True {
                    n942 = local read "LAB04-1 (SET)"() -> (w1668:T5)
                    n943 = local read "LAB04-1 (TDMS)"() -> (w1665:refnum<k34>)
                    n944 = Unbundle(w1666) -> ("CYCLE"=w1670:dbl)  [unwired: 2 out]
                    n945 = Unbundle(w1668) -> ("T-RISE mins"=w1667:dbl)  [unwired: 4 out]
                    n946 = Greater Or Equal?(x=w1670, y=w1669) -> (x >= y?=w1671:bool)
                    n947 = case shown="True" w1671 {
                      tunnel: w1667 -> [w1674 _]
                      tunnel: w1666 -> [w1673 _]
                      tunnel: w1665 -> [w1672 _]
                      frame True {
                        n948 = stacked-sequence {
                          tunnel: w1674 -> [w1677 _]
                          tunnel: w1673 -> [_ w1682]
                          tunnel: w1672 -> [w1675 _]
                          frame #0 {
                            n949 = Build Array("T-RISE") -> (w1679:string[])
                            n950 = Build Array(w1677) -> (w1678:dbl[])
                            n951 = TDMS Write(0:w1675, 5:"TEST PASS", 7:w1679, 9:w1678) -> (15:w1681:errorcluster)  [unwired: 2 in, 3 out]
                            n952 = local write "data file error"(w1681) -> ()
                          }
                          frame #1 {
                            n953 = Bundle(cluster=w1682, "STATUS"="STOP") -> (w1684:T4)  [unwired: 2 in]
                            n954 = local write "LAB04-1 (RESULT)"(TRUE) -> ()
                            n955 = local write "LAB04-1 (DISP)"(w1684) -> ()
                          }
                        }
                      }
                      frame False {
                      }
                    }
                  }
                }
              }
              frame #7 {
                # "LAB04-2"
                n956 = Equal?(x=w1686, y=2) -> (x = y?=w1690:bool)
                n957 = local read "LAB04-2 (DISP)"() -> (w1692:T4)
                n958 = Unbundle(w1692) -> ("STATUS"=w1693:string)  [unwired: 2 out]
                n959 = Equal?(x=w1693, y="RUN") -> (x = y?=w1689:bool)
                n960 = And(x=w1689, y=w1690) -> (x .and. y?=w1688:bool)
                n961 = case shown="True" w1688 {
                  tunnel: w1692 -> [_ w1696]
                  tunnel: w1687 -> [_ w1699]
                  frame False {
                  }
                  frame True {
                    n962 = local read "LAB04-2 (SET)"() -> (w1698:T5)
                    n963 = local read "LAB04-2 (TDMS)"() -> (w1695:refnum<k34>)
                    n964 = Unbundle(w1696) -> ("CYCLE"=w1700:dbl)  [unwired: 2 out]
                    n965 = Unbundle(w1698) -> ("T-RISE mins"=w1697:dbl)  [unwired: 4 out]
                    n966 = Greater Or Equal?(x=w1700, y=w1699) -> (x >= y?=w1701:bool)
                    n967 = case shown="True" w1701 {
                      tunnel: w1697 -> [w1704 _]
                      tunnel: w1696 -> [w1703 _]
                      tunnel: w1695 -> [w1702 _]
                      frame True {
                        n968 = stacked-sequence {
                          tunnel: w1704 -> [w1707 _]
                          tunnel: w1703 -> [_ w1712]
                          tunnel: w1702 -> [w1705 _]
                          frame #0 {
                            n969 = Build Array("T-RISE") -> (w1709:string[])
                            n970 = Build Array(w1707) -> (w1708:dbl[])
                            n971 = TDMS Write(0:w1705, 5:"TEST PASS", 7:w1709, 9:w1708) -> (15:w1711:errorcluster)  [unwired: 2 in, 3 out]
                            n972 = local write "data file error"(w1711) -> ()
                          }
                          frame #1 {
                            n973 = Bundle(cluster=w1712, "STATUS"="STOP") -> (w1714:T4)  [unwired: 2 in]
                            n974 = local write "LAB04-2 (RESULT)"(TRUE) -> ()
                            n975 = local write "LAB04-2 (DISP)"(w1714) -> ()
                          }
                        }
                      }
                      frame False {
                      }
                    }
                  }
                }
              }
              frame #8 {
                # "LAB05-1"
                n976 = Equal?(x=w1716, y=2) -> (x = y?=w1720:bool)
                n977 = local read "LAB05-1 (DISP)"() -> (w1722:T4)
                n978 = Unbundle(w1722) -> ("STATUS"=w1723:string)  [unwired: 2 out]
                n979 = Equal?(x=w1723, y="RUN") -> (x = y?=w1719:bool)
                n980 = And(x=w1719, y=w1720) -> (x .and. y?=w1718:bool)
                n981 = case shown="True" w1718 {
                  tunnel: w1722 -> [_ w1726]
                  tunnel: w1717 -> [_ w1729]
                  frame False {
                  }
                  frame True {
                    n982 = local read "LAB05-1 (SET)"() -> (w1728:T5)
                    n983 = local read "LAB05-1 (TDMS)"() -> (w1725:refnum<k34>)
                    n984 = Unbundle(w1726) -> ("CYCLE"=w1730:dbl)  [unwired: 2 out]
                    n985 = Unbundle(w1728) -> ("T-RISE mins"=w1727:dbl)  [unwired: 4 out]
                    n986 = Greater Or Equal?(x=w1730, y=w1729) -> (x >= y?=w1731:bool)
                    n987 = case shown="True" w1731 {
                      tunnel: w1727 -> [w1734 _]
                      tunnel: w1726 -> [w1733 _]
                      tunnel: w1725 -> [w1732 _]
                      frame True {
                        n988 = stacked-sequence {
                          tunnel: w1734 -> [w1737 _]
                          tunnel: w1733 -> [_ w1742]
                          tunnel: w1732 -> [w1735 _]
                          frame #0 {
                            n989 = Build Array("T-RISE") -> (w1739:string[])
                            n990 = Build Array(w1737) -> (w1738:dbl[])
                            n991 = TDMS Write(0:w1735, 5:"TEST PASS", 7:w1739, 9:w1738) -> (15:w1741:errorcluster)  [unwired: 2 in, 3 out]
                            n992 = local write "data file error"(w1741) -> ()
                          }
                          frame #1 {
                            n993 = Bundle(cluster=w1742, "STATUS"="STOP") -> (w1744:T4)  [unwired: 2 in]
                            n994 = local write "LAB05-1 (RESULT)"(TRUE) -> ()
                            n995 = local write "LAB05-1 (DISP)"(w1744) -> ()
                          }
                        }
                      }
                      frame False {
                      }
                    }
                  }
                }
              }
              frame #9 {
                # "LAB05-2"
                n996 = Equal?(x=w1746, y=2) -> (x = y?=w1750:bool)
                n997 = local read "LAB05-2 (DISP)"() -> (w1752:T4)
                n998 = Unbundle(w1752) -> ("STATUS"=w1753:string)  [unwired: 2 out]
                n999 = Equal?(x=w1753, y="RUN") -> (x = y?=w1749:bool)
                n1000 = And(x=w1749, y=w1750) -> (x .and. y?=w1748:bool)
                n1001 = case shown="True" w1748 {
                  tunnel: w1752 -> [_ w1756]
                  tunnel: w1747 -> [_ w1759]
                  frame False {
                  }
                  frame True {
                    n1002 = local read "LAB05-2 (SET)"() -> (w1758:T5)
                    n1003 = local read "LAB05-2 (TDMS)"() -> (w1755:refnum<k34>)
                    n1004 = Unbundle(w1756) -> ("CYCLE"=w1760:dbl)  [unwired: 2 out]
                    n1005 = Unbundle(w1758) -> ("T-RISE mins"=w1757:dbl)  [unwired: 4 out]
                    n1006 = Greater Or Equal?(x=w1760, y=w1759) -> (x >= y?=w1761:bool)
                    n1007 = case shown="True" w1761 {
                      tunnel: w1757 -> [w1764 _]
                      tunnel: w1756 -> [w1763 _]
                      tunnel: w1755 -> [w1762 _]
                      frame True {
                        n1008 = stacked-sequence {
                          tunnel: w1764 -> [w1767 _]
                          tunnel: w1763 -> [_ w1772]
                          tunnel: w1762 -> [w1765 _]
                          frame #0 {
                            n1009 = Build Array("T-RISE") -> (w1769:string[])
                            n1010 = Build Array(w1767) -> (w1768:dbl[])
                            n1011 = TDMS Write(0:w1765, 5:"TEST PASS", 7:w1769, 9:w1768) -> (15:w1771:errorcluster)  [unwired: 2 in, 3 out]
                            n1012 = local write "data file error"(w1771) -> ()
                          }
                          frame #1 {
                            n1013 = Bundle(cluster=w1772, "STATUS"="STOP") -> (w1774:T4)  [unwired: 2 in]
                            n1014 = local write "LAB05-2 (RESULT)"(TRUE) -> ()
                            n1015 = local write "LAB05-2 (DISP)"(w1774) -> ()
                          }
                        }
                      }
                      frame False {
                      }
                    }
                  }
                }
              }
            }
          }
          frame #6 {
            # "disable functions"
            n1016 = stacked-sequence {
              tunnel: w1785 -> [w1795 _ w1845]
              tunnel: w1784 -> [w1794 _ w1844]
              tunnel: w1783 -> [w1793 _ w1843]
              tunnel: w1782 -> [w1792 _ w1842]
              tunnel: w1781 -> [w1791 _ w1841]
              tunnel: w1780 -> [_ w1815 w1840]
              tunnel: w1779 -> [_ w1814 w1839]
              tunnel: w1778 -> [_ w1813 w1838]
              tunnel: w1777 -> [_ w1812 w1837]
              tunnel: w1776 -> [_ w1811 w1836]
              frame #0 {
                n1017 = Select(t=2, s=w1792, f=0) -> (s? t:f=w1787:i32)
                n1018 = Select(t=2, s=w1793, f=0) -> (s? t:f=w1788:i32)
                n1019 = Select(t=2, s=w1791, f=0) -> (s? t:f=w1786:i32)
                n1020 = Select(t=2, s=w1795, f=0) -> (s? t:f=w1790:i32)
                n1021 = Select(t=2, s=w1794, f=0) -> (s? t:f=w1789:i32)
                n1022 = property on="LAB02-2 SELECT" class="RadioBtnsControl (strict)"("DisabledEnum"=w1787) -> ()  [unwired: 2 in, 2 out]
                n1023 = property on="LAB02-1 SELECT" class="RadioBtnsControl (strict)"("DisabledEnum"=w1788) -> ()  [unwired: 2 in, 2 out]
                n1024 = property on="LAB03-1 SELECT" class="RadioBtnsControl (strict)"("DisabledEnum"=w1786) -> ()  [unwired: 2 in, 2 out]
                n1025 = property on="LAB01-1 SELECT" class="RadioBtnsControl (strict)"("DisabledEnum"=w1790) -> ()  [unwired: 2 in, 2 out]
                n1026 = property on="LAB01-2 SELECT" class="RadioBtnsControl (strict)"("DisabledEnum"=w1789) -> ()  [unwired: 2 in, 2 out]
                n1027 = property on="LAB01-2 (RESULT)" class="Bool (strict)"("DisabledEnum"=w1789) -> ()  [unwired: 2 in, 2 out]
                n1028 = property on="LAB02-1 (RESULT)" class="Bool (strict)"("DisabledEnum"=w1788) -> ()  [unwired: 2 in, 2 out]
                n1029 = property on="LAB01-1 (RESULT)" class="Bool (strict)"("DisabledEnum"=w1790) -> ()  [unwired: 2 in, 2 out]
                n1030 = property on="LAB02-2 (RESULT)" class="Bool (strict)"("DisabledEnum"=w1787) -> ()  [unwired: 2 in, 2 out]
                n1031 = property on="LAB03-1 (RESULT)" class="Bool (strict)"("DisabledEnum"=w1786) -> ()  [unwired: 2 in, 2 out]
              }
              frame #1 {
                n1032 = Select(t=2, s=w1811, f=0) -> (s? t:f=w1806:i32)
                n1033 = Select(t=2, s=w1812, f=0) -> (s? t:f=w1807:i32)
                n1034 = Select(t=2, s=w1815, f=0) -> (s? t:f=w1810:i32)
                n1035 = Select(t=2, s=w1814, f=0) -> (s? t:f=w1809:i32)
                n1036 = Select(t=2, s=w1813, f=0) -> (s? t:f=w1808:i32)
                n1037 = property on="LAB05-2 SELECT" class="RadioBtnsControl (strict)"("DisabledEnum"=w1806) -> ()  [unwired: 2 in, 2 out]
                n1038 = property on="LAB05-1 SELECT" class="RadioBtnsControl (strict)"("DisabledEnum"=w1807) -> ()  [unwired: 2 in, 2 out]
                n1039 = property on="LAB03-2 SELECT" class="RadioBtnsControl (strict)"("DisabledEnum"=w1810) -> ()  [unwired: 2 in, 2 out]
                n1040 = property on="LAB04-1 SELECT" class="RadioBtnsControl (strict)"("DisabledEnum"=w1809) -> ()  [unwired: 2 in, 2 out]
                n1041 = property on="LAB04-2 SELECT" class="RadioBtnsControl (strict)"("DisabledEnum"=w1808) -> ()  [unwired: 2 in, 2 out]
                n1042 = property on="LAB03-2 (RESULT)" class="Bool (strict)"("DisabledEnum"=w1810) -> ()  [unwired: 2 in, 2 out]
                n1043 = property on="LAB05-2 (RESULT)" class="Bool (strict)"("DisabledEnum"=w1806) -> ()  [unwired: 2 in, 2 out]
                n1044 = property on="LAB05-1 (RESULT)" class="Bool (strict)"("DisabledEnum"=w1807) -> ()  [unwired: 2 in, 2 out]
                n1045 = property on="LAB04-2 (RESULT)" class="Bool (strict)"("DisabledEnum"=w1808) -> ()  [unwired: 2 in, 2 out]
                n1046 = property on="LAB04-1 (RESULT)" class="Bool (strict)"("DisabledEnum"=w1809) -> ()  [unwired: 2 in, 2 out]
              }
              frame #2 {
                # "disable calibrate if any test running"
                n1047 = Or(x=w1837, y=w1836) -> (x .or. y?=w1830:bool)
                n1048 = Or(x=w1839, y=w1838) -> (x .or. y?=w1832:bool)
                n1049 = Or(x=w1843, y=w1842) -> (x .or. y?=w1834:bool)
                n1050 = Or(x=w1841, y=w1840) -> (x .or. y?=w1833:bool)
                n1051 = Or(x=w1845, y=w1844) -> (x .or. y?=w1835:bool)
                n1052 = Or(x=w1833, y=w1832) -> (x .or. y?=w1831:bool)
                n1053 = Or(x=w1835, y=w1834) -> (x .or. y?=w1829:bool)
                n1054 = Or(x=w1831, y=w1830) -> (x .or. y?=w1828:bool)
                n1055 = Or(x=w1829, y=w1828) -> (x .or. y?=w1827:bool)
                n1056 = case shown="False" w1827 {
                  tunnel: [0 2] -> w1826
                  frame False {
                  }
                  frame True {
                  }
                }
                n1057 = property on="CALIBRATE" class="Bool (strict)"("DisabledEnum"=w1826) -> ()  [unwired: 2 in, 2 out]
              }
            }
          }
          frame #7 {
            # "end test & close test files"
            n1058 = stacked-sequence {
              frame #0 {
                # "LAB01-1"
                n1059 = local read "LAB01-1 (DISP)"() -> (w1849:T4)
                n1060 = local read "LAB01-1 (TDMS)"() -> (w1848:refnum<k34>)
                n1061 = Unbundle(w1849) -> ("STATUS"=w1850:string)  [unwired: 2 out]
                n1062 = Equal?(x=w1850, y="STOP") -> (x = y?=w1851:bool)
                n1063 = case shown="True" w1851 {
                  tunnel: w1849 -> [_ w1854]
                  tunnel: w1848 -> [_ w1853]
                  frame False {
                  }
                  frame True {
                    n1064 = stacked-sequence {
                      tunnel: w1854 -> [w1856 _]
                      tunnel: w1853 -> [_ w1859]
                      frame #0 {
                        n1065 = Bundle(cluster=w1856, "STATUS"="END") -> (w1857:T4)  [unwired: 2 in]
                        n1066 = local write "LAB01-1RUN"(FALSE) -> ()
                        n1067 = local write "LAB01-1 (DISP)"(w1857) -> ()
                      }
                      frame #1 {
                        n1068 = TDMS Close(11:w1859) -> (0:w1860:errorcluster)  [unwired: 1 in, 1 out]
                        n1069 = local write "data file error"(w1860) -> ()
                      }
                    }
                  }
                }
              }
              frame #1 {
                # "LAB01-2"
                n1070 = local read "LAB01-2 (DISP)"() -> (w1862:T4)
                n1071 = local read "LAB01-2 (TDMS)"() -> (w1861:refnum<k34>)
                n1072 = Unbundle(w1862) -> ("STATUS"=w1863:string)  [unwired: 2 out]
                n1073 = Equal?(x=w1863, y="STOP") -> (x = y?=w1864:bool)
                n1074 = case shown="True" w1864 {
                  tunnel: w1862 -> [_ w1867]
                  tunnel: w1861 -> [_ w1866]
                  frame False {
                  }
                  frame True {
                    n1075 = stacked-sequence {
                      tunnel: w1867 -> [w1869 _]
                      tunnel: w1866 -> [_ w1872]
                      frame #0 {
                        n1076 = Bundle(cluster=w1869, "STATUS"="END") -> (w1870:T4)  [unwired: 2 in]
                        n1077 = local write "LAB01-2 RUN"(FALSE) -> ()
                        n1078 = local write "LAB01-2 (DISP)"(w1870) -> ()
                      }
                      frame #1 {
                        n1079 = TDMS Close(11:w1872) -> (0:w1873:errorcluster)  [unwired: 1 in, 1 out]
                        n1080 = local write "data file error"(w1873) -> ()
                      }
                    }
                  }
                }
              }
              frame #2 {
                # "LAB02-1"
                n1081 = local read "LAB02-1 (DISP)"() -> (w1875:T4)
                n1082 = local read "LAB02-1 (TDMS)"() -> (w1874:refnum<k34>)
                n1083 = Unbundle(w1875) -> ("STATUS"=w1876:string)  [unwired: 2 out]
                n1084 = Equal?(x=w1876, y="STOP") -> (x = y?=w1877:bool)
                n1085 = case shown="True" w1877 {
                  tunnel: w1875 -> [_ w1880]
                  tunnel: w1874 -> [_ w1879]
                  frame False {
                  }
                  frame True {
                    n1086 = stacked-sequence {
                      tunnel: w1880 -> [w1882 _]
                      tunnel: w1879 -> [_ w1885]
                      frame #0 {
                        n1087 = Bundle(cluster=w1882, "STATUS"="END") -> (w1883:T4)  [unwired: 2 in]
                        n1088 = local write "LAB02-1 RUN"(FALSE) -> ()
                        n1089 = local write "LAB02-1 (DISP)"(w1883) -> ()
                      }
                      frame #1 {
                        n1090 = TDMS Close(11:w1885) -> (0:w1886:errorcluster)  [unwired: 1 in, 1 out]
                        n1091 = local write "data file error"(w1886) -> ()
                      }
                    }
                  }
                }
              }
              frame #3 {
                # "LAB02-2"
                n1092 = local read "LAB02-2 (DISP)"() -> (w1888:T4)
                n1093 = local read "LAB02-2 (TDMS)"() -> (w1887:refnum<k34>)
                n1094 = Unbundle(w1888) -> ("STATUS"=w1889:string)  [unwired: 2 out]
                n1095 = Equal?(x=w1889, y="STOP") -> (x = y?=w1890:bool)
                n1096 = case shown="True" w1890 {
                  tunnel: w1888 -> [_ w1893]
                  tunnel: w1887 -> [_ w1892]
                  frame False {
                  }
                  frame True {
                    n1097 = stacked-sequence {
                      tunnel: w1893 -> [w1895 _]
                      tunnel: w1892 -> [_ w1898]
                      frame #0 {
                        n1098 = Bundle(cluster=w1895, "STATUS"="END") -> (w1896:T4)  [unwired: 2 in]
                        n1099 = local write "LAB02-2 RUN"(FALSE) -> ()
                        n1100 = local write "LAB02-2 (DISP)"(w1896) -> ()
                      }
                      frame #1 {
                        n1101 = TDMS Close(11:w1898) -> (0:w1899:errorcluster)  [unwired: 1 in, 1 out]
                        n1102 = local write "data file error"(w1899) -> ()
                      }
                    }
                  }
                }
              }
              frame #4 {
                # "LAB03-1"
                n1103 = local read "LAB03-1 (DISP)"() -> (w1901:T4)
                n1104 = local read "LAB03-1 (TDMS)"() -> (w1900:refnum<k34>)
                n1105 = Unbundle(w1901) -> ("STATUS"=w1902:string)  [unwired: 2 out]
                n1106 = Equal?(x=w1902, y="STOP") -> (x = y?=w1903:bool)
                n1107 = case shown="True" w1903 {
                  tunnel: w1901 -> [_ w1906]
                  tunnel: w1900 -> [_ w1905]
                  frame False {
                  }
                  frame True {
                    n1108 = stacked-sequence {
                      tunnel: w1906 -> [w1908 _]
                      tunnel: w1905 -> [_ w1911]
                      frame #0 {
                        n1109 = Bundle(cluster=w1908, "STATUS"="END") -> (w1909:T4)  [unwired: 2 in]
                        n1110 = local write "LAB03-1 RUN"(FALSE) -> ()
                        n1111 = local write "LAB03-1 (DISP)"(w1909) -> ()
                      }
                      frame #1 {
                        n1112 = TDMS Close(11:w1911) -> (0:w1912:errorcluster)  [unwired: 1 in, 1 out]
                        n1113 = local write "data file error"(w1912) -> ()
                      }
                    }
                  }
                }
              }
              frame #5 {
                # "LAB03-2"
                n1114 = local read "LAB03-2 (DISP)"() -> (w1914:T4)
                n1115 = local read "LAB03-2 (TDMS)"() -> (w1913:refnum<k34>)
                n1116 = Unbundle(w1914) -> ("STATUS"=w1915:string)  [unwired: 2 out]
                n1117 = Equal?(x=w1915, y="STOP") -> (x = y?=w1916:bool)
                n1118 = case shown="True" w1916 {
                  tunnel: w1914 -> [_ w1919]
                  tunnel: w1913 -> [_ w1918]
                  frame False {
                  }
                  frame True {
                    n1119 = stacked-sequence {
                      tunnel: w1919 -> [w1921 _]
                      tunnel: w1918 -> [_ w1924]
                      frame #0 {
                        n1120 = Bundle(cluster=w1921, "STATUS"="END") -> (w1922:T4)  [unwired: 2 in]
                        n1121 = local write "LAB03-2 RUN"(FALSE) -> ()
                        n1122 = local write "LAB03-2 (DISP)"(w1922) -> ()
                      }
                      frame #1 {
                        n1123 = TDMS Close(11:w1924) -> (0:w1925:errorcluster)  [unwired: 1 in, 1 out]
                        n1124 = local write "data file error"(w1925) -> ()
                      }
                    }
                  }
                }
              }
              frame #6 {
                # "LAB04-1"
                n1125 = local read "LAB04-1 (DISP)"() -> (w1927:T4)
                n1126 = local read "LAB04-1 (TDMS)"() -> (w1926:refnum<k34>)
                n1127 = Unbundle(w1927) -> ("STATUS"=w1928:string)  [unwired: 2 out]
                n1128 = Equal?(x=w1928, y="STOP") -> (x = y?=w1929:bool)
                n1129 = case shown="True" w1929 {
                  tunnel: w1927 -> [_ w1932]
                  tunnel: w1926 -> [_ w1931]
                  frame False {
                  }
                  frame True {
                    n1130 = stacked-sequence {
                      tunnel: w1932 -> [w1934 _]
                      tunnel: w1931 -> [_ w1937]
                      frame #0 {
                        n1131 = Bundle(cluster=w1934, "STATUS"="END") -> (w1935:T4)  [unwired: 2 in]
                        n1132 = local write "LAB04-1 RUN"(FALSE) -> ()
                        n1133 = local write "LAB04-1 (DISP)"(w1935) -> ()
                      }
                      frame #1 {
                        n1134 = TDMS Close(11:w1937) -> (0:w1938:errorcluster)  [unwired: 1 in, 1 out]
                        n1135 = local write "data file error"(w1938) -> ()
                      }
                    }
                  }
                }
              }
              frame #7 {
                # "LAB04-2"
                n1136 = local read "LAB04-2 (DISP)"() -> (w1940:T4)
                n1137 = local read "LAB04-2 (TDMS)"() -> (w1939:refnum<k34>)
                n1138 = Unbundle(w1940) -> ("STATUS"=w1941:string)  [unwired: 2 out]
                n1139 = Equal?(x=w1941, y="STOP") -> (x = y?=w1942:bool)
                n1140 = case shown="True" w1942 {
                  tunnel: w1940 -> [_ w1945]
                  tunnel: w1939 -> [_ w1944]
                  frame False {
                  }
                  frame True {
                    n1141 = stacked-sequence {
                      tunnel: w1945 -> [w1947 _]
                      tunnel: w1944 -> [_ w1950]
                      frame #0 {
                        n1142 = Bundle(cluster=w1947, "STATUS"="END") -> (w1948:T4)  [unwired: 2 in]
                        n1143 = local write "LAB04-2 RUN"(FALSE) -> ()
                        n1144 = local write "LAB04-2 (DISP)"(w1948) -> ()
                      }
                      frame #1 {
                        n1145 = TDMS Close(11:w1950) -> (0:w1951:errorcluster)  [unwired: 1 in, 1 out]
                        n1146 = local write "data file error"(w1951) -> ()
                      }
                    }
                  }
                }
              }
              frame #8 {
                # "LAB05-1"
                n1147 = local read "LAB05-1 (DISP)"() -> (w1953:T4)
                n1148 = local read "LAB05-1 (TDMS)"() -> (w1952:refnum<k34>)
                n1149 = Unbundle(w1953) -> ("STATUS"=w1954:string)  [unwired: 2 out]
                n1150 = Equal?(x=w1954, y="STOP") -> (x = y?=w1955:bool)
                n1151 = case shown="True" w1955 {
                  tunnel: w1953 -> [_ w1958]
                  tunnel: w1952 -> [_ w1957]
                  frame False {
                  }
                  frame True {
                    n1152 = stacked-sequence {
                      tunnel: w1958 -> [w1960 _]
                      tunnel: w1957 -> [_ w1963]
                      frame #0 {
                        n1153 = Bundle(cluster=w1960, "STATUS"="END") -> (w1961:T4)  [unwired: 2 in]
                        n1154 = local write "LAB05-1 RUN"(FALSE) -> ()
                        n1155 = local write "LAB05-1 (DISP)"(w1961) -> ()
                      }
                      frame #1 {
                        n1156 = TDMS Close(11:w1963) -> (0:w1964:errorcluster)  [unwired: 1 in, 1 out]
                        n1157 = local write "data file error"(w1964) -> ()
                      }
                    }
                  }
                }
              }
              frame #9 {
                # "LAB05-2"
                n1158 = local read "LAB05-2 (DISP)"() -> (w1966:T4)
                n1159 = local read "LAB05-2 (TDMS)"() -> (w1965:refnum<k34>)
                n1160 = Unbundle(w1966) -> ("STATUS"=w1967:string)  [unwired: 2 out]
                n1161 = Equal?(x=w1967, y="STOP") -> (x = y?=w1968:bool)
                n1162 = case shown="True" w1968 {
                  tunnel: w1966 -> [_ w1971]
                  tunnel: w1965 -> [_ w1970]
                  frame False {
                  }
                  frame True {
                    n1163 = stacked-sequence {
                      tunnel: w1971 -> [w1973 _]
                      tunnel: w1970 -> [_ w1976]
                      frame #0 {
                        n1164 = Bundle(cluster=w1973, "STATUS"="END") -> (w1974:T4)  [unwired: 2 in]
                        n1165 = local write "LAB05-2 RUN"(FALSE) -> ()
                        n1166 = local write "LAB05-2 (DISP)"(w1974) -> ()
                      }
                      frame #1 {
                        n1167 = TDMS Close(11:w1976) -> (0:w1977:errorcluster)  [unwired: 1 in, 1 out]
                        n1168 = local write "data file error"(w1977) -> ()
                      }
                    }
                  }
                }
              }
            }
          }
          frame #8 {
            # "drive jigs"
            n1169 = stacked-sequence {
              frame #0 {
                # "jig on"
                n1170 = local read "jig cycle"() -> (w1978:dbl)
                n1171 = Equal?(x=w1978, y=0) -> (x = y?=w1980:bool)
                n1172 = case shown="True" w1980 {
                  frame False {
                  }
                  frame True {
                    n1173 = local read "LAB01-1RUN"() -> (w1981:bool)
                    n1174 = local read "LAB01-2 RUN"() -> (w1982:bool)
                    n1175 = local read "LAB03-1 RUN"() -> (w1988:bool)
                    n1176 = local read "LAB03-2 RUN"() -> (w1987:bool)
                    n1177 = local read "LAB02-1 RUN"() -> (w1990:bool)
                    n1178 = local read "LAB02-2 RUN"() -> (w1989:bool)
                    n1179 = local read "LAB04-1 RUN"() -> (w1986:bool)
                    n1180 = local read "LAB04-2 RUN"() -> (w1985:bool)
                    n1181 = local read "LAB05-1 RUN"() -> (w1984:bool)
                    n1182 = local read "LAB05-2 RUN"() -> (w1983:bool)
                    n1183 = local write "LAB05-1 (JIG)"(w1984) -> ()
                    n1184 = local write "LAB05-2 (JIG)"(w1983) -> ()
                    n1185 = local write "LAB04-2 (JIG)"(w1985) -> ()
                    n1186 = local write "LAB02-1 (JIG)"(w1990) -> ()
                    n1187 = local write "LAB03-1 (JIG)"(w1988) -> ()
                    n1188 = local write "LAB04-1 (JIG)"(w1986) -> ()
                    n1189 = local write "LAB03-2 (JIG)"(w1987) -> ()
                    n1190 = local write "LAB02-2 (JIG)"(w1989) -> ()
                    n1191 = local write "LAB01-1 (JIG)"(w1981) -> ()
                    n1192 = local write "LAB01-2 (JIG)"(w1982) -> ()
                  }
                }
              }
              frame #1 {
                # "jig off"
                n1193 = local read "jig cycle"() -> (w1993:dbl)
                n1194 = local read "on loops"() -> (w1992:dbl)
                n1195 = Equal?(x=w1993, y=w1992) -> (x = y?=w1991:bool)
                n1196 = case shown="True" w1991 {
                  frame False {
                  }
                  frame True {
                    w2044 = FALSE
                    w2045 = TRUE
                    w2043 = 2
                    n1197 = local read "LAB05-2 SELECT"() -> (w2034:T3)
                    n1198 = local read "LAB04-2 SELECT"() -> (w2036:T3)
                    n1199 = local read "LAB04-1 SELECT"() -> (w2037:T3)
                    n1200 = local read "LAB05-1 SELECT"() -> (w2035:T3)
                    n1201 = local read "LAB03-2 SELECT"() -> (w2038:T3)
                    n1202 = local read "LAB02-1 SELECT"() -> (w2041:T3)
                    n1203 = local read "LAB03-1 SELECT"() -> (w2039:T3)
                    n1204 = local read "LAB02-2 SELECT"() -> (w2040:T3)
                    n1205 = local read "LAB01-2 SELECT"() -> (w2042:T3)
                    n1206 = local read "LAB05-1 RUN"() -> (w2004:bool)
                    n1207 = local read "LAB05-2 RUN"() -> (w2003:bool)
                    n1208 = local read "LAB04-2 RUN"() -> (w2005:bool)
                    n1209 = local read "LAB04-1 RUN"() -> (w2006:bool)
                    n1210 = local read "LAB01-2 RUN"() -> (w2011:bool)
                    n1211 = local read "LAB03-2 RUN"() -> (w2007:bool)
                    n1212 = local read "LAB01-1RUN"() -> (w2022:bool)
                    n1213 = local read "LAB01-1 SELECT"() -> (w2046:T3)
                    n1214 = local read "LAB03-1 RUN"() -> (w2008:bool)
                    n1215 = local read "LAB02-1 RUN"() -> (w2010:bool)
                    n1216 = local read "LAB02-2 RUN"() -> (w2009:bool)
                    n1217 = Equal?(x=w2043, y=w2039) -> (x = y?=w2017:bool)
                    n1218 = Equal?(x=w2043, y=w2038) -> (x = y?=w2016:bool)
                    n1219 = Equal?(x=w2043, y=w2037) -> (x = y?=w2015:bool)
                    n1220 = Equal?(x=w2043, y=w2036) -> (x = y?=w2014:bool)
                    n1221 = Equal?(x=w2043, y=w2035) -> (x = y?=w2013:bool)
                    n1222 = Equal?(x=w2043, y=w2034) -> (x = y?=w2012:bool)
                    n1223 = Equal?(x=w2043, y=w2046) -> (x = y?=w2023:bool)
                    n1224 = Equal?(x=w2043, y=w2041) -> (x = y?=w2019:bool)
                    n1225 = Equal?(x=w2043, y=w2040) -> (x = y?=w2018:bool)
                    n1226 = Equal?(x=w2043, y=w2042) -> (x = y?=w2020:bool)
                    n1227 = And(x=w2014, y=w2005) -> (x .and. y?=w1996:bool)
                    n1228 = And(x=w2017, y=w2008) -> (x .and. y?=w1999:bool)
                    n1229 = And(x=w2015, y=w2006) -> (x .and. y?=w1997:bool)
                    n1230 = And(x=w2012, y=w2003) -> (x .and. y?=w1994:bool)
                    n1231 = And(x=w2018, y=w2009) -> (x .and. y?=w2000:bool)
                    n1232 = And(x=w2016, y=w2007) -> (x .and. y?=w1998:bool)
                    n1233 = And(x=w2013, y=w2004) -> (x .and. y?=w1995:bool)
                    n1234 = And(x=w2020, y=w2011) -> (x .and. y?=w2002:bool)
                    n1235 = And(x=w2023, y=w2022) -> (x .and. y?=w2021:bool)
                    n1236 = And(x=w2019, y=w2010) -> (x .and. y?=w2001:bool)
                    n1237 = Select(t=w2045, s=w2021, f=w2044) -> (s? t:f=w2024:bool)
                    n1238 = Select(t=w2045, s=w2002, f=w2044) -> (s? t:f=w2025:bool)
                    n1239 = Select(t=w2045, s=w2001, f=w2044) -> (s? t:f=w2026:bool)
                    n1240 = Select(t=w2045, s=w2000, f=w2044) -> (s? t:f=w2027:bool)
                    n1241 = Select(t=w2045, s=w1999, f=w2044) -> (s? t:f=w2028:bool)
                    n1242 = Select(t=w2045, s=w1998, f=w2044) -> (s? t:f=w2029:bool)
                    n1243 = Select(t=w2045, s=w1997, f=w2044) -> (s? t:f=w2030:bool)
                    n1244 = Select(t=w2045, s=w1996, f=w2044) -> (s? t:f=w2031:bool)
                    n1245 = Select(t=w2045, s=w1995, f=w2044) -> (s? t:f=w2032:bool)
                    n1246 = Select(t=w2045, s=w1994, f=w2044) -> (s? t:f=w2033:bool)
                    n1247 = local write "LAB03-2 (JIG)"(w2029) -> ()
                    n1248 = local write "LAB02-1 (JIG)"(w2026) -> ()
                    n1249 = local write "LAB02-2 (JIG)"(w2027) -> ()
                    n1250 = local write "LAB01-2 (JIG)"(w2025) -> ()
                    n1251 = local write "LAB03-1 (JIG)"(w2028) -> ()
                    n1252 = local write "LAB01-1 (JIG)"(w2024) -> ()
                    n1253 = local write "LAB05-2 (JIG)"(w2033) -> ()
                    n1254 = local write "LAB04-1 (JIG)"(w2030) -> ()
                    n1255 = local write "LAB05-1 (JIG)"(w2032) -> ()
                    n1256 = local write "LAB04-2 (JIG)"(w2031) -> ()
                  }
                }
              }
            }
          }
          frame #9 {
            # "drive digital output"
            n1257 = local read "LAB05-2 (O/I)"() -> (w2052:bool)
            n1258 = local read "LAB05-2 (JIG)"() -> (w2051:bool)
            n1259 = local read "LAB05-1 (O/I)"() -> (w2054:bool)
            n1260 = local read "LAB05-1 (JIG)"() -> (w2053:bool)
            n1261 = local read "LAB04-2 (O/I)"() -> (w2056:bool)
            n1262 = local read "LAB04-2 (JIG)"() -> (w2055:bool)
            n1263 = local read "LAB03-1 (O/I)"() -> (w2061:bool)
            n1264 = local read "LAB04-1 (O/I)"() -> (w2057:bool)
            n1265 = local read "LAB04-1 (JIG)"() -> (w2050:bool)
            n1266 = local read "LAB02-1 (O/I)"() -> (w2065:bool)
            n1267 = local read "LAB02-2 (O/I)"() -> (w2063:bool)
            n1268 = local read "LAB03-2 (O/I)"() -> (w2059:bool)
            n1269 = local read "LAB03-2 (JIG)"() -> (w2058:bool)
            n1270 = local read "LAB02-1 (JIG)"() -> (w2064:bool)
            n1271 = local read "LAB02-2 (JIG)"() -> (w2062:bool)
            n1272 = local read "LAB03-1 (JIG)"() -> (w2060:bool)
            n1273 = local read "LAB01-2 (O/I)"() -> (w2067:bool)
            n1274 = local read "LAB01-2 (JIG)"() -> (w2066:bool)
            n1275 = local read "LAB01-1 (O/I)"() -> (w2069:bool)
            n1276 = local read "LAB01-1 (JIG)"() -> (w2068:bool)
            n1277 = Build Array(w2056, w2055, w2054, w2053, w2052, w2051) -> (w2047:bool[])
            n1278 = Build Array(w2062, w2061, w2060, w2059, w2058, w2057, w2050) -> (w2048:bool[])
            n1279 = Build Array(w2069, w2068, w2067, w2066, w2065, w2064, w2063) -> (w2049:bool[])
            n1280 = call "sub vi - Drive Relays All v6.vi"("Array #2"=w2047, "Array #1"=w2048, "Array #0"=w2049) -> ()  [unwired: 8 in, 1 out]
          }
          frame #10 {
            # "get temperature values"
            n1281 = stacked-sequence {
              frame #0 {
                n1282 = local read "jig cycle"() -> (w2070:dbl)
                n1283 = local read "on loops"() -> (w2073:dbl)
                n1284 = local read "jig cycle"() -> (w2075:dbl)
                n1285 = Add(x=w2073, y=1) -> (x+y=w2074:dbl)
                n1286 = Equal?(x=w2075, y=0) -> (x = y?=w2076:bool)
                n1287 = Equal?(x=w2070, y=w2074) -> (x = y?=w2071:bool)
                n1288 = case shown="True" w2076 {
                  frame False {
                  }
                  frame True {
                    w2088 = FALSE
                    w2089 = TRUE
                    n1289 = local write "TEMP update"(TRUE) -> ()
                    n1290 = call "sub vi - GET ALL TEMP v3.vi"("LA01-EN"=w2089, "LA02-EN"=w2089, "LA03-EN"=w2089, "LA04-EN"=w2088, "LA05-EN"=w2088, "Gen Cal Value"=1.0) -> ("LA01 TEMP"=w2087:T14, "LA02 TEMP"=w2085:T14, "LA03 TEMP"=w2084:T14)  [unwired: 4 in, 3 out]
                    n1291 = local write "LAB03 TEMP"(w2084) -> ()
                    n1292 = local write "LAB02 TEMP"(w2085) -> ()
                    n1293 = local write "LAB01 TEMP"(w2087) -> ()
                  }
                }
                n1294 = case shown="True" w2071 {
                  frame False {
                  }
                  frame True {
                    w2081 = TRUE
                    w2082 = FALSE
                    n1295 = local write "TEMP update"(TRUE) -> ()
                    n1296 = call "sub vi - GET ALL TEMP v3.vi"("LA01-EN"=w2082, "LA02-EN"=w2082, "LA03-EN"=w2082, "LA04-EN"=w2081, "LA05-EN"=w2081, "Gen Cal Value"=1.0) -> ("LA04 TEMP"=w2079:T14, "LA05 TEMP"=w2078:T14)  [unwired: 4 in, 4 out]
                    n1297 = local write "LAB04 TEMP"(w2079) -> ()
                    n1298 = local write "LAB05 TEMP"(w2078) -> ()
                  }
                }
              }
              frame #1 {
                n1299 = local read "LAB01 (CAL)"() -> (w2107:T6)
                n1300 = local read "LAB01 TEMP"() -> (w2108:T9)
                n1301 = Unbundle By Name(w2108) -> ("T1 Live"=w2098:dbl, "T1 Neut"=w2097:dbl, "T2 Live"=w2096:dbl, "T2 Neut"=w2095:dbl)  [unwired: 2 out]
                n1302 = Unbundle By Name(w2107) -> ("1 (TL) cal"=w2094:dbl, "1 (TN) cal"=w2093:dbl, "2 (TL) cal"=w2092:dbl, "2 (TN) cal"=w2091:dbl)  [unwired: 6 out]
                n1303 = Multiply(x=w2098, y=w2094) -> (x*y=w2104:dbl)
                n1304 = Multiply(x=w2097, y=w2093) -> (x*y=w2103:dbl)
                n1305 = Multiply(x=w2096, y=w2092) -> (x*y=w2100:dbl)
                n1306 = Multiply(x=w2095, y=w2091) -> (x*y=w2099:dbl)
                n1307 = local read "LAB01-2 (SIG)"() -> (w2102:T2)
                n1308 = local read "LAB01-1 (SIG)"() -> (w2106:T2)
                n1309 = Bundle By Name(cluster=w2106, "Tmp Live"=w2104, "Tmp Neut"=w2103) -> (w2105:T2)
                n1310 = Bundle By Name(cluster=w2102, "Tmp Live"=w2100, "Tmp Neut"=w2099) -> (w2101:T2)
                n1311 = local write "LAB01-1 (SIG)"(w2105) -> ()
                n1312 = local write "LAB01-2 (SIG)"(w2101) -> ()
              }
              frame #2 {
                n1313 = local read "LAB02 (CAL)"() -> (w2125:T7)
                n1314 = local read "LAB02 TEMP"() -> (w2126:T9)
                n1315 = Unbundle By Name(w2126) -> ("T1 Live"=w2116:dbl, "T1 Neut"=w2115:dbl, "T2 Live"=w2114:dbl, "T2 Neut"=w2113:dbl)  [unwired: 2 out]
                n1316 = Unbundle By Name(w2125) -> ("1 (TL) cal"=w2112:dbl, "1 (TN) cal"=w2111:dbl, "2 (TL) cal"=w2110:dbl, "2 (TN) cal"=w2109:dbl)  [unwired: 6 out]
                n1317 = Multiply(x=w2116, y=w2112) -> (x*y=w2122:dbl)
                n1318 = Multiply(x=w2115, y=w2111) -> (x*y=w2121:dbl)
                n1319 = Multiply(x=w2114, y=w2110) -> (x*y=w2118:dbl)
                n1320 = Multiply(x=w2113, y=w2109) -> (x*y=w2117:dbl)
                n1321 = local read "LAB02-2 (SIG)"() -> (w2120:T2)
                n1322 = local read "LAB02-1 (SIG)"() -> (w2124:T2)
                n1323 = Bundle By Name(cluster=w2124, "Tmp Live"=w2122, "Tmp Neut"=w2121) -> (w2123:T2)
                n1324 = Bundle By Name(cluster=w2120, "Tmp Live"=w2118, "Tmp Neut"=w2117) -> (w2119:T2)
                n1325 = local write "LAB02-1 (SIG)"(w2123) -> ()
                n1326 = local write "LAB02-2 (SIG)"(w2119) -> ()
              }
              frame #3 {
                n1327 = local read "LAB03 (CAL)"() -> (w2143:T6)
                n1328 = local read "LAB03 TEMP"() -> (w2144:T9)
                n1329 = Unbundle By Name(w2144) -> ("T1 Live"=w2134:dbl, "T1 Neut"=w2133:dbl, "T2 Live"=w2132:dbl, "T2 Neut"=w2131:dbl)  [unwired: 2 out]
                n1330 = Unbundle By Name(w2143) -> ("1 (TL) cal"=w2130:dbl, "1 (TN) cal"=w2129:dbl, "2 (TL) cal"=w2128:dbl, "2 (TN) cal"=w2127:dbl)  [unwired: 6 out]
                n1331 = Multiply(x=w2134, y=w2130) -> (x*y=w2140:dbl)
                n1332 = Multiply(x=w2133, y=w2129) -> (x*y=w2139:dbl)
                n1333 = Multiply(x=w2132, y=w2128) -> (x*y=w2136:dbl)
                n1334 = Multiply(x=w2131, y=w2127) -> (x*y=w2135:dbl)
                n1335 = local read "LAB03-2 (SIG)"() -> (w2138:T2)
                n1336 = local read "LAB03-1 (SIG)"() -> (w2142:T2)
                n1337 = Bundle By Name(cluster=w2142, "Tmp Live"=w2140, "Tmp Neut"=w2139) -> (w2141:T2)
                n1338 = Bundle By Name(cluster=w2138, "Tmp Live"=w2136, "Tmp Neut"=w2135) -> (w2137:T2)
                n1339 = local write "LAB03-1 (SIG)"(w2141) -> ()
                n1340 = local write "LAB03-2 (SIG)"(w2137) -> ()
              }
              frame #4 {
                n1341 = local read "LAB04 (CAL)"() -> (w2161:T6)
                n1342 = local read "LAB04 TEMP"() -> (w2162:T9)
                n1343 = Unbundle By Name(w2162) -> ("T1 Live"=w2152:dbl, "T1 Neut"=w2151:dbl, "T2 Live"=w2150:dbl, "T2 Neut"=w2149:dbl)  [unwired: 2 out]
                n1344 = Unbundle By Name(w2161) -> ("1 (TL) cal"=w2148:dbl, "1 (TN) cal"=w2147:dbl, "2 (TL) cal"=w2146:dbl, "2 (TN) cal"=w2145:dbl)  [unwired: 6 out]
                n1345 = Multiply(x=w2152, y=w2148) -> (x*y=w2158:dbl)
                n1346 = Multiply(x=w2151, y=w2147) -> (x*y=w2157:dbl)
                n1347 = Multiply(x=w2150, y=w2146) -> (x*y=w2154:dbl)
                n1348 = Multiply(x=w2149, y=w2145) -> (x*y=w2153:dbl)
                n1349 = local read "LAB04-2 (SIG)"() -> (w2156:T2)
                n1350 = local read "LAB04-1 (SIG)"() -> (w2160:T2)
                n1351 = Bundle By Name(cluster=w2160, "Tmp Live"=w2158, "Tmp Neut"=w2157) -> (w2159:T2)
                n1352 = Bundle By Name(cluster=w2156, "Tmp Live"=w2154, "Tmp Neut"=w2153) -> (w2155:T2)
                n1353 = local write "LAB04-1 (SIG)"(w2159) -> ()
                n1354 = local write "LAB04-2 (SIG)"(w2155) -> ()
              }
              frame #5 {
                n1355 = local read "LAB05 (CAL)"() -> (w2179:T6)
                n1356 = local read "LAB05 TEMP"() -> (w2180:T9)
                n1357 = Unbundle By Name(w2180) -> ("T1 Live"=w2170:dbl, "T1 Neut"=w2169:dbl, "T2 Live"=w2168:dbl, "T2 Neut"=w2167:dbl)  [unwired: 2 out]
                n1358 = Unbundle By Name(w2179) -> ("1 (TL) cal"=w2166:dbl, "1 (TN) cal"=w2165:dbl, "2 (TL) cal"=w2164:dbl, "2 (TN) cal"=w2163:dbl)  [unwired: 6 out]
                n1359 = Multiply(x=w2170, y=w2166) -> (x*y=w2176:dbl)
                n1360 = Multiply(x=w2169, y=w2165) -> (x*y=w2175:dbl)
                n1361 = Multiply(x=w2168, y=w2164) -> (x*y=w2172:dbl)
                n1362 = Multiply(x=w2167, y=w2163) -> (x*y=w2171:dbl)
                n1363 = local read "LAB05-2 (SIG)"() -> (w2174:T2)
                n1364 = local read "LAB05-1 (SIG)"() -> (w2178:T2)
                n1365 = Bundle By Name(cluster=w2178, "Tmp Live"=w2176, "Tmp Neut"=w2175) -> (w2177:T2)
                n1366 = Bundle By Name(cluster=w2174, "Tmp Live"=w2172, "Tmp Neut"=w2171) -> (w2173:T2)
                n1367 = local write "LAB05-1 (SIG)"(w2177) -> ()
                n1368 = local write "LAB05-2 (SIG)"(w2173) -> ()
              }
            }
          }
          frame #11 {
            # "get analog values"
            n1369 = local read "on loops"() -> (w2187:dbl)
            n1370 = local read "jig cycle"() -> (w2184:dbl)
            n1371 = Add(x=w2187, y=2) -> (x+y=w2185:dbl)
            n1372 = Equal?(x=w2184, y=1) -> (x = y?=w2182:bool)
            n1373 = Equal?(x=w2184, y=w2185) -> (x = y?=w2183:bool)
            n1374 = Or(x=w2182, y=w2183) -> (x .or. y?=w2181:bool)
            n1375 = case shown="True" w2181 {
              frame False {
              }
              frame True {
                n1376 = call "sub vi - Read Analog All v8.vi"() -> ("Analog loop time"=w2195:dbl, "array GRAPH"=w2194:dynamicdata[], "LAB01"=w2193:T15, "LAB02"=w2192:T16, "LAB03"=w2191:T17, "LAB04"=w2190:T18, "array ERROR"=w2196:errorcluster[], "LAB05"=w2189:T19)  [unwired: 8 in]
                n1377 = stacked-sequence {
                  tunnel: w2196 -> [w2199 _ _ _ _ _]
                  tunnel: w2195 -> [w2198 _ _ _ _ _]
                  tunnel: w2194 -> [w2197 _ _ _ _ _]
                  tunnel: w2193 -> [_ w2244 _ _ _ _]
                  tunnel: w2192 -> [_ _ w2245 _ _ _]
                  tunnel: w2191 -> [_ _ _ w2269 _ _]
                  tunnel: w2190 -> [_ _ _ _ w2293 _]
                  tunnel: w2189 -> [_ _ _ _ _ w2317]
                  frame #0 {
                    n1378 = local write "AI update"(TRUE) -> ()
                    n1379 = Index Array(array=w2197, index=6) -> (element=→"LAB04-1 (GRAPH)":dynamicdata)
                    n1380 = Index Array(array=w2197, index=7) -> (element=→"LAB04-2 (GRAPH)":dynamicdata)
                    n1381 = Index Array(array=w2197, index=9) -> (element=→"LAB05-2 (GRAPH)":dynamicdata)
                    n1382 = Index Array(array=w2197, index=8) -> (element=→"LAB05-1 (GRAPH)":dynamicdata)
                    n1383 = Index Array(array=w2197, index=5) -> (element=→"LAB03-2 (GRAPH)":dynamicdata)
                    n1384 = Index Array(array=w2197, index=0) -> (element=→"LAB01-1 (GRAPH)":dynamicdata)
                    n1385 = Index Array(array=w2197, index=1) -> (element=→"LAB01-2 (GRAPH)":dynamicdata)
                    n1386 = Index Array(array=w2197, index=2) -> (element=→"LAB02-1 (GRAPH)":dynamicdata)
                    n1387 = Index Array(array=w2197, index=3) -> (element=→"LAB02-2 (GRAPH)":dynamicdata)
                    n1388 = Index Array(array=w2197, index=4) -> (element=→"LAB03-1 (GRAPH)":dynamicdata)
                    "AI loop time" <- w2198
                    "Analog Error Array" <- w2199
                  }
                  frame #1 {
                    n1389 = local read "LAB01 (CAL)"() -> (w2243:T6)
                    n1390 = Unbundle By Name(w2244) -> ("LAB01-1 (A)"=w2242:dbl, "LAB01-1 (V)"=w2241:dbl, "LAB01-1 (PF)"=w2240:dbl, "LAB01-2 (A)"=w2239:dbl, "LAB01-2 (V)"=w2238:dbl, "LAB01-2 (PF)"=w2237:dbl)
                    n1391 = Unbundle By Name(w2243) -> ("1  (A) cal"=w2236:dbl, "1 (V) cal"=w2235:dbl, "1 (PF) cal"=w2234:dbl, "2 (A) cal"=w2233:dbl, "2 (V) cal"=w2232:dbl, "2 (PF) cal"=w2231:dbl)  [unwired: 4 out]
                    n1392 = Multiply(x=w2242, y=w2236) -> (x*y=w2229:dbl)
                    n1393 = Multiply(x=w2241, y=w2235) -> (x*y=w2228:dbl)
                    n1394 = Multiply(x=w2240, y=w2234) -> (x*y=w2227:dbl)
                    n1395 = Multiply(x=w2239, y=w2233) -> (x*y=w2223:dbl)
                    n1396 = local read "LAB01-1 (SIG)"() -> (w2230:T2)
                    n1397 = Multiply(x=w2238, y=w2232) -> (x*y=w2222:dbl)
                    n1398 = Multiply(x=w2237, y=w2231) -> (x*y=w2221:dbl)
                    n1399 = local read "LAB01-2 (SIG)"() -> (w2225:T2)
                    n1400 = Bundle By Name(cluster=w2230, "AMPS"=w2229, "VOLTS"=w2228, "PF"=w2227) -> (w2226:T2)
                    n1401 = Bundle By Name(cluster=w2225, "AMPS"=w2223, "VOLTS"=w2222, "PF"=w2221) -> (w2224:T2)
                    n1402 = local write "LAB01-2 (SIG)"(w2224) -> ()
                    n1403 = local write "LAB01-1 (SIG)"(w2226) -> ()
                  }
                  frame #2 {
                    n1404 = local read "LAB02 (CAL)"() -> (w2268:T7)
                    n1405 = Unbundle By Name(w2245) -> ("LAB02-1 (A)"=w2267:dbl, "LAB02-1 (V)"=w2266:dbl, "LAB02-1 (PF)"=w2265:dbl, "LAB02-2 (A)"=w2264:dbl, "LAB02-2 (V)"=w2263:dbl, "LAB02-2 (PF)"=w2262:dbl)
                    n1406 = Unbundle By Name(w2268) -> ("1 (A) cal"=w2261:dbl, "1 (V) cal"=w2260:dbl, "1 (PF) cal"=w2259:dbl, "2 (A) cal"=w2258:dbl, "2 (V) cal"=w2257:dbl, "2 (PF) cal"=w2256:dbl)  [unwired: 4 out]
                    n1407 = Multiply(x=w2267, y=w2261) -> (x*y=w2254:dbl)
                    n1408 = Multiply(x=w2266, y=w2260) -> (x*y=w2253:dbl)
                    n1409 = Multiply(x=w2265, y=w2259) -> (x*y=w2252:dbl)
                    n1410 = Multiply(x=w2264, y=w2258) -> (x*y=w2248:dbl)
                    n1411 = local read "LAB02-1 (SIG)"() -> (w2255:T2)
                    n1412 = Multiply(x=w2263, y=w2257) -> (x*y=w2247:dbl)
                    n1413 = Multiply(x=w2262, y=w2256) -> (x*y=w2246:dbl)
                    n1414 = local read "LAB02-2 (SIG)"() -> (w2250:T2)
                    n1415 = Bundle By Name(cluster=w2255, "AMPS"=w2254, "VOLTS"=w2253, "PF"=w2252) -> (w2251:T2)
                    n1416 = Bundle By Name(cluster=w2250, "AMPS"=w2248, "VOLTS"=w2247, "PF"=w2246) -> (w2249:T2)
                    n1417 = local write "LAB02-2 (SIG)"(w2249) -> ()
                    n1418 = local write "LAB02-1 (SIG)"(w2251) -> ()
                  }
                  frame #3 {
                    n1419 = local read "LAB03 (CAL)"() -> (w2292:T6)
                    n1420 = Unbundle By Name(w2269) -> ("LAB03-1 (A)"=w2291:dbl, "LAB03-1 (V)"=w2290:dbl, "LAB03-1 (PF)"=w2289:dbl, "LAB03-2 (A)"=w2288:dbl, "LAB03-2 (V)"=w2287:dbl, "LAB03-2 (PF)"=w2286:dbl)
                    n1421 = Unbundle By Name(w2292) -> ("1  (A) cal"=w2285:dbl, "1 (V) cal"=w2284:dbl, "1 (PF) cal"=w2283:dbl, "2 (A) cal"=w2282:dbl, "2 (V) cal"=w2281:dbl, "2 (PF) cal"=w2280:dbl)  [unwired: 4 out]
                    n1422 = Multiply(x=w2291, y=w2285) -> (x*y=w2278:dbl)
                    n1423 = Multiply(x=w2290, y=w2284) -> (x*y=w2277:dbl)
                    n1424 = Multiply(x=w2289, y=w2283) -> (x*y=w2276:dbl)
                    n1425 = Multiply(x=w2288, y=w2282) -> (x*y=w2272:dbl)
                    n1426 = local read "LAB03-1 (SIG)"() -> (w2279:T2)
                    n1427 = Multiply(x=w2287, y=w2281) -> (x*y=w2271:dbl)
                    n1428 = Multiply(x=w2286, y=w2280) -> (x*y=w2270:dbl)
                    n1429 = local read "LAB03-1 (SIG)"() -> (w2274:T2)
                    n1430 = Bundle By Name(cluster=w2279, "AMPS"=w2278, "VOLTS"=w2277, "PF"=w2276) -> (w2275:T2)
                    n1431 = Bundle By Name(cluster=w2274, "AMPS"=w2272, "VOLTS"=w2271, "PF"=w2270) -> (w2273:T2)
                    n1432 = local write "LAB03-1 (SIG)"(w2273) -> ()
                    n1433 = local write "LAB03-1 (SIG)"(w2275) -> ()
                  }
                  frame #4 {
                    n1434 = local read "LAB04 (CAL)"() -> (w2316:T6)
                    n1435 = Unbundle By Name(w2293) -> ("LAB04-1 (A)"=w2315:dbl, "LAB04-1 (V)"=w2314:dbl, "LAB04-1 (PF)"=w2313:dbl, "LAB04-2 (A)"=w2312:dbl, "LAB04-2 (V)"=w2311:dbl, "LAB04-2 (PF)"=w2310:dbl)
                    n1436 = Unbundle By Name(w2316) -> ("1  (A) cal"=w2309:dbl, "1 (V) cal"=w2308:dbl, "1 (PF) cal"=w2307:dbl, "2 (A) cal"=w2306:dbl, "2 (V) cal"=w2305:dbl, "2 (PF) cal"=w2304:dbl)  [unwired: 4 out]
                    n1437 = Multiply(x=w2315, y=w2309) -> (x*y=w2302:dbl)
                    n1438 = Multiply(x=w2314, y=w2308) -> (x*y=w2301:dbl)
                    n1439 = Multiply(x=w2313, y=w2307) -> (x*y=w2300:dbl)
                    n1440 = Multiply(x=w2312, y=w2306) -> (x*y=w2296:dbl)
                    n1441 = local read "LAB04-1 (SIG)"() -> (w2303:T2)
                    n1442 = Multiply(x=w2311, y=w2305) -> (x*y=w2295:dbl)
                    n1443 = Multiply(x=w2310, y=w2304) -> (x*y=w2294:dbl)
                    n1444 = local read "LAB04-2 (SIG)"() -> (w2298:T2)
                    n1445 = Bundle By Name(cluster=w2303, "AMPS"=w2302, "VOLTS"=w2301, "PF"=w2300) -> (w2299:T2)
                    n1446 = Bundle By Name(cluster=w2298, "AMPS"=w2296, "VOLTS"=w2295, "PF"=w2294) -> (w2297:T2)
                    n1447 = local write "LAB04-2 (SIG)"(w2297) -> ()
                    n1448 = local write "LAB04-1 (SIG)"(w2299) -> ()
                  }
                  frame #5 {
                    n1449 = local read "LAB05 (CAL)"() -> (w2340:T6)
                    n1450 = Unbundle By Name(w2317) -> ("LAB05-1 (A)"=w2339:dbl, "LAB05-1 (V)"=w2338:dbl, "LAB05-1 (PF)"=w2337:dbl, "LAB05-2 (A)"=w2336:dbl, "LAB05-2 (V)"=w2335:dbl, "LAB05-2 (PF)"=w2334:dbl)
                    n1451 = Unbundle By Name(w2340) -> ("1  (A) cal"=w2333:dbl, "1 (V) cal"=w2332:dbl, "1 (PF) cal"=w2331:dbl, "2 (A) cal"=w2330:dbl, "2 (V) cal"=w2329:dbl, "2 (PF) cal"=w2328:dbl)  [unwired: 4 out]
                    n1452 = Multiply(x=w2339, y=w2333) -> (x*y=w2326:dbl)
                    n1453 = Multiply(x=w2338, y=w2332) -> (x*y=w2325:dbl)
                    n1454 = Multiply(x=w2337, y=w2331) -> (x*y=w2324:dbl)
                    n1455 = Multiply(x=w2336, y=w2330) -> (x*y=w2320:dbl)
                    n1456 = local read "LAB05-1 (SIG)"() -> (w2327:T2)
                    n1457 = Multiply(x=w2335, y=w2329) -> (x*y=w2319:dbl)
                    n1458 = Multiply(x=w2334, y=w2328) -> (x*y=w2318:dbl)
                    n1459 = local read "LAB05-2 (SIG)"() -> (w2322:T2)
                    n1460 = Bundle By Name(cluster=w2327, "AMPS"=w2326, "VOLTS"=w2325, "PF"=w2324) -> (w2323:T2)
                    n1461 = Bundle By Name(cluster=w2322, "AMPS"=w2320, "VOLTS"=w2319, "PF"=w2318) -> (w2321:T2)
                    n1462 = local write "LAB05-2 (SIG)"(w2321) -> ()
                    n1463 = local write "LAB05-1 (SIG)"(w2323) -> ()
                  }
                }
              }
            }
          }
          frame #12 {
            # "save test data to file"
            n1464 = local read "on loops"() -> (w2357:dbl)
            n1465 = local read "jig cycle"() -> (w2354:dbl)
            n1466 = Add(x=w2357, y=2) -> (x+y=w2355:dbl)
            n1467 = Equal?(x=w2354, y=1) -> (x = y?=w2352:bool)
            n1468 = Equal?(x=w2354, y=w2355) -> (x = y?=w2353:bool)
            n1469 = Or(x=w2352, y=w2353) -> (x .or. y?=w2351:bool)
            n1470 = case shown="True" w2351 {
              tunnel: w2350 -> [_ w2368]
              tunnel: w2349 -> [_ w2367]
              tunnel: w2348 -> [_ w2366]
              tunnel: w2347 -> [_ w2365]
              tunnel: w2346 -> [_ w2364]
              tunnel: w2345 -> [_ w2363]
              tunnel: w2344 -> [_ w2362]
              tunnel: w2343 -> [_ w2361]
              tunnel: w2342 -> [_ w2360]
              tunnel: w2341 -> [_ w2359]
              frame False {
              }
              frame True {
                n1471 = stacked-sequence {
                  tunnel: w2368 -> [w2369 _ _ _ _ _ _ _ _ _]
                  tunnel: w2367 -> [_ w2414 _ _ _ _ _ _ _ _]
                  tunnel: w2366 -> [_ _ w2459 _ _ _ _ _ _ _]
                  tunnel: w2365 -> [_ _ _ w2504 _ _ _ _ _ _]
                  tunnel: w2364 -> [_ _ _ _ w2549 _ _ _ _ _]
                  tunnel: w2363 -> [_ _ _ _ _ w2594 _ _ _ _]
                  tunnel: w2362 -> [_ _ _ _ _ _ w2639 _ _ _]
                  tunnel: w2361 -> [_ _ _ _ _ _ _ w2684 _ _]
                  tunnel: w2360 -> [_ _ _ _ _ _ _ _ w2729 _]
                  tunnel: w2359 -> [_ _ _ _ _ _ _ _ _ w2774]
                  frame #0 {
                    # "LAB01-1"
                    n1472 = case shown="True" w2369 {
                      frame False {
                      }
                      frame True {
                        n1473 = local read "LAB01-1 (DISP)"() -> (w2411:T4)
                        n1474 = local read "LAB01-1 (SIG)"() -> (w2412:T2)
                        n1475 = local read "LAB01-1 (TDMS)"() -> (w2413:refnum<k34>)
                        n1476 = Build Array("TEMP Neut") -> (w2377:string[])
                        n1477 = Build Array("CYCLE") -> (w2372:string[])
                        n1478 = Build Array("TEMP Live") -> (w2382:string[])
                        n1479 = Build Array("PF") -> (w2387:string[])
                        n1480 = Build Array("AMPS") -> (w2408:string[])
                        n1481 = Build Array("VOLTS") -> (w2399:string[])
                        n1482 = Unbundle(w2412) -> ("AMPS"=w2407:dbl, "VOLTS"=w2396:dbl, "PF"=w2395:dbl, "Tmp Live"=w2394:dbl, "Tmp Neut"=w2397:dbl)
                        n1483 = Unbundle(w2411) -> ("CYCLE"=w2392:dbl)  [unwired: 2 out]
                        n1484 = Build Array(w2396) -> (w2393:dbl[])
                        n1485 = Build Array(w2395) -> (w2386:dbl[])
                        n1486 = Build Array(w2394) -> (w2381:dbl[])
                        n1487 = Build Array(w2397) -> (w2376:dbl[])
                        n1488 = Build Array(w2407) -> (w2406:dbl[])
                        n1489 = Build Array(w2392) -> (w2371:dbl[])
                        n1490 = TDMS Write(0:w2413, 5:"LAB01-1 TEST VALUES", 7:w2408, 9:w2406) -> (4:w2401:refnum<k34>, 6:w2400:string, 15:w2388:errorcluster)  [unwired: 2 in, 1 out]
                        n1491 = TDMS Write(0:w2401, 5:w2400, 7:w2399, 9:w2393, 11:w2388) -> (4:w2391:refnum<k34>, 6:w2390:string, 15:w2389:errorcluster)  [unwired: 1 in, 1 out]
                        n1492 = TDMS Write(0:w2391, 5:w2390, 7:w2387, 9:w2386, 11:w2389) -> (4:w2385:refnum<k34>, 6:w2384:string, 15:w2383:errorcluster)  [unwired: 1 in, 1 out]
                        n1493 = TDMS Write(0:w2385, 5:w2384, 7:w2382, 9:w2381, 11:w2383) -> (4:w2380:refnum<k34>, 6:w2379:string, 15:w2378:errorcluster)  [unwired: 1 in, 1 out]
                        n1494 = TDMS Write(0:w2380, 5:w2379, 7:w2377, 9:w2376, 11:w2378) -> (4:w2375:refnum<k34>, 6:w2374:string, 15:w2373:errorcluster)  [unwired: 1 in, 1 out]
                        n1495 = TDMS Write(0:w2375, 5:w2374, 7:w2372, 9:w2371, 11:w2373) -> (15:w2370:errorcluster)  [unwired: 1 in, 3 out]
                        n1496 = local write "data file error"(w2370) -> ()
                      }
                    }
                  }
                  frame #1 {
                    # "LAB01-2"
                    n1497 = case shown="True" w2414 {
                      frame False {
                      }
                      frame True {
                        n1498 = local read "LAB01-2 (DISP)"() -> (w2456:T4)
                        n1499 = local read "LAB01-2 (SIG)"() -> (w2457:T2)
                        n1500 = local read "LAB01-2 (TDMS)"() -> (w2458:refnum<k34>)
                        n1501 = Build Array("TEMP Neut") -> (w2422:string[])
                        n1502 = Build Array("CYCLE") -> (w2417:string[])
                        n1503 = Build Array("TEMP Live") -> (w2427:string[])
                        n1504 = Build Array("PF") -> (w2432:string[])
                        n1505 = Build Array("AMPS") -> (w2453:string[])
                        n1506 = Build Array("VOLTS") -> (w2444:string[])
                        n1507 = Unbundle(w2457) -> ("AMPS"=w2452:dbl, "VOLTS"=w2441:dbl, "PF"=w2440:dbl, "Tmp Live"=w2439:dbl, "Tmp Neut"=w2442:dbl)
                        n1508 = Unbundle(w2456) -> ("CYCLE"=w2437:dbl)  [unwired: 2 out]
                        n1509 = Build Array(w2441) -> (w2438:dbl[])
                        n1510 = Build Array(w2440) -> (w2431:dbl[])
                        n1511 = Build Array(w2439) -> (w2426:dbl[])
                        n1512 = Build Array(w2442) -> (w2421:dbl[])
                        n1513 = Build Array(w2452) -> (w2451:dbl[])
                        n1514 = Build Array(w2437) -> (w2416:dbl[])
                        n1515 = TDMS Write(0:w2458, 5:"LAB01-2 TEST VALUES", 7:w2453, 9:w2451) -> (4:w2446:refnum<k34>, 6:w2445:string, 15:w2433:errorcluster)  [unwired: 2 in, 1 out]
                        n1516 = TDMS Write(0:w2446, 5:w2445, 7:w2444, 9:w2438, 11:w2433) -> (4:w2436:refnum<k34>, 6:w2435:string, 15:w2434:errorcluster)  [unwired: 1 in, 1 out]
                        n1517 = TDMS Write(0:w2436, 5:w2435, 7:w2432, 9:w2431, 11:w2434) -> (4:w2430:refnum<k34>, 6:w2429:string, 15:w2428:errorcluster)  [unwired: 1 in, 1 out]
                        n1518 = TDMS Write(0:w2430, 5:w2429, 7:w2427, 9:w2426, 11:w2428) -> (4:w2425:refnum<k34>, 6:w2424:string, 15:w2423:errorcluster)  [unwired: 1 in, 1 out]
                        n1519 = TDMS Write(0:w2425, 5:w2424, 7:w2422, 9:w2421, 11:w2423) -> (4:w2420:refnum<k34>, 6:w2419:string, 15:w2418:errorcluster)  [unwired: 1 in, 1 out]
                        n1520 = TDMS Write(0:w2420, 5:w2419, 7:w2417, 9:w2416, 11:w2418) -> (15:w2415:errorcluster)  [unwired: 1 in, 3 out]
                        n1521 = local write "data file error"(w2415) -> ()
                      }
                    }
                  }
                  frame #2 {
                    # "LAB02-1"
                    n1522 = case shown="True" w2459 {
                      frame False {
                      }
                      frame True {
                        n1523 = local read "LAB02-1 (DISP)"() -> (w2501:T4)
                        n1524 = local read "LAB02-1 (SIG)"() -> (w2502:T2)
                        n1525 = local read "LAB02-1 (TDMS)"() -> (w2503:refnum<k34>)
                        n1526 = Build Array("TEMP Neut") -> (w2467:string[])
                        n1527 = Build Array("CYCLE") -> (w2462:string[])
                        n1528 = Build Array("TEMP Live") -> (w2472:string[])
                        n1529 = Build Array("PF") -> (w2477:string[])
                        n1530 = Build Array("AMPS") -> (w2498:string[])
                        n1531 = Build Array("VOLTS") -> (w2489:string[])
                        n1532 = Unbundle(w2502) -> ("AMPS"=w2497:dbl, "VOLTS"=w2486:dbl, "PF"=w2485:dbl, "Tmp Live"=w2484:dbl, "Tmp Neut"=w2487:dbl)
                        n1533 = Unbundle(w2501) -> ("CYCLE"=w2482:dbl)  [unwired: 2 out]
                        n1534 = Build Array(w2486) -> (w2483:dbl[])
                        n1535 = Build Array(w2485) -> (w2476:dbl[])
                        n1536 = Build Array(w2484) -> (w2471:dbl[])
                        n1537 = Build Array(w2487) -> (w2466:dbl[])
                        n1538 = Build Array(w2497) -> (w2496:dbl[])
                        n1539 = Build Array(w2482) -> (w2461:dbl[])
                        n1540 = TDMS Write(0:w2503, 5:"LAB02-1 TEST VALUES", 7:w2498, 9:w2496) -> (4:w2491:refnum<k34>, 6:w2490:string, 15:w2478:errorcluster)  [unwired: 2 in, 1 out]
                        n1541 = TDMS Write(0:w2491, 5:w2490, 7:w2489, 9:w2483, 11:w2478) -> (4:w2481:refnum<k34>, 6:w2480:string, 15:w2479:errorcluster)  [unwired: 1 in, 1 out]
                        n1542 = TDMS Write(0:w2481, 5:w2480, 7:w2477, 9:w2476, 11:w2479) -> (4:w2475:refnum<k34>, 6:w2474:string, 15:w2473:errorcluster)  [unwired: 1 in, 1 out]
                        n1543 = TDMS Write(0:w2475, 5:w2474, 7:w2472, 9:w2471, 11:w2473) -> (4:w2470:refnum<k34>, 6:w2469:string, 15:w2468:errorcluster)  [unwired: 1 in, 1 out]
                        n1544 = TDMS Write(0:w2470, 5:w2469, 7:w2467, 9:w2466, 11:w2468) -> (4:w2465:refnum<k34>, 6:w2464:string, 15:w2463:errorcluster)  [unwired: 1 in, 1 out]
                        n1545 = TDMS Write(0:w2465, 5:w2464, 7:w2462, 9:w2461, 11:w2463) -> (15:w2460:errorcluster)  [unwired: 1 in, 3 out]
                        n1546 = local write "data file error"(w2460) -> ()
                      }
                    }
                  }
                  frame #3 {
                    # "LAB02-2"
                    n1547 = case shown="True" w2504 {
                      frame False {
                      }
                      frame True {
                        n1548 = local read "LAB02-2 (DISP)"() -> (w2546:T4)
                        n1549 = local read "LAB02-2 (SIG)"() -> (w2547:T2)
                        n1550 = local read "LAB02-2 (TDMS)"() -> (w2548:refnum<k34>)
                        n1551 = Build Array("TEMP Neut") -> (w2512:string[])
                        n1552 = Build Array("CYCLE") -> (w2507:string[])
                        n1553 = Build Array("TEMP Live") -> (w2517:string[])
                        n1554 = Build Array("PF") -> (w2522:string[])
                        n1555 = Build Array("AMPS") -> (w2543:string[])
                        n1556 = Build Array("VOLTS") -> (w2534:string[])
                        n1557 = Unbundle(w2547) -> ("AMPS"=w2542:dbl, "VOLTS"=w2531:dbl, "PF"=w2530:dbl, "Tmp Live"=w2529:dbl, "Tmp Neut"=w2532:dbl)
                        n1558 = Unbundle(w2546) -> ("CYCLE"=w2527:dbl)  [unwired: 2 out]
                        n1559 = Build Array(w2531) -> (w2528:dbl[])
                        n1560 = Build Array(w2530) -> (w2521:dbl[])
                        n1561 = Build Array(w2529) -> (w2516:dbl[])
                        n1562 = Build Array(w2532) -> (w2511:dbl[])
                        n1563 = Build Array(w2542) -> (w2541:dbl[])
                        n1564 = Build Array(w2527) -> (w2506:dbl[])
                        n1565 = TDMS Write(0:w2548, 5:"LAB02-2 TEST VALUES", 7:w2543, 9:w2541) -> (4:w2536:refnum<k34>, 6:w2535:string, 15:w2523:errorcluster)  [unwired: 2 in, 1 out]
                        n1566 = TDMS Write(0:w2536, 5:w2535, 7:w2534, 9:w2528, 11:w2523) -> (4:w2526:refnum<k34>, 6:w2525:string, 15:w2524:errorcluster)  [unwired: 1 in, 1 out]
                        n1567 = TDMS Write(0:w2526, 5:w2525, 7:w2522, 9:w2521, 11:w2524) -> (4:w2520:refnum<k34>, 6:w2519:string, 15:w2518:errorcluster)  [unwired: 1 in, 1 out]
                        n1568 = TDMS Write(0:w2520, 5:w2519, 7:w2517, 9:w2516, 11:w2518) -> (4:w2515:refnum<k34>, 6:w2514:string, 15:w2513:errorcluster)  [unwired: 1 in, 1 out]
                        n1569 = TDMS Write(0:w2515, 5:w2514, 7:w2512, 9:w2511, 11:w2513) -> (4:w2510:refnum<k34>, 6:w2509:string, 15:w2508:errorcluster)  [unwired: 1 in, 1 out]
                        n1570 = TDMS Write(0:w2510, 5:w2509, 7:w2507, 9:w2506, 11:w2508) -> (15:w2505:errorcluster)  [unwired: 1 in, 3 out]
                        n1571 = local write "data file error"(w2505) -> ()
                      }
                    }
                  }
                  frame #4 {
                    # "LAB03-1"
                    n1572 = case shown="True" w2549 {
                      frame False {
                      }
                      frame True {
                        n1573 = local read "LAB03-1 (DISP)"() -> (w2591:T4)
                        n1574 = local read "LAB03-1 (SIG)"() -> (w2592:T2)
                        n1575 = local read "LAB03-1 (TDMS)"() -> (w2593:refnum<k34>)
                        n1576 = Build Array("TEMP Neut") -> (w2557:string[])
                        n1577 = Build Array("CYCLE") -> (w2552:string[])
                        n1578 = Build Array("TEMP Live") -> (w2562:string[])
                        n1579 = Build Array("PF") -> (w2567:string[])
                        n1580 = Build Array("AMPS") -> (w2588:string[])
                        n1581 = Build Array("VOLTS") -> (w2579:string[])
                        n1582 = Unbundle(w2592) -> ("AMPS"=w2587:dbl, "VOLTS"=w2576:dbl, "PF"=w2575:dbl, "Tmp Live"=w2574:dbl, "Tmp Neut"=w2577:dbl)
                        n1583 = Unbundle(w2591) -> ("CYCLE"=w2572:dbl)  [unwired: 2 out]
                        n1584 = Build Array(w2576) -> (w2573:dbl[])
                        n1585 = Build Array(w2575) -> (w2566:dbl[])
                        n1586 = Build Array(w2574) -> (w2561:dbl[])
                        n1587 = Build Array(w2577) -> (w2556:dbl[])
                        n1588 = Build Array(w2587) -> (w2586:dbl[])
                        n1589 = Build Array(w2572) -> (w2551:dbl[])
                        n1590 = TDMS Write(0:w2593, 5:"LAB03-1 TEST VALUES", 7:w2588, 9:w2586) -> (4:w2581:refnum<k34>, 6:w2580:string, 15:w2568:errorcluster)  [unwired: 2 in, 1 out]
                        n1591 = TDMS Write(0:w2581, 5:w2580, 7:w2579, 9:w2573, 11:w2568) -> (4:w2571:refnum<k34>, 6:w2570:string, 15:w2569:errorcluster)  [unwired: 1 in, 1 out]
                        n1592 = TDMS Write(0:w2571, 5:w2570, 7:w2567, 9:w2566, 11:w2569) -> (4:w2565:refnum<k34>, 6:w2564:string, 15:w2563:errorcluster)  [unwired: 1 in, 1 out]
                        n1593 = TDMS Write(0:w2565, 5:w2564, 7:w2562, 9:w2561, 11:w2563) -> (4:w2560:refnum<k34>, 6:w2559:string, 15:w2558:errorcluster)  [unwired: 1 in, 1 out]
                        n1594 = TDMS Write(0:w2560, 5:w2559, 7:w2557, 9:w2556, 11:w2558) -> (4:w2555:refnum<k34>, 6:w2554:string, 15:w2553:errorcluster)  [unwired: 1 in, 1 out]
                        n1595 = TDMS Write(0:w2555, 5:w2554, 7:w2552, 9:w2551, 11:w2553) -> (15:w2550:errorcluster)  [unwired: 1 in, 3 out]
                        n1596 = local write "data file error"(w2550) -> ()
                      }
                    }
                  }
                  frame #5 {
                    # "LAB03-2"
                    n1597 = case shown="True" w2594 {
                      frame False {
                      }
                      frame True {
                        n1598 = local read "LAB03-2 (DISP)"() -> (w2636:T4)
                        n1599 = local read "LAB03-2 (SIG)"() -> (w2637:T2)
                        n1600 = local read "LAB03-2 (TDMS)"() -> (w2638:refnum<k34>)
                        n1601 = Build Array("TEMP Neut") -> (w2602:string[])
                        n1602 = Build Array("CYCLE") -> (w2597:string[])
                        n1603 = Build Array("TEMP Live") -> (w2607:string[])
                        n1604 = Build Array("PF") -> (w2612:string[])
                        n1605 = Build Array("AMPS") -> (w2633:string[])
                        n1606 = Build Array("VOLTS") -> (w2624:string[])
                        n1607 = Unbundle(w2637) -> ("AMPS"=w2632:dbl, "VOLTS"=w2621:dbl, "PF"=w2620:dbl, "Tmp Live"=w2619:dbl, "Tmp Neut"=w2622:dbl)
                        n1608 = Unbundle(w2636) -> ("CYCLE"=w2617:dbl)  [unwired: 2 out]
                        n1609 = Build Array(w2621) -> (w2618:dbl[])
                        n1610 = Build Array(w2620) -> (w2611:dbl[])
                        n1611 = Build Array(w2619) -> (w2606:dbl[])
                        n1612 = Build Array(w2622) -> (w2601:dbl[])
                        n1613 = Build Array(w2632) -> (w2631:dbl[])
                        n1614 = Build Array(w2617) -> (w2596:dbl[])
                        n1615 = TDMS Write(0:w2638, 5:"LAB03-2 TEST VALUES", 7:w2633, 9:w2631) -> (4:w2626:refnum<k34>, 6:w2625:string, 15:w2613:errorcluster)  [unwired: 2 in, 1 out]
                        n1616 = TDMS Write(0:w2626, 5:w2625, 7:w2624, 9:w2618, 11:w2613) -> (4:w2616:refnum<k34>, 6:w2615:string, 15:w2614:errorcluster)  [unwired: 1 in, 1 out]
                        n1617 = TDMS Write(0:w2616, 5:w2615, 7:w2612, 9:w2611, 11:w2614) -> (4:w2610:refnum<k34>, 6:w2609:string, 15:w2608:errorcluster)  [unwired: 1 in, 1 out]
                        n1618 = TDMS Write(0:w2610, 5:w2609, 7:w2607, 9:w2606, 11:w2608) -> (4:w2605:refnum<k34>, 6:w2604:string, 15:w2603:errorcluster)  [unwired: 1 in, 1 out]
                        n1619 = TDMS Write(0:w2605, 5:w2604, 7:w2602, 9:w2601, 11:w2603) -> (4:w2600:refnum<k34>, 6:w2599:string, 15:w2598:errorcluster)  [unwired: 1 in, 1 out]
                        n1620 = TDMS Write(0:w2600, 5:w2599, 7:w2597, 9:w2596, 11:w2598) -> (15:w2595:errorcluster)  [unwired: 1 in, 3 out]
                        n1621 = local write "data file error"(w2595) -> ()
                      }
                    }
                  }
                  frame #6 {
                    # "LAB04-1"
                    n1622 = case shown="True" w2639 {
                      frame False {
                      }
                      frame True {
                        n1623 = local read "LAB04-1 (DISP)"() -> (w2681:T4)
                        n1624 = local read "LAB04-1 (SIG)"() -> (w2682:T2)
                        n1625 = local read "LAB04-1 (TDMS)"() -> (w2683:refnum<k34>)
                        n1626 = Build Array("TEMP Neut") -> (w2647:string[])
                        n1627 = Build Array("CYCLE") -> (w2642:string[])
                        n1628 = Build Array("TEMP Live") -> (w2652:string[])
                        n1629 = Build Array("PF") -> (w2657:string[])
                        n1630 = Build Array("AMPS") -> (w2678:string[])
                        n1631 = Build Array("VOLTS") -> (w2669:string[])
                        n1632 = Unbundle(w2682) -> ("AMPS"=w2677:dbl, "VOLTS"=w2666:dbl, "PF"=w2665:dbl, "Tmp Live"=w2664:dbl, "Tmp Neut"=w2667:dbl)
                        n1633 = Unbundle(w2681) -> ("CYCLE"=w2662:dbl)  [unwired: 2 out]
                        n1634 = Build Array(w2666) -> (w2663:dbl[])
                        n1635 = Build Array(w2665) -> (w2656:dbl[])
                        n1636 = Build Array(w2664) -> (w2651:dbl[])
                        n1637 = Build Array(w2667) -> (w2646:dbl[])
                        n1638 = Build Array(w2677) -> (w2676:dbl[])
                        n1639 = Build Array(w2662) -> (w2641:dbl[])
                        n1640 = TDMS Write(0:w2683, 5:"LAB04-1 TEST VALUES", 7:w2678, 9:w2676) -> (4:w2671:refnum<k34>, 6:w2670:string, 15:w2658:errorcluster)  [unwired: 2 in, 1 out]
                        n1641 = TDMS Write(0:w2671, 5:w2670, 7:w2669, 9:w2663, 11:w2658) -> (4:w2661:refnum<k34>, 6:w2660:string, 15:w2659:errorcluster)  [unwired: 1 in, 1 out]
                        n1642 = TDMS Write(0:w2661, 5:w2660, 7:w2657, 9:w2656, 11:w2659) -> (4:w2655:refnum<k34>, 6:w2654:string, 15:w2653:errorcluster)  [unwired: 1 in, 1 out]
                        n1643 = TDMS Write(0:w2655, 5:w2654, 7:w2652, 9:w2651, 11:w2653) -> (4:w2650:refnum<k34>, 6:w2649:string, 15:w2648:errorcluster)  [unwired: 1 in, 1 out]
                        n1644 = TDMS Write(0:w2650, 5:w2649, 7:w2647, 9:w2646, 11:w2648) -> (4:w2645:refnum<k34>, 6:w2644:string, 15:w2643:errorcluster)  [unwired: 1 in, 1 out]
                        n1645 = TDMS Write(0:w2645, 5:w2644, 7:w2642, 9:w2641, 11:w2643) -> (15:w2640:errorcluster)  [unwired: 1 in, 3 out]
                        n1646 = local write "data file error"(w2640) -> ()
                      }
                    }
                  }
                  frame #7 {
                    # "LAB04-2"
                    n1647 = case shown="True" w2684 {
                      frame False {
                      }
                      frame True {
                        n1648 = local read "LAB04-2 (DISP)"() -> (w2726:T4)
                        n1649 = local read "LAB04-2 (SIG)"() -> (w2727:T2)
                        n1650 = local read "LAB04-2 (TDMS)"() -> (w2728:refnum<k34>)
                        n1651 = Build Array("TEMP Neut") -> (w2692:string[])
                        n1652 = Build Array("CYCLE") -> (w2687:string[])
                        n1653 = Build Array("TEMP Live") -> (w2697:string[])
                        n1654 = Build Array("PF") -> (w2702:string[])
                        n1655 = Build Array("AMPS") -> (w2723:string[])
                        n1656 = Build Array("VOLTS") -> (w2714:string[])
                        n1657 = Unbundle(w2727) -> ("AMPS"=w2722:dbl, "VOLTS"=w2711:dbl, "PF"=w2710:dbl, "Tmp Live"=w2709:dbl, "Tmp Neut"=w2712:dbl)
                        n1658 = Unbundle(w2726) -> ("CYCLE"=w2707:dbl)  [unwired: 2 out]
                        n1659 = Build Array(w2711) -> (w2708:dbl[])
                        n1660 = Build Array(w2710) -> (w2701:dbl[])
                        n1661 = Build Array(w2709) -> (w2696:dbl[])
                        n1662 = Build Array(w2712) -> (w2691:dbl[])
                        n1663 = Build Array(w2722) -> (w2721:dbl[])
                        n1664 = Build Array(w2707) -> (w2686:dbl[])
                        n1665 = TDMS Write(0:w2728, 5:"LAB04-2 TEST VALUES", 7:w2723, 9:w2721) -> (4:w2716:refnum<k34>, 6:w2715:string, 15:w2703:errorcluster)  [unwired: 2 in, 1 out]
                        n1666 = TDMS Write(0:w2716, 5:w2715, 7:w2714, 9:w2708, 11:w2703) -> (4:w2706:refnum<k34>, 6:w2705:string, 15:w2704:errorcluster)  [unwired: 1 in, 1 out]
                        n1667 = TDMS Write(0:w2706, 5:w2705, 7:w2702, 9:w2701, 11:w2704) -> (4:w2700:refnum<k34>, 6:w2699:string, 15:w2698:errorcluster)  [unwired: 1 in, 1 out]
                        n1668 = TDMS Write(0:w2700, 5:w2699, 7:w2697, 9:w2696, 11:w2698) -> (4:w2695:refnum<k34>, 6:w2694:string, 15:w2693:errorcluster)  [unwired: 1 in, 1 out]
                        n1669 = TDMS Write(0:w2695, 5:w2694, 7:w2692, 9:w2691, 11:w2693) -> (4:w2690:refnum<k34>, 6:w2689:string, 15:w2688:errorcluster)  [unwired: 1 in, 1 out]
                        n1670 = TDMS Write(0:w2690, 5:w2689, 7:w2687, 9:w2686, 11:w2688) -> (15:w2685:errorcluster)  [unwired: 1 in, 3 out]
                        n1671 = local write "data file error"(w2685) -> ()
                      }
                    }
                  }
                  frame #8 {
                    # "LAB05-1"
                    n1672 = case shown="True" w2729 {
                      frame False {
                      }
                      frame True {
                        n1673 = local read "LAB05-1 (DISP)"() -> (w2771:T4)
                        n1674 = local read "LAB05-1 (SIG)"() -> (w2772:T2)
                        n1675 = local read "LAB05-1 (TDMS)"() -> (w2773:refnum<k34>)
                        n1676 = Build Array("TEMP Neut") -> (w2737:string[])
                        n1677 = Build Array("CYCLE") -> (w2732:string[])
                        n1678 = Build Array("TEMP Live") -> (w2742:string[])
                        n1679 = Build Array("PF") -> (w2747:string[])
                        n1680 = Build Array("AMPS") -> (w2768:string[])
                        n1681 = Build Array("VOLTS") -> (w2759:string[])
                        n1682 = Unbundle(w2772) -> ("AMPS"=w2767:dbl, "VOLTS"=w2756:dbl, "PF"=w2755:dbl, "Tmp Live"=w2754:dbl, "Tmp Neut"=w2757:dbl)
                        n1683 = Unbundle(w2771) -> ("CYCLE"=w2752:dbl)  [unwired: 2 out]
                        n1684 = Build Array(w2756) -> (w2753:dbl[])
                        n1685 = Build Array(w2755) -> (w2746:dbl[])
                        n1686 = Build Array(w2754) -> (w2741:dbl[])
                        n1687 = Build Array(w2757) -> (w2736:dbl[])
                        n1688 = Build Array(w2767) -> (w2766:dbl[])
                        n1689 = Build Array(w2752) -> (w2731:dbl[])
                        n1690 = TDMS Write(0:w2773, 5:"LAB05-1 TEST VALUES", 7:w2768, 9:w2766) -> (4:w2761:refnum<k34>, 6:w2760:string, 15:w2748:errorcluster)  [unwired: 2 in, 1 out]
                        n1691 = TDMS Write(0:w2761, 5:w2760, 7:w2759, 9:w2753, 11:w2748) -> (4:w2751:refnum<k34>, 6:w2750:string, 15:w2749:errorcluster)  [unwired: 1 in, 1 out]
                        n1692 = TDMS Write(0:w2751, 5:w2750, 7:w2747, 9:w2746, 11:w2749) -> (4:w2745:refnum<k34>, 6:w2744:string, 15:w2743:errorcluster)  [unwired: 1 in, 1 out]
                        n1693 = TDMS Write(0:w2745, 5:w2744, 7:w2742, 9:w2741, 11:w2743) -> (4:w2740:refnum<k34>, 6:w2739:string, 15:w2738:errorcluster)  [unwired: 1 in, 1 out]
                        n1694 = TDMS Write(0:w2740, 5:w2739, 7:w2737, 9:w2736, 11:w2738) -> (4:w2735:refnum<k34>, 6:w2734:string, 15:w2733:errorcluster)  [unwired: 1 in, 1 out]
                        n1695 = TDMS Write(0:w2735, 5:w2734, 7:w2732, 9:w2731, 11:w2733) -> (15:w2730:errorcluster)  [unwired: 1 in, 3 out]
                        n1696 = local write "data file error"(w2730) -> ()
                      }
                    }
                  }
                  frame #9 {
                    # "LAB05-2"
                    n1697 = case shown="True" w2774 {
                      frame False {
                      }
                      frame True {
                        n1698 = local read "LAB05-2 (DISP)"() -> (w2816:T4)
                        n1699 = local read "LAB05-2 (SIG)"() -> (w2817:T2)
                        n1700 = local read "LAB05-2 (TDMS)"() -> (w2818:refnum<k34>)
                        n1701 = Build Array("TEMP Neut") -> (w2782:string[])
                        n1702 = Build Array("CYCLE") -> (w2777:string[])
                        n1703 = Build Array("TEMP Live") -> (w2787:string[])
                        n1704 = Build Array("PF") -> (w2792:string[])
                        n1705 = Build Array("AMPS") -> (w2813:string[])
                        n1706 = Build Array("VOLTS") -> (w2804:string[])
                        n1707 = Unbundle(w2817) -> ("AMPS"=w2812:dbl, "VOLTS"=w2801:dbl, "PF"=w2800:dbl, "Tmp Live"=w2799:dbl, "Tmp Neut"=w2802:dbl)
                        n1708 = Unbundle(w2816) -> ("CYCLE"=w2797:dbl)  [unwired: 2 out]
                        n1709 = Build Array(w2801) -> (w2798:dbl[])
                        n1710 = Build Array(w2800) -> (w2791:dbl[])
                        n1711 = Build Array(w2799) -> (w2786:dbl[])
                        n1712 = Build Array(w2802) -> (w2781:dbl[])
                        n1713 = Build Array(w2812) -> (w2811:dbl[])
                        n1714 = Build Array(w2797) -> (w2776:dbl[])
                        n1715 = TDMS Write(0:w2818, 5:"LAB05-2 TEST VALUES", 7:w2813, 9:w2811) -> (4:w2806:refnum<k34>, 6:w2805:string, 15:w2793:errorcluster)  [unwired: 2 in, 1 out]
                        n1716 = TDMS Write(0:w2806, 5:w2805, 7:w2804, 9:w2798, 11:w2793) -> (4:w2796:refnum<k34>, 6:w2795:string, 15:w2794:errorcluster)  [unwired: 1 in, 1 out]
                        n1717 = TDMS Write(0:w2796, 5:w2795, 7:w2792, 9:w2791, 11:w2794) -> (4:w2790:refnum<k34>, 6:w2789:string, 15:w2788:errorcluster)  [unwired: 1 in, 1 out]
                        n1718 = TDMS Write(0:w2790, 5:w2789, 7:w2787, 9:w2786, 11:w2788) -> (4:w2785:refnum<k34>, 6:w2784:string, 15:w2783:errorcluster)  [unwired: 1 in, 1 out]
                        n1719 = TDMS Write(0:w2785, 5:w2784, 7:w2782, 9:w2781, 11:w2783) -> (4:w2780:refnum<k34>, 6:w2779:string, 15:w2778:errorcluster)  [unwired: 1 in, 1 out]
                        n1720 = TDMS Write(0:w2780, 5:w2779, 7:w2777, 9:w2776, 11:w2778) -> (15:w2775:errorcluster)  [unwired: 1 in, 3 out]
                        n1721 = local write "data file error"(w2775) -> ()
                      }
                    }
                  }
                }
              }
            }
          }
          frame #13 {
            # "check for cycle test fail conditions"
            n1722 = local read "on loops"() -> (w2845:dbl)
            n1723 = local read "jig cycle"() -> (w2842:dbl)
            n1724 = local read "jig cycle"() -> (w2847:dbl)
            n1725 = Add(x=w2845, y=3.0) -> (x+y=w2843:dbl)
            n1726 = Equal?(x=w2842, y=w2843) -> (x = y?=w2838:bool)
            n1727 = Equal?(x=w2847, y=1.0) -> (x = y?=w2840:bool)
            n1728 = stacked-sequence {
              tunnel: w2841 -> [w2849 _ _ _ _ _ _ _ _ _]
              tunnel: w2840 -> [w2853 w2906 w2957 w3008 w3059 w3110 w3161 w3212 w3263 w3314]
              tunnel: w2839 -> [w2859 _ _ _ _ _ _ _ _ _]
              tunnel: w2838 -> [w2852 w2905 w2956 w3007 w3058 w3109 w3160 w3211 w3262 w3313]
              tunnel: w2837 -> [_ w2902 _ _ _ _ _ _ _ _]
              tunnel: w2836 -> [_ w2901 _ _ _ _ _ _ _ _]
              tunnel: w2835 -> [_ _ w2953 _ _ _ _ _ _ _]
              tunnel: w2834 -> [_ _ w2952 _ _ _ _ _ _ _]
              tunnel: w2833 -> [_ _ _ w3004 _ _ _ _ _ _]
              tunnel: w2832 -> [_ _ _ w3003 _ _ _ _ _ _]
              tunnel: w2831 -> [_ _ _ _ w3055 _ _ _ _ _]
              tunnel: w2830 -> [_ _ _ _ w3054 _ _ _ _ _]
              tunnel: w2829 -> [_ _ _ _ _ w3106 _ _ _ _]
              tunnel: w2828 -> [_ _ _ _ _ w3105 _ _ _ _]
              tunnel: w2827 -> [_ _ _ _ _ _ w3157 _ _ _]
              tunnel: w2826 -> [_ _ _ _ _ _ w3156 _ _ _]
              tunnel: w2825 -> [_ _ _ _ _ _ _ w3208 _ _]
              tunnel: w2824 -> [_ _ _ _ _ _ _ w3207 _ _]
              tunnel: w2823 -> [_ _ _ _ _ _ _ _ w3259 _]
              tunnel: w2822 -> [_ _ _ _ _ _ _ _ w3258 _]
              tunnel: w2821 -> [_ _ _ _ _ _ _ _ _ w3310]
              tunnel: w2820 -> [_ _ _ _ _ _ _ _ _ w3309]
              tunnel: 2.0 -> [w2848 w2900 w2951 w3002 w3053 w3104 w3155 w3206 w3257 w3308]
              frame #0 {
                # "LAB01-1"
                n1729 = local read "LAB01-1 (SIG)"() -> (w2855:T2)
                n1730 = Or(x=w2853, y=w2852) -> (x .or. y?=w2857:bool)
                n1731 = case shown="\"CYCLE TEST\"" w2849 {
                  tunnel: [FALSE TRUE FALSE] -> w2850
                  frame "TEST SET UP", Default {
                  }
                  frame "CYCLE TEST" {
                  }
                  frame "T-RISE TEST" {
                  }
                }
                n1732 = And(x=w2859, y=w2857) -> (x .and. y?=w2856:bool)
                n1733 = local read "LAB01-1 (TDMS)"() -> (w2851:refnum<k34>)
                n1734 = Unbundle(w2855) -> ("AMPS"=w2854:dbl)  [unwired: 4 out]
                n1735 = And(x=w2850, y=w2856) -> (x .and. y?=w2858:bool)
                n1736 = case shown="True" w2858 {
                  tunnel: w2854 -> [_ w2868]
                  tunnel: w2853 -> [_ w2870]
                  tunnel: w2852 -> [_ w2869]
                  tunnel: w2851 -> [_ w2862]
                  tunnel: w2848 -> [_ w2861]
                  tunnel: w2848 -> [_ w2860]
                  frame False {
                  }
                  frame True {
                    # "check for amps fail"
                    n1737 = case shown="True" w2869 {
                      tunnel: w2868 -> [_ w2876]
                      tunnel: [FALSE w2875] -> w2866
                      tunnel: ["" "AMPS HI"] -> w2864
                      tunnel: w2861 -> [_ w2873]
                      frame False {
                      }
                      frame True {
                        n1738 = Greater?(x=w2876, y=w2873) -> (0:w2875:bool)
                      }
                    }
                    n1739 = case shown="True" w2870 {
                      tunnel: w2868 -> [_ w2882]
                      tunnel: [FALSE w2881] -> w2867
                      tunnel: ["" "AMPS LO"] -> w2863
                      tunnel: w2860 -> [_ w2879]
                      frame False {
                      }
                      frame True {
                        n1740 = Less?(x=w2882, y=w2879) -> (x < y?=w2881:bool)
                      }
                    }
                    n1741 = Or(x=w2867, y=w2866) -> (x .or. y?=w2865:bool)
                    n1742 = case shown="True" w2865 {
                      tunnel: w2864 -> [_ w2885]
                      tunnel: w2863 -> [_ w2884]
                      tunnel: w2862 -> [_ w2883]
                      frame False {
                      }
                      frame True {
                        n1743 = stacked-sequence {
                          tunnel: w2885 -> [w2890 _]
                          tunnel: w2884 -> [w2889 _]
                          tunnel: w2883 -> [w2886 _]
                          frame #0 {
                            n1744 = Build Array(w2890, w2889) -> (w2888:string[])
                            n1745 = TDMS Write(0:w2886, 5:"TEST RESULT", 7:"AMPS FAIL ", 9:w2888) -> (15:w2892:errorcluster)  [unwired: 2 in, 3 out]
                            n1746 = local write "data file error"(w2892) -> ()
                          }
                          frame #1 {
                            n1747 = local read "LAB01-1 (DISP)"() -> (w2896:T4)
                            n1748 = Bundle(cluster=w2896, "STATUS"="STOP") -> (w2895:T4)  [unwired: 2 in]
                            n1749 = local write "LAB01-1 (RESULT)"(FALSE) -> ()
                            n1750 = local write "LAB01-1 (DISP)"(w2895) -> ()
                          }
                        }
                      }
                    }
                  }
                }
              }
              frame #1 {
                # "LAB01-2"
                n1751 = local read "LAB01-2 (SIG)"() -> (w2908:T2)
                n1752 = Or(x=w2906, y=w2905) -> (x .or. y?=w2910:bool)
                n1753 = case shown="\"CYCLE TEST\"" w2901 {
                  tunnel: [FALSE TRUE FALSE] -> w2903
                  frame "TEST SET UP", Default {
                  }
                  frame "CYCLE TEST" {
                  }
                  frame "T-RISE TEST" {
                  }
                }
                n1754 = And(x=w2902, y=w2910) -> (x .and. y?=w2909:bool)
                n1755 = local read "LAB01-2 (TDMS)"() -> (w2904:refnum<k34>)
                n1756 = Unbundle(w2908) -> ("AMPS"=w2907:dbl)  [unwired: 4 out]
                n1757 = And(x=w2903, y=w2909) -> (x .and. y?=w2911:bool)
                n1758 = case shown="True" w2911 {
                  tunnel: w2907 -> [_ w2919]
                  tunnel: w2906 -> [_ w2921]
                  tunnel: w2905 -> [_ w2920]
                  tunnel: w2904 -> [_ w2913]
                  tunnel: w2900 -> [_ w2912]
                  frame False {
                  }
                  frame True {
                    # "check for amps fail"
                    n1759 = case shown="True" w2920 {
                      tunnel: w2919 -> [_ w2927]
                      tunnel: [FALSE w2926] -> w2917
                      tunnel: ["" "AMPS HI"] -> w2915
                      tunnel: w2912 -> [_ w2924]
                      frame False {
                      }
                      frame True {
                        n1760 = Greater?(x=w2927, y=w2924) -> (0:w2926:bool)
                      }
                    }
                    n1761 = case shown="True" w2921 {
                      tunnel: w2919 -> [_ w2933]
                      tunnel: [FALSE w2932] -> w2918
                      tunnel: ["" "AMPS LO"] -> w2914
                      tunnel: w2912 -> [_ w2930]
                      frame False {
                      }
                      frame True {
                        n1762 = Less?(x=w2933, y=w2930) -> (x < y?=w2932:bool)
                      }
                    }
                    n1763 = Or(x=w2918, y=w2917) -> (x .or. y?=w2916:bool)
                    n1764 = case shown="True" w2916 {
                      tunnel: w2915 -> [_ w2936]
                      tunnel: w2914 -> [_ w2935]
                      tunnel: w2913 -> [_ w2934]
                      frame False {
                      }
                      frame True {
                        n1765 = stacked-sequence {
                          tunnel: w2936 -> [w2941 _]
                          tunnel: w2935 -> [w2940 _]
                          tunnel: w2934 -> [w2937 _]
                          frame #0 {
                            n1766 = Build Array(w2941, w2940) -> (w2939:string[])
                            n1767 = TDMS Write(0:w2937, 5:"TEST RESULT", 7:"AMPS FAIL ", 9:w2939) -> (15:w2943:errorcluster)  [unwired: 2 in, 3 out]
                            n1768 = local write "data file error"(w2943) -> ()
                          }
                          frame #1 {
                            n1769 = local read "LAB01-2 (DISP)"() -> (w2947:T4)
                            n1770 = Bundle(cluster=w2947, "STATUS"="STOP") -> (w2946:T4)  [unwired: 2 in]
                            n1771 = local write "LAB01-2 (RESULT)"(FALSE) -> ()
                            n1772 = local write "LAB01-2 (DISP)"(w2946) -> ()
                          }
                        }
                      }
                    }
                  }
                }
              }
              frame #2 {
                # "LAB02-1"
                n1773 = local read "LAB02-1 (SIG)"() -> (w2959:T2)
                n1774 = Or(x=w2957, y=w2956) -> (x .or. y?=w2961:bool)
                n1775 = case shown="\"CYCLE TEST\"" w2952 {
                  tunnel: [FALSE TRUE FALSE] -> w2954
                  frame "TEST SET UP", Default {
                  }
                  frame "CYCLE TEST" {
                  }
                  frame "T-RISE TEST" {
                  }
                }
                n1776 = And(x=w2953, y=w2961) -> (x .and. y?=w2960:bool)
                n1777 = local read "LAB02-1 (TDMS)"() -> (w2955:refnum<k34>)
                n1778 = Unbundle(w2959) -> ("AMPS"=w2958:dbl)  [unwired: 4 out]
                n1779 = And(x=w2954, y=w2960) -> (x .and. y?=w2962:bool)
                n1780 = case shown="True" w2962 {
                  tunnel: w2958 -> [_ w2970]
                  tunnel: w2957 -> [_ w2972]
                  tunnel: w2956 -> [_ w2971]
                  tunnel: w2955 -> [_ w2964]
                  tunnel: w2951 -> [_ w2963]
                  frame False {
                  }
                  frame True {
                    # "check for amps fail"
                    n1781 = case shown="True" w2971 {
                      tunnel: w2970 -> [_ w2978]
                      tunnel: [FALSE w2977] -> w2968
                      tunnel: ["" "AMPS HI"] -> w2966
                      tunnel: w2963 -> [_ w2975]
                      frame False {
                      }
                      frame True {
                        n1782 = Greater?(x=w2978, y=w2975) -> (0:w2977:bool)
                      }
                    }
                    n1783 = case shown="True" w2972 {
                      tunnel: w2970 -> [_ w2984]
                      tunnel: [FALSE w2983] -> w2969
                      tunnel: ["" "AMPS LO"] -> w2965
                      tunnel: w2963 -> [_ w2981]
                      frame False {
                      }
                      frame True {
                        n1784 = Less?(x=w2984, y=w2981) -> (x < y?=w2983:bool)
                      }
                    }
                    n1785 = Or(x=w2969, y=w2968) -> (x .or. y?=w2967:bool)
                    n1786 = case shown="True" w2967 {
                      tunnel: w2966 -> [_ w2987]
                      tunnel: w2965 -> [_ w2986]
                      tunnel: w2964 -> [_ w2985]
                      frame False {
                      }
                      frame True {
                        n1787 = stacked-sequence {
                          tunnel: w2987 -> [w2992 _]
                          tunnel: w2986 -> [w2991 _]
                          tunnel: w2985 -> [w2988 _]
                          frame #0 {
                            n1788 = Build Array(w2992, w2991) -> (w2990:string[])
                            n1789 = TDMS Write(0:w2988, 5:"TEST RESULT", 7:"AMPS FAIL ", 9:w2990) -> (15:w2994:errorcluster)  [unwired: 2 in, 3 out]
                            n1790 = local write "data file error"(w2994) -> ()
                          }
                          frame #1 {
                            n1791 = local read "LAB02-1 (DISP)"() -> (w2998:T4)
                            n1792 = Bundle(cluster=w2998, "STATUS"="STOP") -> (w2997:T4)  [unwired: 2 in]
                            n1793 = local write "LAB02-1 (RESULT)"(FALSE) -> ()
                            n1794 = local write "LAB02-1 (DISP)"(w2997) -> ()
                          }
                        }
                      }
                    }
                  }
                }
              }
              frame #3 {
                # "LAB02-2"
                n1795 = local read "LAB02-2 (SIG)"() -> (w3010:T2)
                n1796 = Or(x=w3008, y=w3007) -> (x .or. y?=w3012:bool)
                n1797 = case shown="\"CYCLE TEST\"" w3003 {
                  tunnel: [FALSE TRUE FALSE] -> w3005
                  frame "TEST SET UP", Default {
                  }
                  frame "CYCLE TEST" {
                  }
                  frame "T-RISE TEST" {
                  }
                }
                n1798 = And(x=w3004, y=w3012) -> (x .and. y?=w3011:bool)
                n1799 = local read "LAB02-2 (TDMS)"() -> (w3006:refnum<k34>)
                n1800 = Unbundle(w3010) -> ("AMPS"=w3009:dbl)  [unwired: 4 out]
                n1801 = And(x=w3005, y=w3011) -> (x .and. y?=w3013:bool)
                n1802 = case shown="True" w3013 {
                  tunnel: w3009 -> [_ w3021]
                  tunnel: w3008 -> [_ w3023]
                  tunnel: w3007 -> [_ w3022]
                  tunnel: w3006 -> [_ w3015]
                  tunnel: w3002 -> [_ w3014]
                  frame False {
                  }
                  frame True {
                    # "check for amps fail"
                    n1803 = case shown="True" w3022 {
                      tunnel: w3021 -> [_ w3029]
                      tunnel: [FALSE w3028] -> w3019
                      tunnel: ["" "AMPS HI"] -> w3017
                      tunnel: w3014 -> [_ w3026]
                      frame False {
                      }
                      frame True {
                        n1804 = Greater?(x=w3029, y=w3026) -> (0:w3028:bool)
                      }
                    }
                    n1805 = case shown="True" w3023 {
                      tunnel: w3021 -> [_ w3035]
                      tunnel: [FALSE w3034] -> w3020
                      tunnel: ["" "AMPS LO"] -> w3016
                      tunnel: w3014 -> [_ w3032]
                      frame False {
                      }
                      frame True {
                        n1806 = Less?(x=w3035, y=w3032) -> (x < y?=w3034:bool)
                      }
                    }
                    n1807 = Or(x=w3020, y=w3019) -> (x .or. y?=w3018:bool)
                    n1808 = case shown="True" w3018 {
                      tunnel: w3017 -> [_ w3038]
                      tunnel: w3016 -> [_ w3037]
                      tunnel: w3015 -> [_ w3036]
                      frame False {
                      }
                      frame True {
                        n1809 = stacked-sequence {
                          tunnel: w3038 -> [w3043 _]
                          tunnel: w3037 -> [w3042 _]
                          tunnel: w3036 -> [w3039 _]
                          frame #0 {
                            n1810 = Build Array(w3043, w3042) -> (w3041:string[])
                            n1811 = TDMS Write(0:w3039, 5:"TEST RESULT", 7:"AMPS FAIL ", 9:w3041) -> (15:w3045:errorcluster)  [unwired: 2 in, 3 out]
                            n1812 = local write "data file error"(w3045) -> ()
                          }
                          frame #1 {
                            n1813 = local read "LAB02-2 (DISP)"() -> (w3049:T4)
                            n1814 = Bundle(cluster=w3049, "STATUS"="STOP") -> (w3048:T4)  [unwired: 2 in]
                            n1815 = local write "LAB02-2 (RESULT)"(FALSE) -> ()
                            n1816 = local write "LAB02-2 (DISP)"(w3048) -> ()
                          }
                        }
                      }
                    }
                  }
                }
              }
              frame #4 {
                # "LAB03-1"
                n1817 = local read "LAB03-1 (SIG)"() -> (w3061:T2)
                n1818 = Or(x=w3059, y=w3058) -> (x .or. y?=w3063:bool)
                n1819 = case shown="\"CYCLE TEST\"" w3054 {
                  tunnel: [FALSE TRUE FALSE] -> w3056
                  frame "TEST SET UP", Default {
                  }
                  frame "CYCLE TEST" {
                  }
                  frame "T-RISE TEST" {
                  }
                }
                n1820 = And(x=w3055, y=w3063) -> (x .and. y?=w3062:bool)
                n1821 = local read "LAB03-1 (TDMS)"() -> (w3057:refnum<k34>)
                n1822 = Unbundle(w3061) -> ("AMPS"=w3060:dbl)  [unwired: 4 out]
                n1823 = And(x=w3056, y=w3062) -> (x .and. y?=w3064:bool)
                n1824 = case shown="True" w3064 {
                  tunnel: w3060 -> [_ w3072]
                  tunnel: w3059 -> [_ w3074]
                  tunnel: w3058 -> [_ w3073]
                  tunnel: w3057 -> [_ w3066]
                  tunnel: w3053 -> [_ w3065]
                  frame False {
                  }
                  frame True {
                    # "check for amps fail"
                    n1825 = case shown="True" w3073 {
                      tunnel: w3072 -> [_ w3080]
                      tunnel: [FALSE w3079] -> w3070
                      tunnel: ["" "AMPS HI"] -> w3068
                      tunnel: w3065 -> [_ w3077]
                      frame False {
                      }
                      frame True {
                        n1826 = Greater?(x=w3080, y=w3077) -> (0:w3079:bool)
                      }
                    }
                    n1827 = case shown="True" w3074 {
                      tunnel: w3072 -> [_ w3086]
                      tunnel: [FALSE w3085] -> w3071
                      tunnel: ["" "AMPS LO"] -> w3067
                      tunnel: w3065 -> [_ w3083]
                      frame False {
                      }
                      frame True {
                        n1828 = Less?(x=w3086, y=w3083) -> (x < y?=w3085:bool)
                      }
                    }
                    n1829 = Or(x=w3071, y=w3070) -> (x .or. y?=w3069:bool)
                    n1830 = case shown="True" w3069 {
                      tunnel: w3068 -> [_ w3089]
                      tunnel: w3067 -> [_ w3088]
                      tunnel: w3066 -> [_ w3087]
                      frame False {
                      }
                      frame True {
                        n1831 = stacked-sequence {
                          tunnel: w3089 -> [w3094 _]
                          tunnel: w3088 -> [w3093 _]
                          tunnel: w3087 -> [w3090 _]
                          frame #0 {
                            n1832 = Build Array(w3094, w3093) -> (w3092:string[])
                            n1833 = TDMS Write(0:w3090, 5:"TEST RESULT", 7:"AMPS FAIL ", 9:w3092) -> (15:w3096:errorcluster)  [unwired: 2 in, 3 out]
                            n1834 = local write "data file error"(w3096) -> ()
                          }
                          frame #1 {
                            n1835 = local read "LAB03-1 (DISP)"() -> (w3100:T4)
                            n1836 = Bundle(cluster=w3100, "STATUS"="STOP") -> (w3099:T4)  [unwired: 2 in]
                            n1837 = local write "LAB03-1 (RESULT)"(FALSE) -> ()
                            n1838 = local write "LAB03-1 (DISP)"(w3099) -> ()
                          }
                        }
                      }
                    }
                  }
                }
              }
              frame #5 {
                # "LAB03-2"
                n1839 = local read "LAB03-2 (SIG)"() -> (w3112:T2)
                n1840 = Or(x=w3110, y=w3109) -> (x .or. y?=w3114:bool)
                n1841 = case shown="\"CYCLE TEST\"" w3105 {
                  tunnel: [FALSE TRUE FALSE] -> w3107
                  frame "TEST SET UP", Default {
                  }
                  frame "CYCLE TEST" {
                  }
                  frame "T-RISE TEST" {
                  }
                }
                n1842 = And(x=w3106, y=w3114) -> (x .and. y?=w3113:bool)
                n1843 = local read "LAB03-2 (TDMS)"() -> (w3108:refnum<k34>)
                n1844 = Unbundle(w3112) -> ("AMPS"=w3111:dbl)  [unwired: 4 out]
                n1845 = And(x=w3107, y=w3113) -> (x .and. y?=w3115:bool)
                n1846 = case shown="True" w3115 {
                  tunnel: w3111 -> [_ w3123]
                  tunnel: w3110 -> [_ w3125]
                  tunnel: w3109 -> [_ w3124]
                  tunnel: w3108 -> [_ w3117]
                  tunnel: w3104 -> [_ w3116]
                  frame False {
                  }
                  frame True {
                    # "check for amps fail"
                    n1847 = case shown="True" w3124 {
                      tunnel: w3123 -> [_ w3131]
                      tunnel: [FALSE w3130] -> w3121
                      tunnel: ["" "AMPS HI"] -> w3119
                      tunnel: w3116 -> [_ w3128]
                      frame False {
                      }
                      frame True {
                        n1848 = Greater?(x=w3131, y=w3128) -> (0:w3130:bool)
                      }
                    }
                    n1849 = case shown="True" w3125 {
                      tunnel: w3123 -> [_ w3137]
                      tunnel: [FALSE w3136] -> w3122
                      tunnel: ["" "AMPS LO"] -> w3118
                      tunnel: w3116 -> [_ w3134]
                      frame False {
                      }
                      frame True {
                        n1850 = Less?(x=w3137, y=w3134) -> (x < y?=w3136:bool)
                      }
                    }
                    n1851 = Or(x=w3122, y=w3121) -> (x .or. y?=w3120:bool)
                    n1852 = case shown="True" w3120 {
                      tunnel: w3119 -> [_ w3140]
                      tunnel: w3118 -> [_ w3139]
                      tunnel: w3117 -> [_ w3138]
                      frame False {
                      }
                      frame True {
                        n1853 = stacked-sequence {
                          tunnel: w3140 -> [w3145 _]
                          tunnel: w3139 -> [w3144 _]
                          tunnel: w3138 -> [w3141 _]
                          frame #0 {
                            n1854 = Build Array(w3145, w3144) -> (w3143:string[])
                            n1855 = TDMS Write(0:w3141, 5:"TEST RESULT", 7:"AMPS FAIL ", 9:w3143) -> (15:w3147:errorcluster)  [unwired: 2 in, 3 out]
                            n1856 = local write "data file error"(w3147) -> ()
                          }
                          frame #1 {
                            n1857 = local read "LAB03-2 (DISP)"() -> (w3151:T4)
                            n1858 = Bundle(cluster=w3151, "STATUS"="STOP") -> (w3150:T4)  [unwired: 2 in]
                            n1859 = local write "LAB03-2 (RESULT)"(FALSE) -> ()
                            n1860 = local write "LAB03-2 (DISP)"(w3150) -> ()
                          }
                        }
                      }
                    }
                  }
                }
              }
              frame #6 {
                # "LAB04-1"
                n1861 = local read "LAB04-1 (SIG)"() -> (w3163:T2)
                n1862 = Or(x=w3161, y=w3160) -> (x .or. y?=w3165:bool)
                n1863 = case shown="\"CYCLE TEST\"" w3156 {
                  tunnel: [FALSE TRUE FALSE] -> w3158
                  frame "TEST SET UP", Default {
                  }
                  frame "CYCLE TEST" {
                  }
                  frame "T-RISE TEST" {
                  }
                }
                n1864 = And(x=w3157, y=w3165) -> (x .and. y?=w3164:bool)
                n1865 = local read "LAB04-1 (TDMS)"() -> (w3159:refnum<k34>)
                n1866 = Unbundle(w3163) -> ("AMPS"=w3162:dbl)  [unwired: 4 out]
                n1867 = And(x=w3158, y=w3164) -> (x .and. y?=w3166:bool)
                n1868 = case shown="True" w3166 {
                  tunnel: w3162 -> [_ w3174]
                  tunnel: w3161 -> [_ w3176]
                  tunnel: w3160 -> [_ w3175]
                  tunnel: w3159 -> [_ w3168]
                  tunnel: w3155 -> [_ w3167]
                  frame False {
                  }
                  frame True {
                    # "check for amps fail"
                    n1869 = case shown="True" w3175 {
                      tunnel: w3174 -> [_ w3182]
                      tunnel: [FALSE w3181] -> w3172
                      tunnel: ["" "AMPS HI"] -> w3170
                      tunnel: w3167 -> [_ w3179]
                      frame False {
                      }
                      frame True {
                        n1870 = Greater?(x=w3182, y=w3179) -> (0:w3181:bool)
                      }
                    }
                    n1871 = case shown="True" w3176 {
                      tunnel: w3174 -> [_ w3188]
                      tunnel: [FALSE w3187] -> w3173
                      tunnel: ["" "AMPS LO"] -> w3169
                      tunnel: w3167 -> [_ w3185]
                      frame False {
                      }
                      frame True {
                        n1872 = Less?(x=w3188, y=w3185) -> (x < y?=w3187:bool)
                      }
                    }
                    n1873 = Or(x=w3173, y=w3172) -> (x .or. y?=w3171:bool)
                    n1874 = case shown="True" w3171 {
                      tunnel: w3170 -> [_ w3191]
                      tunnel: w3169 -> [_ w3190]
                      tunnel: w3168 -> [_ w3189]
                      frame False {
                      }
                      frame True {
                        n1875 = stacked-sequence {
                          tunnel: w3191 -> [w3196 _]
                          tunnel: w3190 -> [w3195 _]
                          tunnel: w3189 -> [w3192 _]
                          frame #0 {
                            n1876 = Build Array(w3196, w3195) -> (w3194:string[])
                            n1877 = TDMS Write(0:w3192, 5:"TEST RESULT", 7:"AMPS FAIL ", 9:w3194) -> (15:w3198:errorcluster)  [unwired: 2 in, 3 out]
                            n1878 = local write "data file error"(w3198) -> ()
                          }
                          frame #1 {
                            n1879 = local read "LAB04-1 (DISP)"() -> (w3202:T4)
                            n1880 = Bundle(cluster=w3202, "STATUS"="STOP") -> (w3201:T4)  [unwired: 2 in]
                            n1881 = local write "LAB04-1 (RESULT)"(FALSE) -> ()
                            n1882 = local write "LAB04-1 (DISP)"(w3201) -> ()
                          }
                        }
                      }
                    }
                  }
                }
              }
              frame #7 {
                # "LAB04-2"
                n1883 = local read "LAB04-2 (SIG)"() -> (w3214:T2)
                n1884 = Or(x=w3212, y=w3211) -> (x .or. y?=w3216:bool)
                n1885 = case shown="\"CYCLE TEST\"" w3207 {
                  tunnel: [FALSE TRUE FALSE] -> w3209
                  frame "TEST SET UP", Default {
                  }
                  frame "CYCLE TEST" {
                  }
                  frame "T-RISE TEST" {
                  }
                }
                n1886 = And(x=w3208, y=w3216) -> (x .and. y?=w3215:bool)
                n1887 = local read "LAB04-2 (TDMS)"() -> (w3210:refnum<k34>)
                n1888 = Unbundle(w3214) -> ("AMPS"=w3213:dbl)  [unwired: 4 out]
                n1889 = And(x=w3209, y=w3215) -> (x .and. y?=w3217:bool)
                n1890 = case shown="True" w3217 {
                  tunnel: w3213 -> [_ w3225]
                  tunnel: w3212 -> [_ w3227]
                  tunnel: w3211 -> [_ w3226]
                  tunnel: w3210 -> [_ w3219]
                  tunnel: w3206 -> [_ w3218]
                  frame False {
                  }
                  frame True {
                    # "check for amps fail"
                    n1891 = case shown="True" w3226 {
                      tunnel: w3225 -> [_ w3233]
                      tunnel: [FALSE w3232] -> w3223
                      tunnel: ["" "AMPS HI"] -> w3221
                      tunnel: w3218 -> [_ w3230]
                      frame False {
                      }
                      frame True {
                        n1892 = Greater?(x=w3233, y=w3230) -> (0:w3232:bool)
                      }
                    }
                    n1893 = case shown="True" w3227 {
                      tunnel: w3225 -> [_ w3239]
                      tunnel: [FALSE w3238] -> w3224
                      tunnel: ["" "AMPS LO"] -> w3220
                      tunnel: w3218 -> [_ w3236]
                      frame False {
                      }
                      frame True {
                        n1894 = Less?(x=w3239, y=w3236) -> (x < y?=w3238:bool)
                      }
                    }
                    n1895 = Or(x=w3224, y=w3223) -> (x .or. y?=w3222:bool)
                    n1896 = case shown="True" w3222 {
                      tunnel: w3221 -> [_ w3242]
                      tunnel: w3220 -> [_ w3241]
                      tunnel: w3219 -> [_ w3240]
                      frame False {
                      }
                      frame True {
                        n1897 = stacked-sequence {
                          tunnel: w3242 -> [w3247 _]
                          tunnel: w3241 -> [w3246 _]
                          tunnel: w3240 -> [w3243 _]
                          frame #0 {
                            n1898 = Build Array(w3247, w3246) -> (w3245:string[])
                            n1899 = TDMS Write(0:w3243, 5:"TEST RESULT", 7:"AMPS FAIL ", 9:w3245) -> (15:w3249:errorcluster)  [unwired: 2 in, 3 out]
                            n1900 = local write "data file error"(w3249) -> ()
                          }
                          frame #1 {
                            n1901 = local read "LAB04-2 (DISP)"() -> (w3253:T4)
                            n1902 = Bundle(cluster=w3253, "STATUS"="STOP") -> (w3252:T4)  [unwired: 2 in]
                            n1903 = local write "LAB04-2 (RESULT)"(FALSE) -> ()
                            n1904 = local write "LAB04-2 (DISP)"(w3252) -> ()
                          }
                        }
                      }
                    }
                  }
                }
              }
              frame #8 {
                # "LAB05-1"
                n1905 = local read "LAB05-1 (SIG)"() -> (w3265:T2)
                n1906 = Or(x=w3263, y=w3262) -> (x .or. y?=w3267:bool)
                n1907 = case shown="\"CYCLE TEST\"" w3258 {
                  tunnel: [FALSE TRUE FALSE] -> w3260
                  frame "TEST SET UP", Default {
                  }
                  frame "CYCLE TEST" {
                  }
                  frame "T-RISE TEST" {
                  }
                }
                n1908 = And(x=w3259, y=w3267) -> (x .and. y?=w3266:bool)
                n1909 = local read "LAB05-1 (TDMS)"() -> (w3261:refnum<k34>)
                n1910 = Unbundle(w3265) -> ("AMPS"=w3264:dbl)  [unwired: 4 out]
                n1911 = And(x=w3260, y=w3266) -> (x .and. y?=w3268:bool)
                n1912 = case shown="True" w3268 {
                  tunnel: w3264 -> [_ w3276]
                  tunnel: w3263 -> [_ w3278]
                  tunnel: w3262 -> [_ w3277]
                  tunnel: w3261 -> [_ w3270]
                  tunnel: w3257 -> [_ w3269]
                  frame False {
                  }
                  frame True {
                    # "check for amps fail"
                    n1913 = case shown="True" w3277 {
                      tunnel: w3276 -> [_ w3284]
                      tunnel: [FALSE w3283] -> w3274
                      tunnel: ["" "AMPS HI"] -> w3272
                      tunnel: w3269 -> [_ w3281]
                      frame False {
                      }
                      frame True {
                        n1914 = Greater?(x=w3284, y=w3281) -> (0:w3283:bool)
                      }
                    }
                    n1915 = case shown="True" w3278 {
                      tunnel: w3276 -> [_ w3290]
                      tunnel: [FALSE w3289] -> w3275
                      tunnel: ["" "AMPS LO"] -> w3271
                      tunnel: w3269 -> [_ w3287]
                      frame False {
                      }
                      frame True {
                        n1916 = Less?(x=w3290, y=w3287) -> (x < y?=w3289:bool)
                      }
                    }
                    n1917 = Or(x=w3275, y=w3274) -> (x .or. y?=w3273:bool)
                    n1918 = case shown="True" w3273 {
                      tunnel: w3272 -> [_ w3293]
                      tunnel: w3271 -> [_ w3292]
                      tunnel: w3270 -> [_ w3291]
                      frame False {
                      }
                      frame True {
                        n1919 = stacked-sequence {
                          tunnel: w3293 -> [w3298 _]
                          tunnel: w3292 -> [w3297 _]
                          tunnel: w3291 -> [w3294 _]
                          frame #0 {
                            n1920 = Build Array(w3298, w3297) -> (w3296:string[])
                            n1921 = TDMS Write(0:w3294, 5:"TEST RESULT", 7:"AMPS FAIL ", 9:w3296) -> (15:w3300:errorcluster)  [unwired: 2 in, 3 out]
                            n1922 = local write "data file error"(w3300) -> ()
                          }
                          frame #1 {
                            n1923 = local read "LAB05-1 (DISP)"() -> (w3304:T4)
                            n1924 = Bundle(cluster=w3304, "STATUS"="STOP") -> (w3303:T4)  [unwired: 2 in]
                            n1925 = local write "LAB05-1 (RESULT)"(FALSE) -> ()
                            n1926 = local write "LAB05-1 (DISP)"(w3303) -> ()
                          }
                        }
                      }
                    }
                  }
                }
              }
              frame #9 {
                # "LAB05-2"
                n1927 = local read "LAB05-2 (SIG)"() -> (w3316:T2)
                n1928 = Or(x=w3314, y=w3313) -> (x .or. y?=w3318:bool)
                n1929 = case shown="\"CYCLE TEST\"" w3309 {
                  tunnel: [FALSE TRUE FALSE] -> w3311
                  frame "TEST SET UP", Default {
                  }
                  frame "CYCLE TEST" {
                  }
                  frame "T-RISE TEST" {
                  }
                }
                n1930 = And(x=w3310, y=w3318) -> (x .and. y?=w3317:bool)
                n1931 = local read "LAB05-2 (TDMS)"() -> (w3312:refnum<k34>)
                n1932 = Unbundle(w3316) -> ("AMPS"=w3315:dbl)  [unwired: 4 out]
                n1933 = And(x=w3311, y=w3317) -> (x .and. y?=w3319:bool)
                n1934 = case shown="True" w3319 {
                  tunnel: w3315 -> [_ w3327]
                  tunnel: w3314 -> [_ w3329]
                  tunnel: w3313 -> [_ w3328]
                  tunnel: w3312 -> [_ w3321]
                  tunnel: w3308 -> [_ w3320]
                  frame False {
                  }
                  frame True {
                    # "check for amps fail"
                    n1935 = case shown="True" w3328 {
                      tunnel: w3327 -> [_ w3335]
                      tunnel: [FALSE w3334] -> w3325
                      tunnel: ["" "AMPS HI"] -> w3323
                      tunnel: w3320 -> [_ w3332]
                      frame False {
                      }
                      frame True {
                        n1936 = Greater?(x=w3335, y=w3332) -> (0:w3334:bool)
                      }
                    }
                    n1937 = case shown="True" w3329 {
                      tunnel: w3327 -> [_ w3341]
                      tunnel: [FALSE w3340] -> w3326
                      tunnel: ["" "AMPS LO"] -> w3322
                      tunnel: w3320 -> [_ w3338]
                      frame False {
                      }
                      frame True {
                        n1938 = Less?(x=w3341, y=w3338) -> (x < y?=w3340:bool)
                      }
                    }
                    n1939 = Or(x=w3326, y=w3325) -> (x .or. y?=w3324:bool)
                    n1940 = case shown="True" w3324 {
                      tunnel: w3323 -> [_ w3344]
                      tunnel: w3322 -> [_ w3343]
                      tunnel: w3321 -> [_ w3342]
                      frame False {
                      }
                      frame True {
                        n1941 = stacked-sequence {
                          tunnel: w3344 -> [w3349 _]
                          tunnel: w3343 -> [w3348 _]
                          tunnel: w3342 -> [w3345 _]
                          frame #0 {
                            n1942 = Build Array(w3349, w3348) -> (w3347:string[])
                            n1943 = TDMS Write(0:w3345, 5:"TEST RESULT", 7:"AMPS FAIL ", 9:w3347) -> (15:w3351:errorcluster)  [unwired: 2 in, 3 out]
                            n1944 = local write "data file error"(w3351) -> ()
                          }
                          frame #1 {
                            n1945 = local read "LAB05-2 (DISP)"() -> (w3355:T4)
                            n1946 = Bundle(cluster=w3355, "STATUS"="STOP") -> (w3354:T4)  [unwired: 2 in]
                            n1947 = local write "LAB05-2 (RESULT)"(FALSE) -> ()
                            n1948 = local write "LAB05-2 (DISP)"(w3354) -> ()
                          }
                        }
                      }
                    }
                  }
                }
              }
            }
          }
          frame #14 {
            # "check for temperature rise test fail conditions"
            n1949 = stacked-sequence {
              tunnel: w3379 -> [w3401 _ _ _ _ _ _ _ _ _]
              tunnel: w3378 -> [w3400 _ _ _ _ _ _ _ _ _]
              tunnel: w3377 -> [_ w3438 _ _ _ _ _ _ _ _]
              tunnel: w3376 -> [_ _ w3494 _ _ _ _ _ _ _]
              tunnel: w3375 -> [_ _ _ w3550 _ _ _ _ _ _]
              tunnel: w3374 -> [_ _ _ _ w3606 _ _ _ _ _]
              tunnel: w3373 -> [_ _ _ _ _ w3662 _ _ _ _]
              tunnel: w3372 -> [_ _ _ _ _ _ w3718 _ _ _]
              tunnel: w3371 -> [_ _ _ _ _ _ _ w3774 _ _]
              tunnel: w3370 -> [_ _ _ _ _ _ _ _ w3830 _]
              tunnel: w3369 -> [_ _ _ _ _ _ _ _ _ w3886]
              tunnel: w3368 -> [_ w3437 _ _ _ _ _ _ _ _]
              tunnel: w3367 -> [_ _ w3493 _ _ _ _ _ _ _]
              tunnel: w3366 -> [_ _ _ w3549 _ _ _ _ _ _]
              tunnel: w3365 -> [_ _ _ _ w3605 _ _ _ _ _]
              tunnel: w3364 -> [_ _ _ _ _ w3661 _ _ _ _]
              tunnel: w3363 -> [_ _ _ _ _ _ _ w3773 _ _]
              tunnel: w3362 -> [_ _ _ _ _ _ _ _ w3829 _]
              tunnel: w3361 -> [_ _ _ _ _ _ _ _ _ w3885]
              tunnel: w3360 -> [_ _ _ _ _ _ w3717 _ _ _]
              tunnel: 2.0 -> [w3380 w3436 w3492 w3548 w3604 w3660 w3716 w3772 w3828 w3884]
              frame #0 {
                # "LAB01-1"
                n1950 = local read "LAB01-1 (TEMP START)"() -> (w3394:cluster{"TL":dbl, "TN":dbl})
                n1951 = local read "LAB01-1 (DISP)"() -> (w3385:T4)
                n1952 = local read "LAB01-1 (SIG)"() -> (w3396:T2)
                n1953 = case shown="\"T-RISE TEST\"" w3401 {
                  tunnel: [FALSE FALSE TRUE] -> w3399
                  frame "TEST SET UP", Default {
                  }
                  frame "CYCLE TEST" {
                  }
                  frame "T-RISE TEST" {
                  }
                }
                n1954 = local read "LAB01-1 (SET)"() -> (w3389:T5)
                n1955 = Unbundle(w3396) -> ("AMPS"=w3395:dbl, "Tmp Live"=w3393:dbl, "Tmp Neut"=w3392:dbl)  [unwired: 2 out]
                n1956 = Unbundle(w3385) -> ("CYCLE"=w3384:dbl)  [unwired: 2 out]
                n1957 = Unbundle(w3394) -> ("TL"=w3391:dbl, "TN"=w3390:dbl)
                n1958 = local read "LAB01-1 (TDMS)"() -> (w3381:refnum<k34>)
                n1959 = Greater?(x=w3384, y=2.0) -> (0:w3383:bool)
                n1960 = And(x=w3400, y=w3383) -> (x .and. y?=w3397:bool)
                n1961 = Unbundle(w3389) -> ("T-RISE deg C"=w3386:dbl)  [unwired: 4 out]
                n1962 = Subtract(x=w3393, y=w3391) -> (x-y=w3388:dbl)
                n1963 = And(x=w3399, y=w3397) -> (x .and. y?=w3398:bool)
                n1964 = Subtract(x=w3392, y=w3390) -> (x-y=w3387:dbl)
                n1965 = case shown="True" w3398 {
                  tunnel: w3395 -> [_ w3418]
                  tunnel: w3388 -> [_ w3412]
                  tunnel: w3387 -> [_ w3411]
                  tunnel: w3386 -> [_ w3410]
                  tunnel: w3381 -> [_ w3403]
                  tunnel: w3380 -> [_ w3402]
                  frame False {
                  }
                  frame True {
                    # "check for amps & t-rise fail"
                    n1966 = Less?(x=w3418, y=w3402) -> (x < y?=w3405:bool)
                    n1967 = Greater?(x=w3412, y=w3410) -> (0:w3415:bool)
                    n1968 = Greater?(x=w3411, y=w3410) -> (0:w3416:bool)
                    n1969 = Or(x=w3415, y=w3416) -> (x .or. y?=w3404:bool)
                    n1970 = Select(t="AMPS LO", s=w3405, f="") -> (s? t:f=w3406:string)
                    n1971 = Select(t="T-RISE HI", s=w3404, f="") -> (s? t:f=w3407:string)
                    n1972 = Or(x=w3405, y=w3404) -> (x .or. y?=w3417:bool)
                    n1973 = case shown="True" w3417 {
                      tunnel: w3407 -> [_ w3421]
                      tunnel: w3406 -> [_ w3420]
                      tunnel: w3403 -> [_ w3419]
                      frame False {
                      }
                      frame True {
                        n1974 = stacked-sequence {
                          tunnel: w3421 -> [w3424 _]
                          tunnel: w3420 -> [w3423 _]
                          tunnel: w3419 -> [w3422 _]
                          frame #0 {
                            n1975 = Build Array(w3423, w3424) -> (w3426:string[])
                            n1976 = TDMS Write(0:w3422, 5:"TEST RESULT", 7:"T-RISE FAIL ", 9:w3426) -> (15:w3428:errorcluster)  [unwired: 2 in, 3 out]
                            n1977 = local write "data file error"(w3428) -> ()
                          }
                          frame #1 {
                            n1978 = local read "LAB01-1 (DISP)"() -> (w3432:T4)
                            n1979 = Bundle(cluster=w3432, "STATUS"="STOP") -> (w3431:T4)  [unwired: 2 in]
                            n1980 = local write "LAB01-1 (RESULT)"(FALSE) -> ()
                            n1981 = local write "LAB01-1 (DISP)"(w3431) -> ()
                          }
                        }
                      }
                    }
                  }
                }
              }
              frame #1 {
                # "LAB01-2"
                n1982 = local read "LAB01-2 (TEMP START)"() -> (w3452:cluster{"TL":dbl, "TN":dbl})
                n1983 = local read "LAB01-2 (DISP)"() -> (w3443:T4)
                n1984 = local read "LAB01-2 (SIG)"() -> (w3454:T2)
                n1985 = case shown="\"T-RISE TEST\"" w3438 {
                  tunnel: [FALSE FALSE TRUE] -> w3457
                  frame "TEST SET UP", Default {
                  }
                  frame "CYCLE TEST" {
                  }
                  frame "T-RISE TEST" {
                  }
                }
                n1986 = local read "LAB01-2(SET)"() -> (w3447:T5)
                n1987 = Unbundle(w3454) -> ("AMPS"=w3453:dbl, "Tmp Live"=w3451:dbl, "Tmp Neut"=w3450:dbl)  [unwired: 2 out]
                n1988 = Unbundle(w3443) -> ("CYCLE"=w3442:dbl)  [unwired: 2 out]
                n1989 = Unbundle(w3452) -> ("TL"=w3449:dbl, "TN"=w3448:dbl)
                n1990 = local read "LAB01-2 (TDMS)"() -> (w3439:refnum<k34>)
                n1991 = Greater?(x=w3442, y=2.0) -> (0:w3441:bool)
                n1992 = And(x=w3437, y=w3441) -> (x .and. y?=w3455:bool)
                n1993 = Unbundle(w3447) -> ("T-RISE deg C"=w3444:dbl)  [unwired: 4 out]
                n1994 = Subtract(x=w3451, y=w3449) -> (x-y=w3446:dbl)
                n1995 = And(x=w3457, y=w3455) -> (x .and. y?=w3456:bool)
                n1996 = Subtract(x=w3450, y=w3448) -> (x-y=w3445:dbl)
                n1997 = case shown="True" w3456 {
                  tunnel: w3453 -> [_ w3474]
                  tunnel: w3446 -> [_ w3468]
                  tunnel: w3445 -> [_ w3467]
                  tunnel: w3444 -> [_ w3466]
                  tunnel: w3439 -> [_ w3459]
                  tunnel: w3436 -> [_ w3458]
                  frame False {
                  }
                  frame True {
                    # "check for amps & t-rise fail"
                    n1998 = Less?(x=w3474, y=w3458) -> (x < y?=w3461:bool)
                    n1999 = Greater?(x=w3468, y=w3466) -> (0:w3471:bool)
                    n2000 = Greater?(x=w3467, y=w3466) -> (0:w3472:bool)
                    n2001 = Or(x=w3471, y=w3472) -> (x .or. y?=w3460:bool)
                    n2002 = Select(t="AMPS LO", s=w3461, f="") -> (s? t:f=w3462:string)
                    n2003 = Select(t="T-RISE HI", s=w3460, f="") -> (s? t:f=w3463:string)
                    n2004 = Or(x=w3461, y=w3460) -> (x .or. y?=w3473:bool)
                    n2005 = case shown="True" w3473 {
                      tunnel: w3463 -> [_ w3477]
                      tunnel: w3462 -> [_ w3476]
                      tunnel: w3459 -> [_ w3475]
                      frame False {
                      }
                      frame True {
                        n2006 = stacked-sequence {
                          tunnel: w3477 -> [w3480 _]
                          tunnel: w3476 -> [w3479 _]
                          tunnel: w3475 -> [w3478 _]
                          frame #0 {
                            n2007 = Build Array(w3479, w3480) -> (w3482:string[])
                            n2008 = TDMS Write(0:w3478, 5:"TEST RESULT", 7:"T-RISE FAIL ", 9:w3482) -> (15:w3484:errorcluster)  [unwired: 2 in, 3 out]
                            n2009 = local write "data file error"(w3484) -> ()
                          }
                          frame #1 {
                            n2010 = local read "LAB01-2 (DISP)"() -> (w3488:T4)
                            n2011 = Bundle(cluster=w3488, "STATUS"="STOP") -> (w3487:T4)  [unwired: 2 in]
                            n2012 = local write "LAB01-2 (RESULT)"(FALSE) -> ()
                            n2013 = local write "LAB01-2 (DISP)"(w3487) -> ()
                          }
                        }
                      }
                    }
                  }
                }
              }
              frame #2 {
                # "LAB02-1"
                n2014 = local read "LAB02-1 (TEMP START)"() -> (w3508:cluster{"TL":dbl, "TN":dbl})
                n2015 = local read "LAB02-1 (DISP)"() -> (w3499:T4)
                n2016 = local read "LAB02-1 (SIG)"() -> (w3510:T2)
                n2017 = case shown="\"T-RISE TEST\"" w3494 {
                  tunnel: [FALSE FALSE TRUE] -> w3513
                  frame "TEST SET UP", Default {
                  }
                  frame "CYCLE TEST" {
                  }
                  frame "T-RISE TEST" {
                  }
                }
                n2018 = local read "LAB02-1 (SET)"() -> (w3503:T5)
                n2019 = Unbundle(w3510) -> ("AMPS"=w3509:dbl, "Tmp Live"=w3507:dbl, "Tmp Neut"=w3506:dbl)  [unwired: 2 out]
                n2020 = Unbundle(w3499) -> ("CYCLE"=w3498:dbl)  [unwired: 2 out]
                n2021 = Unbundle(w3508) -> ("TL"=w3505:dbl, "TN"=w3504:dbl)
                n2022 = local read "LAB02-1 (TDMS)"() -> (w3495:refnum<k34>)
                n2023 = Greater?(x=w3498, y=2.0) -> (0:w3497:bool)
                n2024 = And(x=w3493, y=w3497) -> (x .and. y?=w3511:bool)
                n2025 = Unbundle(w3503) -> ("T-RISE deg C"=w3500:dbl)  [unwired: 4 out]
                n2026 = Subtract(x=w3507, y=w3505) -> (x-y=w3502:dbl)
                n2027 = And(x=w3513, y=w3511) -> (x .and. y?=w3512:bool)
                n2028 = Subtract(x=w3506, y=w3504) -> (x-y=w3501:dbl)
                n2029 = case shown="True" w3512 {
                  tunnel: w3509 -> [_ w3530]
                  tunnel: w3502 -> [_ w3524]
                  tunnel: w3501 -> [_ w3523]
                  tunnel: w3500 -> [_ w3522]
                  tunnel: w3495 -> [_ w3515]
                  tunnel: w3492 -> [_ w3514]
                  frame False {
                  }
                  frame True {
                    # "check for amps & t-rise fail"
                    n2030 = Less?(x=w3530, y=w3514) -> (x < y?=w3517:bool)
                    n2031 = Greater?(x=w3524, y=w3522) -> (0:w3527:bool)
                    n2032 = Greater?(x=w3523, y=w3522) -> (0:w3528:bool)
                    n2033 = Or(x=w3527, y=w3528) -> (x .or. y?=w3516:bool)
                    n2034 = Select(t="AMPS LO", s=w3517, f="") -> (s? t:f=w3518:string)
                    n2035 = Select(t="T-RISE HI", s=w3516, f="") -> (s? t:f=w3519:string)
                    n2036 = Or(x=w3517, y=w3516) -> (x .or. y?=w3529:bool)
                    n2037 = case shown="True" w3529 {
                      tunnel: w3519 -> [_ w3533]
                      tunnel: w3518 -> [_ w3532]
                      tunnel: w3515 -> [_ w3531]
                      frame False {
                      }
                      frame True {
                        n2038 = stacked-sequence {
                          tunnel: w3533 -> [w3536 _]
                          tunnel: w3532 -> [w3535 _]
                          tunnel: w3531 -> [w3534 _]
                          frame #0 {
                            n2039 = Build Array(w3535, w3536) -> (w3538:string[])
                            n2040 = TDMS Write(0:w3534, 5:"TEST RESULT", 7:"T-RISE FAIL ", 9:w3538) -> (15:w3540:errorcluster)  [unwired: 2 in, 3 out]
                            n2041 = local write "data file error"(w3540) -> ()
                          }
                          frame #1 {
                            n2042 = local read "LAB02-1 (DISP)"() -> (w3544:T4)
                            n2043 = Bundle(cluster=w3544, "STATUS"="STOP") -> (w3543:T4)  [unwired: 2 in]
                            n2044 = local write "LAB02-1 (RESULT)"(FALSE) -> ()
                            n2045 = local write "LAB02-1 (DISP)"(w3543) -> ()
                          }
                        }
                      }
                    }
                  }
                }
              }
              frame #3 {
                # "LAB02-2"
                n2046 = local read "LAB02-2 (TEMP START)"() -> (w3564:cluster{"TL":dbl, "TN":dbl})
                n2047 = local read "LAB02-2 (DISP)"() -> (w3555:T4)
                n2048 = local read "LAB02-2 (SIG)"() -> (w3566:T2)
                n2049 = case shown="\"T-RISE TEST\"" w3550 {
                  tunnel: [FALSE FALSE TRUE] -> w3569
                  frame "TEST SET UP", Default {
                  }
                  frame "CYCLE TEST" {
                  }
                  frame "T-RISE TEST" {
                  }
                }
                n2050 = local read "LAB02-2 (SET)"() -> (w3559:T5)
                n2051 = Unbundle(w3566) -> ("AMPS"=w3565:dbl, "Tmp Live"=w3563:dbl, "Tmp Neut"=w3562:dbl)  [unwired: 2 out]
                n2052 = Unbundle(w3555) -> ("CYCLE"=w3554:dbl)  [unwired: 2 out]
                n2053 = Unbundle(w3564) -> ("TL"=w3561:dbl, "TN"=w3560:dbl)
                n2054 = local read "LAB02-2 (TDMS)"() -> (w3551:refnum<k34>)
                n2055 = Greater?(x=w3554, y=2.0) -> (0:w3553:bool)
                n2056 = And(x=w3549, y=w3553) -> (x .and. y?=w3567:bool)
                n2057 = Unbundle(w3559) -> ("T-RISE deg C"=w3556:dbl)  [unwired: 4 out]
                n2058 = Subtract(x=w3563, y=w3561) -> (x-y=w3558:dbl)
                n2059 = And(x=w3569, y=w3567) -> (x .and. y?=w3568:bool)
                n2060 = Subtract(x=w3562, y=w3560) -> (x-y=w3557:dbl)
                n2061 = case shown="True" w3568 {
                  tunnel: w3565 -> [_ w3586]
                  tunnel: w3558 -> [_ w3580]
                  tunnel: w3557 -> [_ w3579]
                  tunnel: w3556 -> [_ w3578]
                  tunnel: w3551 -> [_ w3571]
                  tunnel: w3548 -> [_ w3570]
                  frame False {
                  }
                  frame True {
                    # "check for amps & t-rise fail"
                    n2062 = Less?(x=w3586, y=w3570) -> (x < y?=w3573:bool)
                    n2063 = Greater?(x=w3580, y=w3578) -> (0:w3583:bool)
                    n2064 = Greater?(x=w3579, y=w3578) -> (0:w3584:bool)
                    n2065 = Or(x=w3583, y=w3584) -> (x .or. y?=w3572:bool)
                    n2066 = Select(t="AMPS LO", s=w3573, f="") -> (s? t:f=w3574:string)
                    n2067 = Select(t="T-RISE HI", s=w3572, f="") -> (s? t:f=w3575:string)
                    n2068 = Or(x=w3573, y=w3572) -> (x .or. y?=w3585:bool)
                    n2069 = case shown="True" w3585 {
                      tunnel: w3575 -> [_ w3589]
                      tunnel: w3574 -> [_ w3588]
                      tunnel: w3571 -> [_ w3587]
                      frame False {
                      }
                      frame True {
                        n2070 = stacked-sequence {
                          tunnel: w3589 -> [w3592 _]
                          tunnel: w3588 -> [w3591 _]
                          tunnel: w3587 -> [w3590 _]
                          frame #0 {
                            n2071 = Build Array(w3591, w3592) -> (w3594:string[])
                            n2072 = TDMS Write(0:w3590, 5:"TEST RESULT", 7:"T-RISE FAIL ", 9:w3594) -> (15:w3596:errorcluster)  [unwired: 2 in, 3 out]
                            n2073 = local write "data file error"(w3596) -> ()
                          }
                          frame #1 {
                            n2074 = local read "LAB02-2 (DISP)"() -> (w3600:T4)
                            n2075 = Bundle(cluster=w3600, "STATUS"="STOP") -> (w3599:T4)  [unwired: 2 in]
                            n2076 = local write "LAB02-2 (RESULT)"(FALSE) -> ()
                            n2077 = local write "LAB02-2 (DISP)"(w3599) -> ()
                          }
                        }
                      }
                    }
                  }
                }
              }
              frame #4 {
                # "LAB03-1"
                n2078 = local read "LAB03-1 (TEMP START)"() -> (w3620:cluster{"TL":dbl, "TN":dbl})
                n2079 = local read "LAB03-1 (DISP)"() -> (w3611:T4)
                n2080 = local read "LAB03-1 (SIG)"() -> (w3622:T2)
                n2081 = case shown="\"T-RISE TEST\"" w3606 {
                  tunnel: [FALSE FALSE TRUE] -> w3625
                  frame "TEST SET UP", Default {
                  }
                  frame "CYCLE TEST" {
                  }
                  frame "T-RISE TEST" {
                  }
                }
                n2082 = local read "LAB03-1 (SET)"() -> (w3615:T5)
                n2083 = Unbundle(w3622) -> ("AMPS"=w3621:dbl, "Tmp Live"=w3619:dbl, "Tmp Neut"=w3618:dbl)  [unwired: 2 out]
                n2084 = Unbundle(w3611) -> ("CYCLE"=w3610:dbl)  [unwired: 2 out]
                n2085 = Unbundle(w3620) -> ("TL"=w3617:dbl, "TN"=w3616:dbl)
                n2086 = local read "LAB03-1 (TDMS)"() -> (w3607:refnum<k34>)
                n2087 = Greater?(x=w3610, y=2.0) -> (0:w3609:bool)
                n2088 = And(x=w3605, y=w3609) -> (x .and. y?=w3623:bool)
                n2089 = Unbundle(w3615) -> ("T-RISE deg C"=w3612:dbl)  [unwired: 4 out]
                n2090 = Subtract(x=w3619, y=w3617) -> (x-y=w3614:dbl)
                n2091 = And(x=w3625, y=w3623) -> (x .and. y?=w3624:bool)
                n2092 = Subtract(x=w3618, y=w3616) -> (x-y=w3613:dbl)
                n2093 = case shown="True" w3624 {
                  tunnel: w3621 -> [_ w3642]
                  tunnel: w3614 -> [_ w3636]
                  tunnel: w3613 -> [_ w3635]
                  tunnel: w3612 -> [_ w3634]
                  tunnel: w3607 -> [_ w3627]
                  tunnel: w3604 -> [_ w3626]
                  frame False {
                  }
                  frame True {
                    # "check for amps & t-rise fail"
                    n2094 = Less?(x=w3642, y=w3626) -> (x < y?=w3629:bool)
                    n2095 = Greater?(x=w3636, y=w3634) -> (0:w3639:bool)
                    n2096 = Greater?(x=w3635, y=w3634) -> (0:w3640:bool)
                    n2097 = Or(x=w3639, y=w3640) -> (x .or. y?=w3628:bool)
                    n2098 = Select(t="AMPS LO", s=w3629, f="") -> (s? t:f=w3630:string)
                    n2099 = Select(t="T-RISE HI", s=w3628, f="") -> (s? t:f=w3631:string)
                    n2100 = Or(x=w3629, y=w3628) -> (x .or. y?=w3641:bool)
                    n2101 = case shown="True" w3641 {
                      tunnel: w3631 -> [_ w3645]
                      tunnel: w3630 -> [_ w3644]
                      tunnel: w3627 -> [_ w3643]
                      frame False {
                      }
                      frame True {
                        n2102 = stacked-sequence {
                          tunnel: w3645 -> [w3648 _]
                          tunnel: w3644 -> [w3647 _]
                          tunnel: w3643 -> [w3646 _]
                          frame #0 {
                            n2103 = Build Array(w3647, w3648) -> (w3650:string[])
                            n2104 = TDMS Write(0:w3646, 5:"TEST RESULT", 7:"T-RISE FAIL ", 9:w3650) -> (15:w3652:errorcluster)  [unwired: 2 in, 3 out]
                            n2105 = local write "data file error"(w3652) -> ()
                          }
                          frame #1 {
                            n2106 = local read "LAB03-1 (DISP)"() -> (w3656:T4)
                            n2107 = Bundle(cluster=w3656, "STATUS"="STOP") -> (w3655:T4)  [unwired: 2 in]
                            n2108 = local write "LAB03-1 (RESULT)"(FALSE) -> ()
                            n2109 = local write "LAB03-1 (DISP)"(w3655) -> ()
                          }
                        }
                      }
                    }
                  }
                }
              }
              frame #5 {
                # "LAB03-2"
                n2110 = local read "LAB03-2 (TEMP START)"() -> (w3676:cluster{"TL":dbl, "TN":dbl})
                n2111 = local read "LAB03-2 (SIG)"() -> (w3678:T2)
                n2112 = local read "LAB03-2 (DISP)"() -> (w3667:T4)
                n2113 = case shown="\"T-RISE TEST\"" w3662 {
                  tunnel: [FALSE FALSE TRUE] -> w3681
                  frame "TEST SET UP", Default {
                  }
                  frame "CYCLE TEST" {
                  }
                  frame "T-RISE TEST" {
                  }
                }
                n2114 = local read "LAB03-2 (SET)"() -> (w3671:T5)
                n2115 = Unbundle(w3678) -> ("AMPS"=w3677:dbl, "Tmp Live"=w3675:dbl, "Tmp Neut"=w3674:dbl)  [unwired: 2 out]
                n2116 = Unbundle(w3667) -> ("CYCLE"=w3666:dbl)  [unwired: 2 out]
                n2117 = Unbundle(w3676) -> ("TL"=w3673:dbl, "TN"=w3672:dbl)
                n2118 = local read "LAB03-2 (TDMS)"() -> (w3663:refnum<k34>)
                n2119 = Greater?(x=w3666, y=2.0) -> (0:w3665:bool)
                n2120 = And(x=w3661, y=w3665) -> (x .and. y?=w3679:bool)
                n2121 = Unbundle(w3671) -> ("T-RISE deg C"=w3668:dbl)  [unwired: 4 out]
                n2122 = Subtract(x=w3675, y=w3673) -> (x-y=w3670:dbl)
                n2123 = And(x=w3681, y=w3679) -> (x .and. y?=w3680:bool)
                n2124 = Subtract(x=w3674, y=w3672) -> (x-y=w3669:dbl)
                n2125 = case shown="True" w3680 {
                  tunnel: w3677 -> [_ w3698]
                  tunnel: w3670 -> [_ w3692]
                  tunnel: w3669 -> [_ w3691]
                  tunnel: w3668 -> [_ w3690]
                  tunnel: w3663 -> [_ w3683]
                  tunnel: w3660 -> [_ w3682]
                  frame False {
                  }
                  frame True {
                    # "check for amps & t-rise fail"
                    n2126 = Less?(x=w3698, y=w3682) -> (x < y?=w3685:bool)
                    n2127 = Greater?(x=w3692, y=w3690) -> (0:w3695:bool)
                    n2128 = Greater?(x=w3691, y=w3690) -> (0:w3696:bool)
                    n2129 = Or(x=w3695, y=w3696) -> (x .or. y?=w3684:bool)
                    n2130 = Select(t="AMPS LO", s=w3685, f="") -> (s? t:f=w3686:string)
                    n2131 = Select(t="T-RISE HI", s=w3684, f="") -> (s? t:f=w3687:string)
                    n2132 = Or(x=w3685, y=w3684) -> (x .or. y?=w3697:bool)
                    n2133 = case shown="True" w3697 {
                      tunnel: w3687 -> [_ w3701]
                      tunnel: w3686 -> [_ w3700]
                      tunnel: w3683 -> [_ w3699]
                      frame False {
                      }
                      frame True {
                        n2134 = stacked-sequence {
                          tunnel: w3701 -> [w3704 _]
                          tunnel: w3700 -> [w3703 _]
                          tunnel: w3699 -> [w3702 _]
                          frame #0 {
                            n2135 = Build Array(w3703, w3704) -> (w3706:string[])
                            n2136 = TDMS Write(0:w3702, 5:"TEST RESULT", 7:"T-RISE FAIL ", 9:w3706) -> (15:w3708:errorcluster)  [unwired: 2 in, 3 out]
                            n2137 = local write "data file error"(w3708) -> ()
                          }
                          frame #1 {
                            n2138 = local read "LAB03-2 (DISP)"() -> (w3712:T4)
                            n2139 = Bundle(cluster=w3712, "STATUS"="STOP") -> (w3711:T4)  [unwired: 2 in]
                            n2140 = local write "LAB03-2 (RESULT)"(FALSE) -> ()
                            n2141 = local write "LAB03-2 (DISP)"(w3711) -> ()
                          }
                        }
                      }
                    }
                  }
                }
              }
              frame #6 {
                # "LAB04-1"
                n2142 = local read "LAB04-1 (TEMP START)"() -> (w3732:cluster{"TL":dbl, "TN":dbl})
                n2143 = local read "LAB04-1 (SIG)"() -> (w3734:T2)
                n2144 = local read "LAB04-1 (DISP)"() -> (w3723:T4)
                n2145 = case shown="\"T-RISE TEST\"" w3718 {
                  tunnel: [FALSE FALSE TRUE] -> w3737
                  frame "TEST SET UP", Default {
                  }
                  frame "CYCLE TEST" {
                  }
                  frame "T-RISE TEST" {
                  }
                }
                n2146 = local read "LAB04-1 (SET)"() -> (w3727:T5)
                n2147 = Unbundle(w3734) -> ("AMPS"=w3733:dbl, "Tmp Live"=w3731:dbl, "Tmp Neut"=w3730:dbl)  [unwired: 2 out]
                n2148 = Unbundle(w3723) -> ("CYCLE"=w3722:dbl)  [unwired: 2 out]
                n2149 = Unbundle(w3732) -> ("TL"=w3729:dbl, "TN"=w3728:dbl)
                n2150 = local read "LAB04-1 (TDMS)"() -> (w3719:refnum<k34>)
                n2151 = Greater?(x=w3722, y=2.0) -> (0:w3721:bool)
                n2152 = And(x=w3717, y=w3721) -> (x .and. y?=w3735:bool)
                n2153 = Unbundle(w3727) -> ("T-RISE deg C"=w3724:dbl)  [unwired: 4 out]
                n2154 = Subtract(x=w3731, y=w3729) -> (x-y=w3726:dbl)
                n2155 = And(x=w3737, y=w3735) -> (x .and. y?=w3736:bool)
                n2156 = Subtract(x=w3730, y=w3728) -> (x-y=w3725:dbl)
                n2157 = case shown="True" w3736 {
                  tunnel: w3733 -> [_ w3754]
                  tunnel: w3726 -> [_ w3748]
                  tunnel: w3725 -> [_ w3747]
                  tunnel: w3724 -> [_ w3746]
                  tunnel: w3719 -> [_ w3739]
                  tunnel: w3716 -> [_ w3738]
                  frame False {
                  }
                  frame True {
                    # "check for amps & t-rise fail"
                    n2158 = Less?(x=w3754, y=w3738) -> (x < y?=w3741:bool)
                    n2159 = Greater?(x=w3748, y=w3746) -> (0:w3751:bool)
                    n2160 = Greater?(x=w3747, y=w3746) -> (0:w3752:bool)
                    n2161 = Or(x=w3751, y=w3752) -> (x .or. y?=w3740:bool)
                    n2162 = Select(t="AMPS LO", s=w3741, f="") -> (s? t:f=w3742:string)
                    n2163 = Select(t="T-RISE HI", s=w3740, f="") -> (s? t:f=w3743:string)
                    n2164 = Or(x=w3741, y=w3740) -> (x .or. y?=w3753:bool)
                    n2165 = case shown="True" w3753 {
                      tunnel: w3743 -> [_ w3757]
                      tunnel: w3742 -> [_ w3756]
                      tunnel: w3739 -> [_ w3755]
                      frame False {
                      }
                      frame True {
                        n2166 = stacked-sequence {
                          tunnel: w3757 -> [w3760 _]
                          tunnel: w3756 -> [w3759 _]
                          tunnel: w3755 -> [w3758 _]
                          frame #0 {
                            n2167 = Build Array(w3759, w3760) -> (w3762:string[])
                            n2168 = TDMS Write(0:w3758, 5:"TEST RESULT", 7:"T-RISE FAIL ", 9:w3762) -> (15:w3764:errorcluster)  [unwired: 2 in, 3 out]
                            n2169 = local write "data file error"(w3764) -> ()
                          }
                          frame #1 {
                            n2170 = local read "LAB04-1 (DISP)"() -> (w3768:T4)
                            n2171 = Bundle(cluster=w3768, "STATUS"="STOP") -> (w3767:T4)  [unwired: 2 in]
                            n2172 = local write "LAB04-1 (RESULT)"(FALSE) -> ()
                            n2173 = local write "LAB04-1 (DISP)"(w3767) -> ()
                          }
                        }
                      }
                    }
                  }
                }
              }
              frame #7 {
                # "LAB04-2"
                n2174 = local read "LAB04-2 (TEMP START)"() -> (w3788:cluster{"TL":dbl, "TN":dbl})
                n2175 = local read "LAB04-2 (SIG)"() -> (w3790:T2)
                n2176 = local read "LAB04-2 (DISP)"() -> (w3779:T4)
                n2177 = case shown="\"T-RISE TEST\"" w3774 {
                  tunnel: [FALSE FALSE TRUE] -> w3793
                  frame "TEST SET UP", Default {
                  }
                  frame "CYCLE TEST" {
                  }
                  frame "T-RISE TEST" {
                  }
                }
                n2178 = local read "LAB04-2 (SET)"() -> (w3783:T5)
                n2179 = Unbundle(w3790) -> ("AMPS"=w3789:dbl, "Tmp Live"=w3787:dbl, "Tmp Neut"=w3786:dbl)  [unwired: 2 out]
                n2180 = Unbundle(w3779) -> ("CYCLE"=w3778:dbl)  [unwired: 2 out]
                n2181 = Unbundle(w3788) -> ("TL"=w3785:dbl, "TN"=w3784:dbl)
                n2182 = local read "LAB04-2 (TDMS)"() -> (w3775:refnum<k34>)
                n2183 = Greater?(x=w3778, y=2.0) -> (0:w3777:bool)
                n2184 = And(x=w3773, y=w3777) -> (x .and. y?=w3791:bool)
                n2185 = Unbundle(w3783) -> ("T-RISE deg C"=w3780:dbl)  [unwired: 4 out]
                n2186 = Subtract(x=w3787, y=w3785) -> (x-y=w3782:dbl)
                n2187 = And(x=w3793, y=w3791) -> (x .and. y?=w3792:bool)
                n2188 = Subtract(x=w3786, y=w3784) -> (x-y=w3781:dbl)
                n2189 = case shown="True" w3792 {
                  tunnel: w3789 -> [_ w3810]
                  tunnel: w3782 -> [_ w3804]
                  tunnel: w3781 -> [_ w3803]
                  tunnel: w3780 -> [_ w3802]
                  tunnel: w3775 -> [_ w3795]
                  tunnel: w3772 -> [_ w3794]
                  frame False {
                  }
                  frame True {
                    # "check for amps & t-rise fail"
                    n2190 = Less?(x=w3810, y=w3794) -> (x < y?=w3797:bool)
                    n2191 = Greater?(x=w3804, y=w3802) -> (0:w3807:bool)
                    n2192 = Greater?(x=w3803, y=w3802) -> (0:w3808:bool)
                    n2193 = Or(x=w3807, y=w3808) -> (x .or. y?=w3796:bool)
                    n2194 = Select(t="AMPS LO", s=w3797, f="") -> (s? t:f=w3798:string)
                    n2195 = Select(t="T-RISE HI", s=w3796, f="") -> (s? t:f=w3799:string)
                    n2196 = Or(x=w3797, y=w3796) -> (x .or. y?=w3809:bool)
                    n2197 = case shown="True" w3809 {
                      tunnel: w3799 -> [_ w3813]
                      tunnel: w3798 -> [_ w3812]
                      tunnel: w3795 -> [_ w3811]
                      frame False {
                      }
                      frame True {
                        n2198 = stacked-sequence {
                          tunnel: w3813 -> [w3816 _]
                          tunnel: w3812 -> [w3815 _]
                          tunnel: w3811 -> [w3814 _]
                          frame #0 {
                            n2199 = Build Array(w3815, w3816) -> (w3818:string[])
                            n2200 = TDMS Write(0:w3814, 5:"TEST RESULT", 7:"T-RISE FAIL ", 9:w3818) -> (15:w3820:errorcluster)  [unwired: 2 in, 3 out]
                            n2201 = local write "data file error"(w3820) -> ()
                          }
                          frame #1 {
                            n2202 = local read "LAB04-2 (DISP)"() -> (w3824:T4)
                            n2203 = Bundle(cluster=w3824, "STATUS"="STOP") -> (w3823:T4)  [unwired: 2 in]
                            n2204 = local write "LAB04-2 (RESULT)"(FALSE) -> ()
                            n2205 = local write "LAB04-2 (DISP)"(w3823) -> ()
                          }
                        }
                      }
                    }
                  }
                }
              }
              frame #8 {
                # "LAB05-1"
                n2206 = local read "LAB05-1 (TEMP START)"() -> (w3844:cluster{"TL":dbl, "TN":dbl})
                n2207 = local read "LAB05-1 (SIG)"() -> (w3846:T2)
                n2208 = local read "LAB05-1 (DISP)"() -> (w3835:T4)
                n2209 = case shown="\"T-RISE TEST\"" w3830 {
                  tunnel: [FALSE FALSE TRUE] -> w3849
                  frame "TEST SET UP", Default {
                  }
                  frame "CYCLE TEST" {
                  }
                  frame "T-RISE TEST" {
                  }
                }
                n2210 = local read "LAB05-1 (SET)"() -> (w3839:T5)
                n2211 = Unbundle(w3846) -> ("AMPS"=w3845:dbl, "Tmp Live"=w3843:dbl, "Tmp Neut"=w3842:dbl)  [unwired: 2 out]
                n2212 = Unbundle(w3835) -> ("CYCLE"=w3834:dbl)  [unwired: 2 out]
                n2213 = Unbundle(w3844) -> ("TL"=w3841:dbl, "TN"=w3840:dbl)
                n2214 = local read "LAB05-1 (TDMS)"() -> (w3831:refnum<k34>)
                n2215 = Greater?(x=w3834, y=2.0) -> (0:w3833:bool)
                n2216 = And(x=w3829, y=w3833) -> (x .and. y?=w3847:bool)
                n2217 = Unbundle(w3839) -> ("T-RISE deg C"=w3836:dbl)  [unwired: 4 out]
                n2218 = Subtract(x=w3843, y=w3841) -> (x-y=w3838:dbl)
                n2219 = And(x=w3849, y=w3847) -> (x .and. y?=w3848:bool)
                n2220 = Subtract(x=w3842, y=w3840) -> (x-y=w3837:dbl)
                n2221 = case shown="True" w3848 {
                  tunnel: w3845 -> [_ w3866]
                  tunnel: w3838 -> [_ w3860]
                  tunnel: w3837 -> [_ w3859]
                  tunnel: w3836 -> [_ w3858]
                  tunnel: w3831 -> [_ w3851]
                  tunnel: w3828 -> [_ w3850]
                  frame False {
                  }
                  frame True {
                    # "check for amps & t-rise fail"
                    n2222 = Less?(x=w3866, y=w3850) -> (x < y?=w3853:bool)
                    n2223 = Greater?(x=w3860, y=w3858) -> (0:w3863:bool)
                    n2224 = Greater?(x=w3859, y=w3858) -> (0:w3864:bool)
                    n2225 = Or(x=w3863, y=w3864) -> (x .or. y?=w3852:bool)
                    n2226 = Select(t="AMPS LO", s=w3853, f="") -> (s? t:f=w3854:string)
                    n2227 = Select(t="T-RISE HI", s=w3852, f="") -> (s? t:f=w3855:string)
                    n2228 = Or(x=w3853, y=w3852) -> (x .or. y?=w3865:bool)
                    n2229 = case shown="True" w3865 {
                      tunnel: w3855 -> [_ w3869]
                      tunnel: w3854 -> [_ w3868]
                      tunnel: w3851 -> [_ w3867]
                      frame False {
                      }
                      frame True {
                        n2230 = stacked-sequence {
                          tunnel: w3869 -> [w3872 _]
                          tunnel: w3868 -> [w3871 _]
                          tunnel: w3867 -> [w3870 _]
                          frame #0 {
                            n2231 = Build Array(w3871, w3872) -> (w3874:string[])
                            n2232 = TDMS Write(0:w3870, 5:"TEST RESULT", 7:"T-RISE FAIL ", 9:w3874) -> (15:w3876:errorcluster)  [unwired: 2 in, 3 out]
                            n2233 = local write "data file error"(w3876) -> ()
                          }
                          frame #1 {
                            n2234 = local read "LAB05-1 (DISP)"() -> (w3880:T4)
                            n2235 = Bundle(cluster=w3880, "STATUS"="STOP") -> (w3879:T4)  [unwired: 2 in]
                            n2236 = local write "LAB05-1 (RESULT)"(FALSE) -> ()
                            n2237 = local write "LAB05-1 (DISP)"(w3879) -> ()
                          }
                        }
                      }
                    }
                  }
                }
              }
              frame #9 {
                # "LAB05-2"
                n2238 = local read "LAB05-2 (TEMP START)"() -> (w3900:cluster{"TL":dbl, "TN":dbl})
                n2239 = local read "LAB05-2 (DISP)"() -> (w3891:T4)
                n2240 = local read "LAB05-2 (SIG)"() -> (w3902:T2)
                n2241 = case shown="\"T-RISE TEST\"" w3886 {
                  tunnel: [FALSE FALSE TRUE] -> w3905
                  frame "TEST SET UP", Default {
                  }
                  frame "CYCLE TEST" {
                  }
                  frame "T-RISE TEST" {
                  }
                }
                n2242 = local read "LAB05-2 (SET)"() -> (w3895:T5)
                n2243 = Unbundle(w3891) -> ("CYCLE"=w3890:dbl)  [unwired: 2 out]
                n2244 = Unbundle(w3902) -> ("AMPS"=w3901:dbl, "Tmp Live"=w3899:dbl, "Tmp Neut"=w3898:dbl)  [unwired: 2 out]
                n2245 = Unbundle(w3900) -> ("TL"=w3897:dbl, "TN"=w3896:dbl)
                n2246 = Greater?(x=w3890, y=2.0) -> (0:w3889:bool)
                n2247 = local read "LAB05-2 (TDMS)"() -> (w3887:refnum<k34>)
                n2248 = And(x=w3885, y=w3889) -> (x .and. y?=w3903:bool)
                n2249 = Unbundle(w3895) -> ("T-RISE deg C"=w3892:dbl)  [unwired: 4 out]
                n2250 = Subtract(x=w3899, y=w3897) -> (x-y=w3894:dbl)
                n2251 = And(x=w3905, y=w3903) -> (x .and. y?=w3904:bool)
                n2252 = Subtract(x=w3898, y=w3896) -> (x-y=w3893:dbl)
                n2253 = case shown="True" w3904 {
                  tunnel: w3901 -> [_ w3922]
                  tunnel: w3894 -> [_ w3916]
                  tunnel: w3893 -> [_ w3915]
                  tunnel: w3892 -> [_ w3914]
                  tunnel: w3887 -> [_ w3907]
                  tunnel: w3884 -> [_ w3906]
                  frame False {
                  }
                  frame True {
                    # "check for amps & t-rise fail"
                    n2254 = Less?(x=w3922, y=w3906) -> (x < y?=w3909:bool)
                    n2255 = Greater?(x=w3916, y=w3914) -> (0:w3919:bool)
                    n2256 = Greater?(x=w3915, y=w3914) -> (0:w3920:bool)
                    n2257 = Or(x=w3919, y=w3920) -> (x .or. y?=w3908:bool)
                    n2258 = Select(t="AMPS LO", s=w3909, f="") -> (s? t:f=w3910:string)
                    n2259 = Select(t="T-RISE HI", s=w3908, f="") -> (s? t:f=w3911:string)
                    n2260 = Or(x=w3909, y=w3908) -> (x .or. y?=w3921:bool)
                    n2261 = case shown="True" w3921 {
                      tunnel: w3911 -> [_ w3925]
                      tunnel: w3910 -> [_ w3924]
                      tunnel: w3907 -> [_ w3923]
                      frame False {
                      }
                      frame True {
                        n2262 = stacked-sequence {
                          tunnel: w3925 -> [w3928 _]
                          tunnel: w3924 -> [w3927 _]
                          tunnel: w3923 -> [w3926 _]
                          frame #0 {
                            n2263 = Build Array(w3927, w3928) -> (w3930:string[])
                            n2264 = TDMS Write(0:w3926, 5:"TEST RESULT", 7:"T-RISE FAIL ", 9:w3930) -> (15:w3932:errorcluster)  [unwired: 2 in, 3 out]
                            n2265 = local write "data file error"(w3932) -> ()
                          }
                          frame #1 {
                            n2266 = local read "LAB05-2 (DISP)"() -> (w3936:T4)
                            n2267 = Bundle(cluster=w3936, "STATUS"="STOP") -> (w3935:T4)  [unwired: 2 in]
                            n2268 = local write "LAB05-2 (RESULT)"(FALSE) -> ()
                            n2269 = local write "LAB05-2 (DISP)"(w3935) -> ()
                          }
                        }
                      }
                    }
                  }
                }
              }
            }
          }
          frame #15 {
            # "run calibration routine"
            n2270 = local read "CALIBRATE"() -> (w3940:bool)
            n2271 = case shown="True" w3940 {
              frame False {
              }
              frame True {
                n2272 = stacked-sequence {
                  seq-local: [w3941 _ _] -> [_ w3943 _]
                  frame #0 {
                    n2273 = call "CALIBRATION PASSWORD"() -> ("PASSWORD"=w3941:string)  [unwired: 17 in, 2 out]
                  }
                  frame #1 {
                    n2274 = Equal?(x=w3943, y="7777") -> (x = y?=w3942:bool)
                    n2275 = case shown="True" w3942 {
                      frame False {
                      }
                      frame True {
                        n2276 = stacked-sequence {
                          frame #0 {
                            n2277 = call "sub vi - calibration v1.vi"() -> ()  [unwired: 12 in]
                          }
                          frame #1 {
                            n2278 = call "sub vi - get calibration values v1.vi"() -> ("LAB01 (CAL)"=w3949:T6, "LAB02 (CAL)"=w3948:T7, "LAB03 (CAL)"=w3947:T6, "LAB04 (CAL)"=w3946:T6, "calibration file error out"=w3950:errorcluster, "LAB05 (CAL)"=w3945:T6)  [unwired: 10 in]
                            n2279 = local write "calibration file error out"(w3950) -> ()
                            n2280 = local write "LAB04 (CAL)"(w3946) -> ()
                            n2281 = local write "LAB05 (CAL)"(w3945) -> ()
                            n2282 = local write "LAB01 (CAL)"(w3949) -> ()
                            n2283 = local write "LAB02 (CAL)"(w3948) -> ()
                            n2284 = local write "LAB03 (CAL)"(w3947) -> ()
                          }
                        }
                      }
                    }
                  }
                  frame #2 {
                    n2285 = local write "CALIBRATE"(FALSE) -> ()
                  }
                }
              }
            }
          }
        }
        n2286 = node-c288() -> ()  [unwired: 1 in, 1 out]
        "loops" <- w33
      }
      n2287 = node-c288(w10) -> ()  [unwired: 1 out]
    }
  }
